vi "CPT Control 12.1.vi"() -> ()   [LabVIEW 2015]
uses:
  <vilib>/Analysis/baseanly.llb/Mean (DBL).vi
  <vilib>/Analysis/baseanly.llb/Normalize Vector.vi
  <vilib>/Utility/file.llb/Read From Spreadsheet File (string).vi
  <vilib>/Utility/file.llb/Write To Spreadsheet File (string).vi
  <vilib>/Utility/file.llb/Write To Spreadsheet File (DBL).vi
  <vilib>/Analysis/2dsp.llb/1D Cross Correlation (DBL).vi
  <vilib>/Utility/file.llb/Read Delimited Spreadsheet (DBL).vi
  <vilib>/Analysis/NI_AALBase.lvlib
  <vilib>/Analysis/NI_AALPro.lvlib
panel:
  out "Waveform Chart":dbl[](graph)
  in  "fre3":dbl
  out "Distance Difference Graph 2":dbl[](graph)
  out "Pore Offset:":dbl
  out "Side Offset:":dbl
  out "Axial Offset:":dbl
  in  "SET Pump Offsets":bool
  in  "Pore Offset SOLL":dbl
  in  "Side Offset Soll":dbl
  in  "Axial Offset Soll":dbl
  out "Stop Distance IS":dbl min=0.0 max=20.0 format="%#_f mm"
  in  "Stop Distance":dbl=20.0 min=0.0 max=20.0 format="%#_g mm"
  out "reset_flag":bool
  out "Time Loop":u32 format="%.0f ms"
  out "Pre-shearing output":dbl
  out "ms Offset":u32
  out "Test Flag":bool
  out "Date/Time:":string
  in  "Notaus":bool
  in  "Settings Tab":T1(tab)
  out "Axial Pressure":T2(graph)
  out "Side Pressure":T2(graph)
  out "Pore Pressure":T2(graph)
  in  "Visualize data":bool
  in  "Set":bool
  in  "maximum acceptable \nSide volume change (ml)":dbl
  in  "SET Pump Pressures":bool
  out "Porepressure":dbl format="%#_4f kPa"
  out "Axialpressure":dbl format="%#_4f kPa"
  out "Sidepressure":dbl format="%#_4f kPa"
  in  "Soll Pore Pressure":dbl min=-200.0 max=4900.0 format="%#_3f kPa"
  in  "Soll Axial Pressure":dbl min=-200.0 max=4000.0 format="%#_3f kPa"
  in  "Soll Side Pressure":dbl min=-200.0 max=4000.0 format="%#_3f kPa"
  in  "Activate Manuel Control":bool
  in  "Schieberegler":dbl(slide) min=-1.0 max=1.0 scale=1.0..-1.0
  out "Position Piston":dbl(slide)
  in  "Move":bool
  out "Contact?":bool
  out "Force Sensor":dbl format="%#_4g N"
  in  "Go - Seitendruck":bool
  in  "Go - Axialdruck":bool
  in  "Velocity Linear":dbl=200.0 format="%#_g kPa/Min"
  in  "Up_Lower":bool
  in  "Delta Pore":dbl format="%#_g kPa"
  in  "GO All Pressure":bool
  in  "Delta Seiten":dbl format="%#_g kPa"
  in  "Delta Axial":dbl format="%#_g kPa"
  in  "Go - Porendruck":bool
  out "Actual side volume change (ml)":sgl format="%.2f"
  out "Velocity deviation":T3(graph)
  out "Acceleration":T3(graph)
  in  "Finish test":bool
  in  "Set file":bool
  in  "Static peneration test":path
  in  "Vibro test 3":path
  in  "Vibro test 1":path
  in  "Static penetration Depth(mm) - 4":dbl
  in  "Time delay - 4":dbl
  in  "Enable Vibro Mode 2":bool
  in  "Enable Vibro Mode 3":bool
  in  "Depth(mm)3":dbl
  in  "Background velocity-3":dbl
  in  "Amplitdue-3":dbl
  in  "freq-3 ( Hz) 2":dbl
  in  "Time delay-3":dbl
  in  "Depth(mm)2":dbl
  in  "Background velocity-2":dbl
  in  "Amplitdue-2":dbl
  in  "freq-2 ( Hz)":dbl
  in  "Switch Vibro Mode":bool
  in  "Control start":bool
  in  "Control Stop":bool
  in  "Activate":bool
  out "Velocity vs Controller output":cluster{dbl[], dbl[]}[](graph)
  out "Correlation curve":dbl[](graph)
  out "time shift steps":sgl format="%.2f"
  in  "Visualize data":bool
  in  "Start Correlation":bool
  out "Intercept b":dbl
  out "Slope m":dbl
  in  "Time delay-2":dbl
  in  "Enable Vibro Mode 1":bool
  in  "Vibration frequency - 1  (Hz)":dbl
  in  "background velocity -1 (mm/s)":dbl
  in  "Amplitude - 1 (mm)":dbl
  in  "Vibro test 2":path
  in  "SET P/I Value":bool
  in  "Set auto file name":bool
  in  "SET Vibro Settings":bool
  out "Vibro Test IS":bool
  out "Frequency IS":dbl min=0.0 max=40.0 format="%#_g Hz"
  out "Amplitude IS":dbl=1.0 min=0.0 max=40.0 format="%#_g mm"
  out "Feeding IS":dbl min=0.0 max=20.0 format="%#_f mm/s"
  in  "New Path":string
  out "Path Logging":path
  in  "Set New Path":bool
  in  "VibroTest":bool=TRUE
  in  "Frequency SOLL":dbl=5.0 min=0.0 max=40.0 format="%#_g Hz"
  in  "Amplitude SOLL":dbl=3.0 min=0.0 max=40.0 format="%#_g mm"
  in  "Vorschub SOLL":dbl=20.0 min=0.0 max=20.0 format="%#_g mm/s"
  in  "Record Data":bool
  out "Record Flag":bool
  in  "start penetration":bool
  out "Boolean":bool
  in  "Soll I-Value":i32 min=-200 max=4000
  in  "Soll P-Value":i32 min=-200 max=4900
  out "IS I-Value":i32
  out "IS P-Value":i32
  out "Axial Pressure okay:":bool
  out "Side Pressure okay:":bool
  out "Pore Pressure okay:":bool
  in  "Circumference Control":bool
  in  "Turn off BC5":bool
  in  "SET Pre-Shearing":bool
  in  "Number of Cycles SOLL":dbl format="%#_f"
  in  "Duration of Cycle SOLL":i32
  in  "Amplitude Cycle SOLL":i32
  in  "Start Pre-Shearing":bool
  out "Pre-Shearing Ended Successful:":bool
  in  "Sollwert Porenwasser":dbl
  in  "Sollwert Seitendruck":dbl
  in  "Huang Su Calibration File":path
  out "IS Parameter 1":dbl=-163.9 format="%#_g x^6 +"
  out "IS Parameter 2":dbl=-163.9 format="%#_g x^5 +"
  out "IS Parameter 3":dbl=-163.9 format="%#_g x^4 +"
  out "IS Parameter 4":dbl=-163.9 format="%#_g x^3 +"
  out "IS Parameter 5":dbl=-163.9 format="%#_g x^2 +"
  out "IS Parameter 6":dbl=-163.9 format="%#_g x     +"
  out "IS Parameter 7":dbl=-163.9
  in  "SET Huang Su":bool
  in  "SOLL Parameter 1":dbl=-163.9 format="%#_g x^6 +"
  in  "SOLL Paramter 2":dbl=-163.9 format="%#_g x^5 +"
  in  "SOLL Parameter 3":dbl=-163.9 format="%#_g x^4 +"
  in  "SOLL Parameter 4":dbl=-163.9 format="%#_g x^3 +"
  in  "SOLL Parameter 5":dbl=-163.9 format="%#_g x^2 +"
  in  "SOLL Parameter 6":dbl=-163.9 format="%#_g x     +"
  in  "SOLL Parameter 7":dbl=-163.9
  out "Piston Position (mm)":dbl[](graph)
  out "Linear calibration":cluster{"array":dbl[], "array":dbl[]}(graph)
  in  "Calibration start":bool
  in  "Soll Slope-Strain":dbl
  in  "Soll Intercept-strain":dbl
  in  "Set button":bool
  out "IS-ADWIN":dbl
  out "IS- ADWIN":dbl
  in  "Initial cone position (mm)":dbl
  in  "Starting penetration depth (mm)  2":dbl
  in  "initial strain r0":dbl
  out "Timer Leackage":dbl format="%#_g s"
  out "Axial Leackage":dbl format="%.2f ml/m"
  out "Side Leackage":dbl format="%.2f ml/m"
  out "Pore Leackage":dbl format="%.2f ml/m"
  in  "Reset Leackage":bool
  out "Axial Kp:":dbl=40.0
  out "Axial Ki:":dbl format="%.2f"
  out "Side Kp:":dbl=40.0
  out "Side Ki:":dbl format="%.2f"
  out "Pore Kp:":dbl=40.0
  out "Pore Ki:":dbl format="%.2f"
  in  "SET Pump Controls":bool
  out "Modus":i32
  in  "Kpa":dbl=40.0
  in  "Kia":dbl=0.2 format="%.1f"
  in  "Kps":dbl=40.0
  in  "Kis":dbl=0.2 format="%.1f"
  in  "Kpp":dbl=40.0
  in  "Kip":dbl=0.2 format="%.1f"
  in  "Set":bool
  out "Side Offset: 2":dbl
  out "Axial Offset: 2":dbl
  out "Pore Offset: 2":dbl
  in  "Axial Offset Soll 2":dbl
  in  "Side Offset Soll 2":dbl
  in  "Pore Offset SOLL 2":dbl
  out "ms Offset Pre-Shearing":u32
  out "Seitendruck save":dbl format="%#.0f"
  out "Axialdruck save":dbl format="%#.0f"
  out "Porendruck save":dbl format="%#.0f"
  in  "View Tab":T4(tab)
  in  "Reset_left_graph":bool
  out "Recording":bool
  out "Cone Pressure":cluster{"mean":dbl, "mean":dbl}(graph)
  out "LVDT 3":dbl format="%0.3f mm"
  out "LVDT 2":dbl format="%0.3f mm"
  out "ml Pore Linear":dbl(slide) scale=0.0..1015.0
  out "ml Side Linear":dbl(slide) scale=0.0..1009.0
  out "ml Axial Linear":dbl(slide) scale=0.0..1014.5
  out "Pore":dbl format="%#_4g ml"
  out "Side":dbl format="%#_4g ml"
  out "Axial":dbl format="%#_4g ml"
  out "Addional Side Pressure":dbl format="%.2f kPa"
  out "Max Expansion":dbl format="%.2f mm"
  out "LVDT 1":dbl format="%0.3f mm"
  in  "Regelung Akiv Axial":bool
  in  "Regelung Akiv Sidepressure":bool
  in  "Regelung Akiv Porepress":bool
  out "Axial Pressure  [KPa]":dbl format="%#.2f kPa"
  out "Side Pressure  [KPa]":dbl format="%#.2f kPa"
  out "Pore Pressure [KPa]":dbl format="%#.2f kPa"
  out "ml Fontpanel":cluster{"mean":dbl, "mean":dbl, "mean":dbl}(graph)
  out "LVDT Frontpannel":cluster{"mean":dbl, "mean":dbl, "mean":dbl}(graph)
  out "Interner Kraftsensor [MPa]":cluster{"Y":dbl[], "Y":dbl[]}[](graph) caption="XY-Graph"
  out "Notaus Activ":bool
  out "Linear Control On":bool
  out "Test Started":bool
  out "Ready":bool
  out "Manuel Control":bool
  out "Pump Control On":bool
  out "Hold Position":bool
  out "Test ended":bool
  out "Penetration ongoing":bool
  out "Cone Tip Resistance":dbl format="%0.2f"
  out "Cone Side Resistance":dbl format="%0.2f"
  in  "Activate Pumps/Piston Controls":bool
  out "Distance Graph":T2(graph)
  out "Linear regression":cluster{dbl[], dbl[]}[](graph)
  out "Controller Output":T2(graph)
  out "Regelung Out":dbl(graph)
  out "Valve Is":dbl(graph)
  out "SOLL IS Distance":cluster{dbl, dbl}(graph)
  in  "Stop/Start":bool
  out "Axialdruck [Pa] 4":dbl(graph)
  out "Seitendruck [Pa] 3":dbl(graph)
  out "Porendruck [Pa] 2":dbl(graph)
  in  "Reset Alarm":bool
  out "Side Alarm":bool
  in  "Erlaubte Max Abweichung Side":dbl
  in  "Erlaubte  Max Abweichung Pore":dbl
  in  "Erlaubte Max Abweichung Axial":dbl
  out "Sollvorgabe":T5(graph)
  out "S":u32
  out "Total Elapsed Seconds":dbl
  out "Alarm Triggered":bool
  out "Abweichung Side":dbl format="%#_4g"
  out "Pore Alarm":bool
  out "Axial Alarm":bool
  out "Abweichung Pore":dbl format="%#_4g"
  out "Abweichung Axial":dbl format="%#_5g"
  # "Activate Manuel Piston Control"
  # "Velocity Piston"
  # "Up"
  # "Down"
  # "IS-ADwin:"
  # "Set Value:"
  # "Pore Pressure:"
  # "Side Pressure"
  # "Axial Pressure"
  # "Linear Pressure Control"
  # "Decreasing"
  # "Increasing"
  # "Delta Pore"
  # "Delta Side"
  # "Delta Axial"
  # "Vibro Settings"
  # "IS-ADwin:"
  # "Set Value:"
  # "Feeding:"
  # "Vibro Test ON:"
  # "Amplitude:"
  # "Frequency:"
  # "Controller Settings"
  # "IS-ADwin:"
  # "Set Value:"
  # "Kp:"
  # "Ki:"
  # "End of Test"
  # "IS-ADwin:"
  # "Set Value:"
  # "IS-ADwin:"
  # "Set Value:"
  # "Leackage Indicator"
  # "IS-ADwin:"
  # "Set Value:"
  # "Control"
  # "Pressure"
  # "reset"
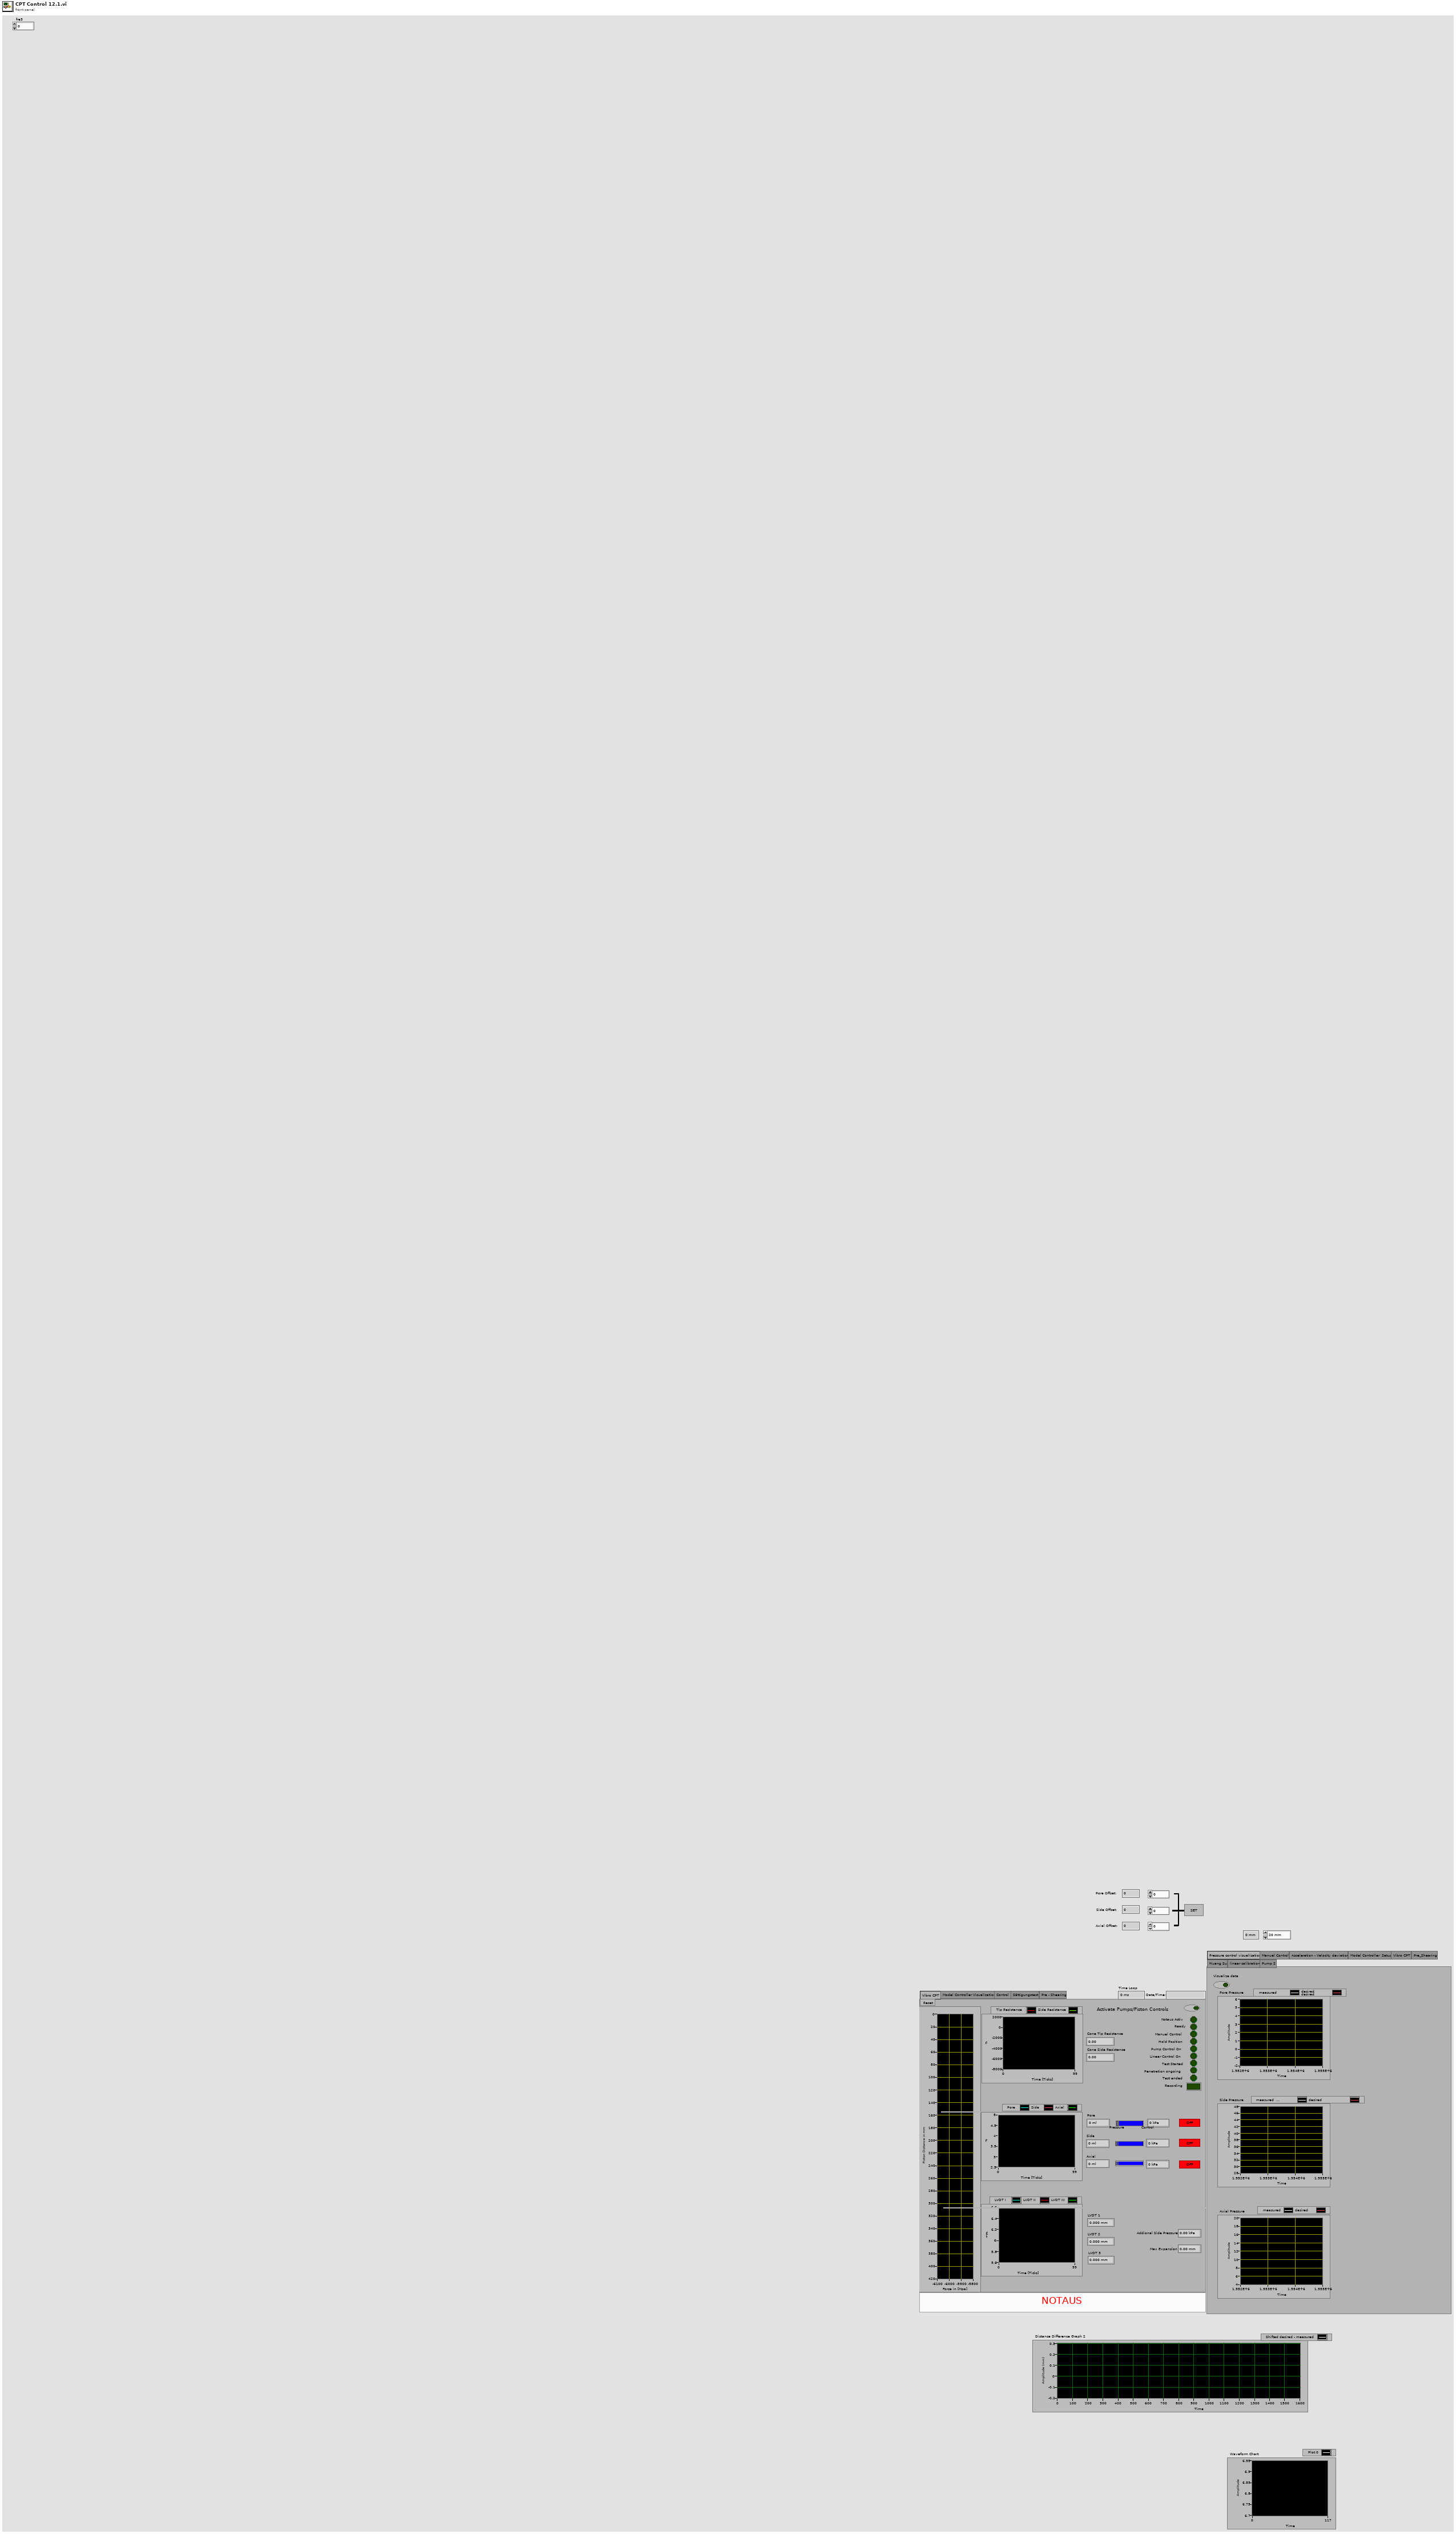
[diagram p1: front panel]
types:
  T1 = enum32{"Pressure control visualization", "Manuel Control", "Acceleration - Velocity deviation", "Model Controller  Setup", "Vibro CPT", "Pre_Shearing", "Huang Su", "linear calibration", "Pump S"}
  T2 = cluster{"Output Array":dbl[], "Output Array":dbl[]}[]
  T3 = cluster{"Output Array":dbl[], "Output Array 2":dbl[]}
  T4 = enum32{"Vibro CPT", "Model Controller Visualization", "Control", "Sättigungstest", "Pre - Shearing"}
  T5 = cluster{"Axial Pressure  [KPa]":dbl, "Pre-shearing output":dbl}
  T6 = enum8{"Enabled", "Disabled", "Disabled and Grayed Out"}
  T7 = enum16{"Program Counter", "Force ", "Position Induktiv", "Position Laser", "Laser 01", "Axial Stellwert", "LVDT 1", "LVDT 2", "LVDT 3", "Pore Pressure", "Side Pressure ", "Axial Pressure", "Pore Volumen", "Side Volumen ", "Axial Volumen ", "NaN", "LVDT Max", "Side Addtional Pressure", "Stellwert Regler", "Cone  Pore Pressure ", "Cone  Side Pressure ", "Valve Kolbenposition", "Regelanweichung", "Regelabweichung Summe ", ""}
  T8 = enum16{"Program Counter", "Force ", "Position Induktiv", "PorePress_regout", "SidePress_regout", "AxialPress_regout", "LVDT 1", "LVDT 2", "LVDT 3", "Pore Pressure", "Side Pressure ", "Axial Pressure", "Pore Volumen", "Side Volumen ", "Axial Volumen ", "Soll_Porepress", "Soll_Sidepress", "Soll_axialpress", "LVDT_max", "desired distance", "predict distance", "fitted velocity", "Valve IST", "Tip resistance", "Pore pressure", "Distance_Regout", "velocity data", "estimated_Distance_Regout", "normalize vel", "normalize Distance_regout", "strain", "additional side pressure", "initial_depth", "Distance_digital", "initial volume", "actual volume", "actual side volume"}
  T9 = enum16{"NaN", "WegInd_Digits", "Valve_IST", "KraftHTM_Digits", "WegInd_Delta", "WegLaser_Digits", "Laser_O1", "Laser_M3", "LVDT_2", "LVDT_3", "LVDT_1", "PorePress_Digits", "AxialPress_Digits", "SidePress_Digits", "SpindelA_Digits", "SpindelB_Digits", "SpindelC_Digits", "FPAR_17", "Slope_calibration", "Intercept_calibration", "PorePressOffset", "AxialPressOffset", "SidePressOffset", "FPAR_23", "FPAR_24", "Vorschub", "Sinusfrequenz_Vibro", "Amplitude_Vibro", "PreShearingOutput", "FPAR_29", "FPAR_30", "FPAR_31", "FPAR_32", "FPAR_33", "FPAR_34", "FPAR_35", "FPAR_36", "FPAR_37", "FPAR_38", "FPAR_39", "Kp_Porepress", "Ki_Porepress", "Kp_Sidepress", "Ki_Sidepress", "Kp_Axialpress", "Ki_Axialpress", "FPAR_46", "FPAR_47", "FPAR_48", "FPAR_49", "FPAR_50", "PaProMin", "FPAR_52", "FPAR_53", "FPAR_54", "Huang_Su_par_1", "Huang_Su_par_2", "Huang_Su_par_3", "Huang_Su_par_4", "Huang_Su_par_5", "FPAR_60", "FPAR_61", "Huang_Su_par_6", "Huang_Su_par_7", "FPAR_64", "FPAR_65", "FPAR_66", "Model_PreShearing", "Model_Vibro", "FPAR_69", "FPAR_70", "FPAR_71", "Set_Soll_PorePressure", "Set_Soll_AxialPressure", "Set_Soll_SidePressure", "Soll_PorePressure", "Soll_AxialPressure", "Soll_SidePressure", "Taktzeit", "Abtastfrequenz", "Clock"}
  T10 = enum16{"NaN", "WegInd_Digits", "Valve_IST", "KraftHTM_Digits", "WegInd_Delta", "WegLaser_Digits", "Laser_O1", "Laser_M3", "LVDT_2", "LVDT_3", "LVDT_1", "PorePress_Digits", "AxialPress_Digits", "SidePress_Digits", "SpindelA_Digits", "SpindelB_Digits", "SpindelC_Digits", "FPAR_17", "FPAR_18", "FPAR_19", "PorePressOffset", "AxialPressOffset", "SidePressOffset", "FPAR_23", "FPAR_24", "Vorschub", "Sinusfrequenz_Vibro", "Amplitude_Vibro", "PreShearingOutput", "FPAR_29", "FPAR_30", "FPAR_31", "FPAR_32", "FPAR_33", "FPAR_34", "FPAR_35", "FPAR_36", "FPAR_37", "FPAR_38", "FPAR_39", "Kp_Porepress", "Ki_Porepress", "Kp_Sidepress", "Ki_Sidepress", "Kp_Axialpress", "Ki_Axialpress", "FPAR_46", "FPAR_47", "FPAR_48", "FPAR_49", "FPAR_50", "PaProMin", "FPAR_52", "FPAR_53", "FPAR_54", "Huang_Su_par_1", "Huang_Su_par_2", "Huang_Su_par_3", "Huang_Su_par_4", "Huang_Su_par_5", "FPAR_60", "FPAR_61", "Huang_Su_par_6", "Huang_Su_par_7", "FPAR_64", "FPAR_65", "FPAR_66", "Model_PreShearing", "Model_Vibro", "FPAR_69", "FPAR_70", "FPAR_71", "Set_Soll_PorePressure", "Set_Soll_AxialPressure", "Set_Soll_SidePressure", "Soll_PorePressure", "Soll_AxialPressure", "Soll_SidePressure", "Taktzeit", "Abtastfrequenz", "Clock"}
  T11 = cluster{"Output Array":dbl[], "Output Array":dbl[]}
  T12 = cluster{"Output Array":dbl[], "normalized waveform":waveform(dbl)}
  T13 = cluster{"Output Array":dbl[], "normalized waveform":waveform(dbl)}[]
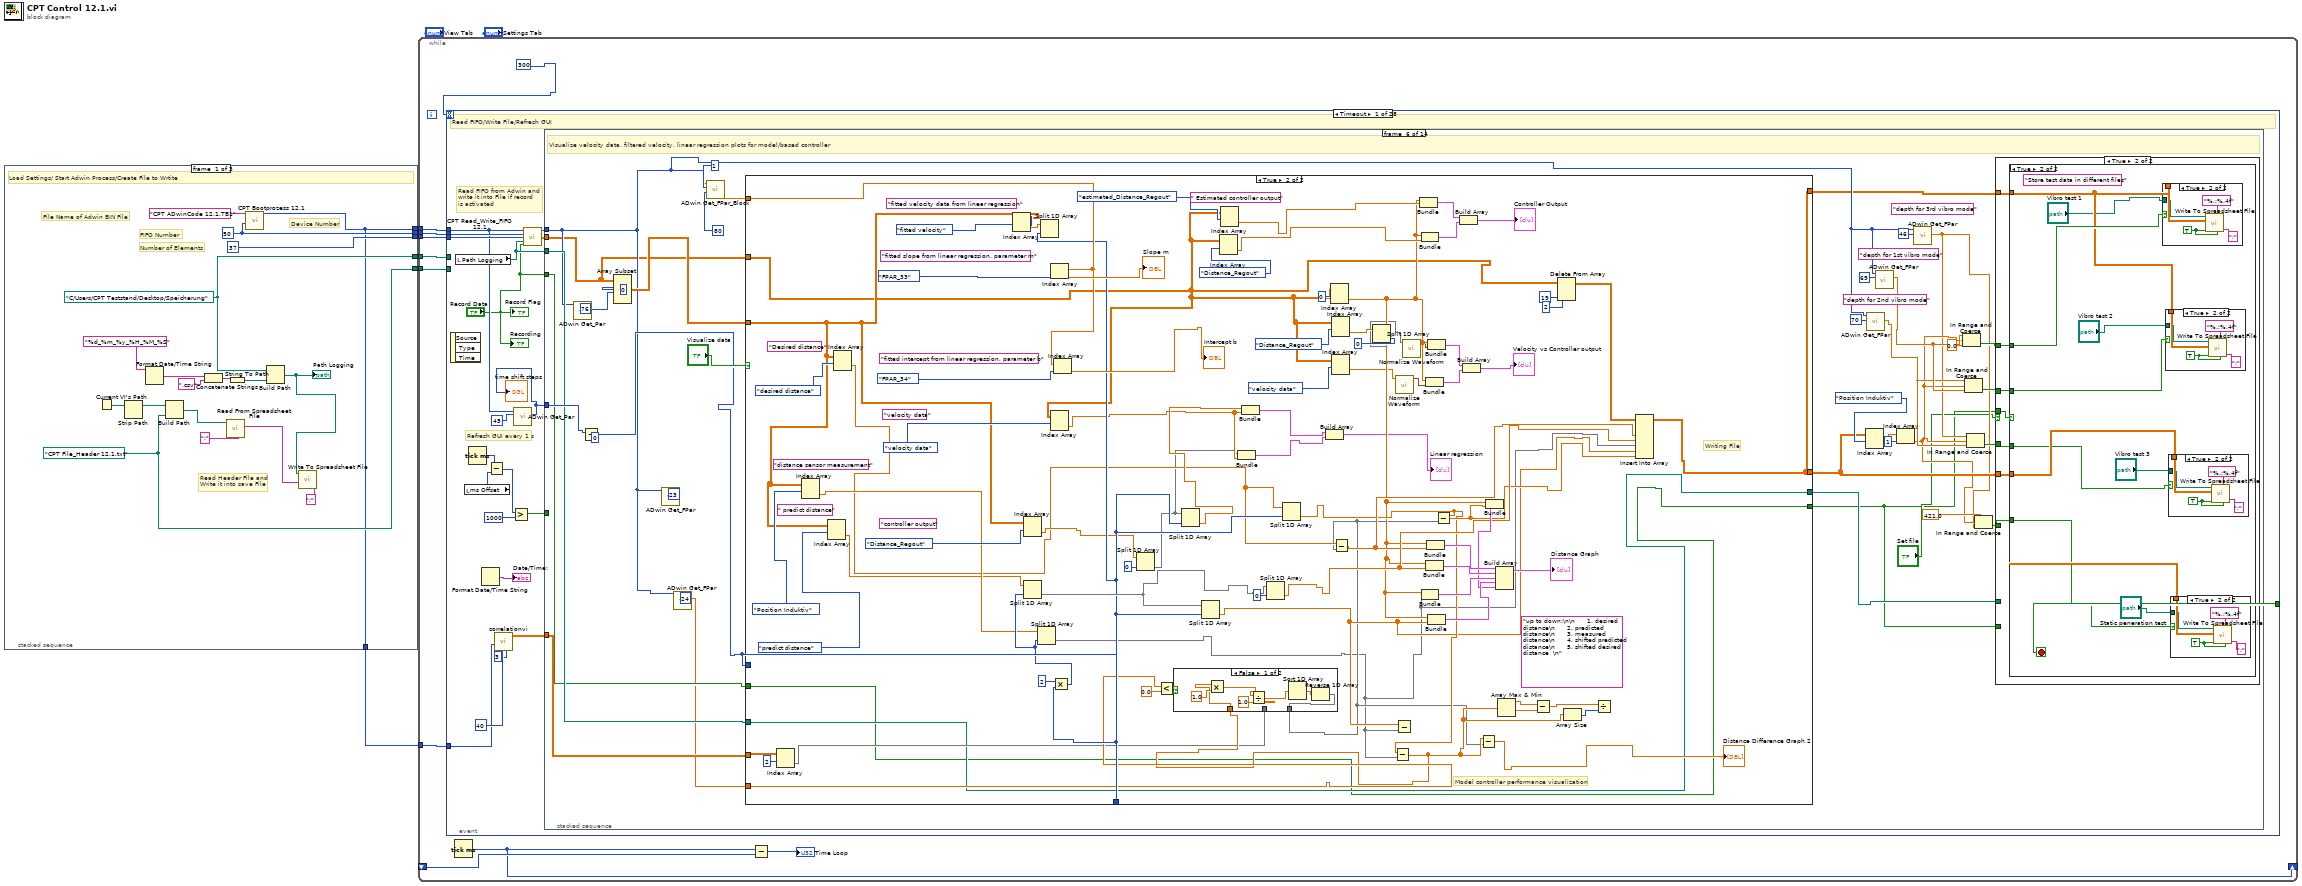
[diagram p0: block diagram]
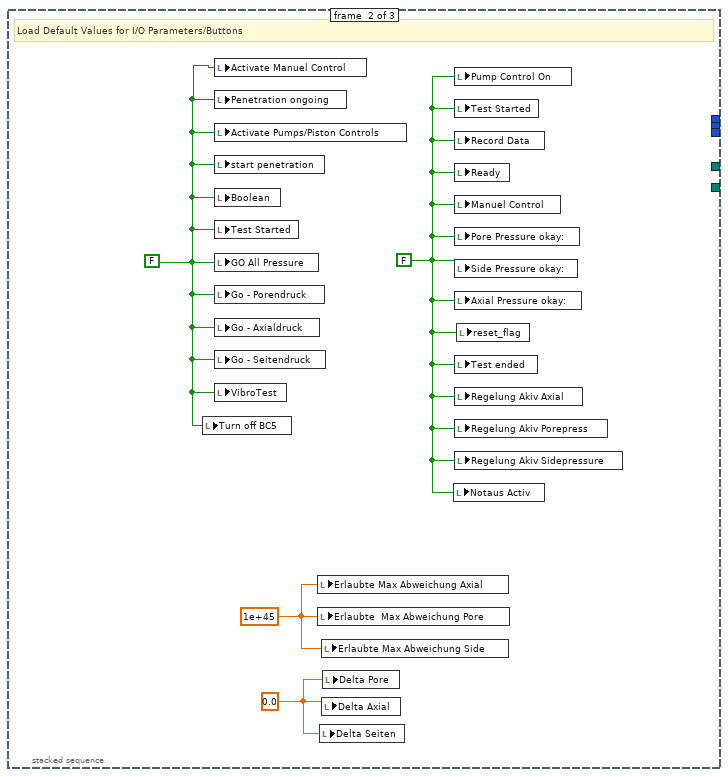
[diagram p2: hidden frame]
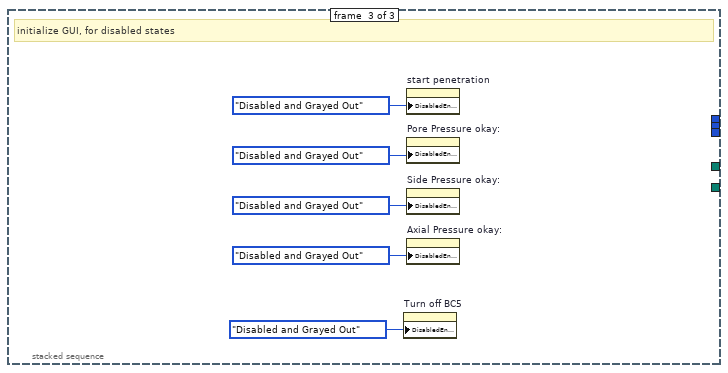
[diagram p3: hidden frame]
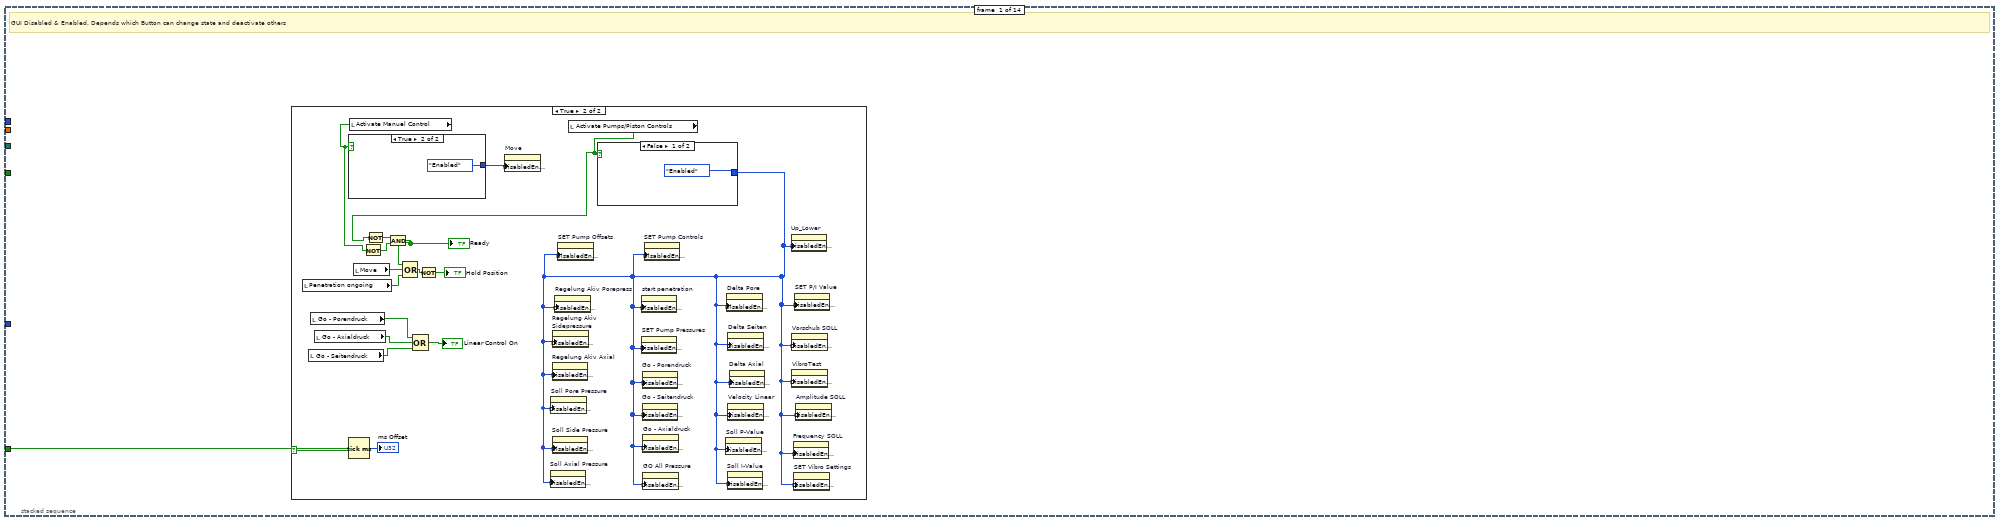
[diagram p4: hidden frame]
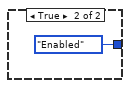
[diagram p6: hidden frame]
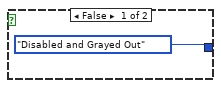
[diagram p7: hidden frame]
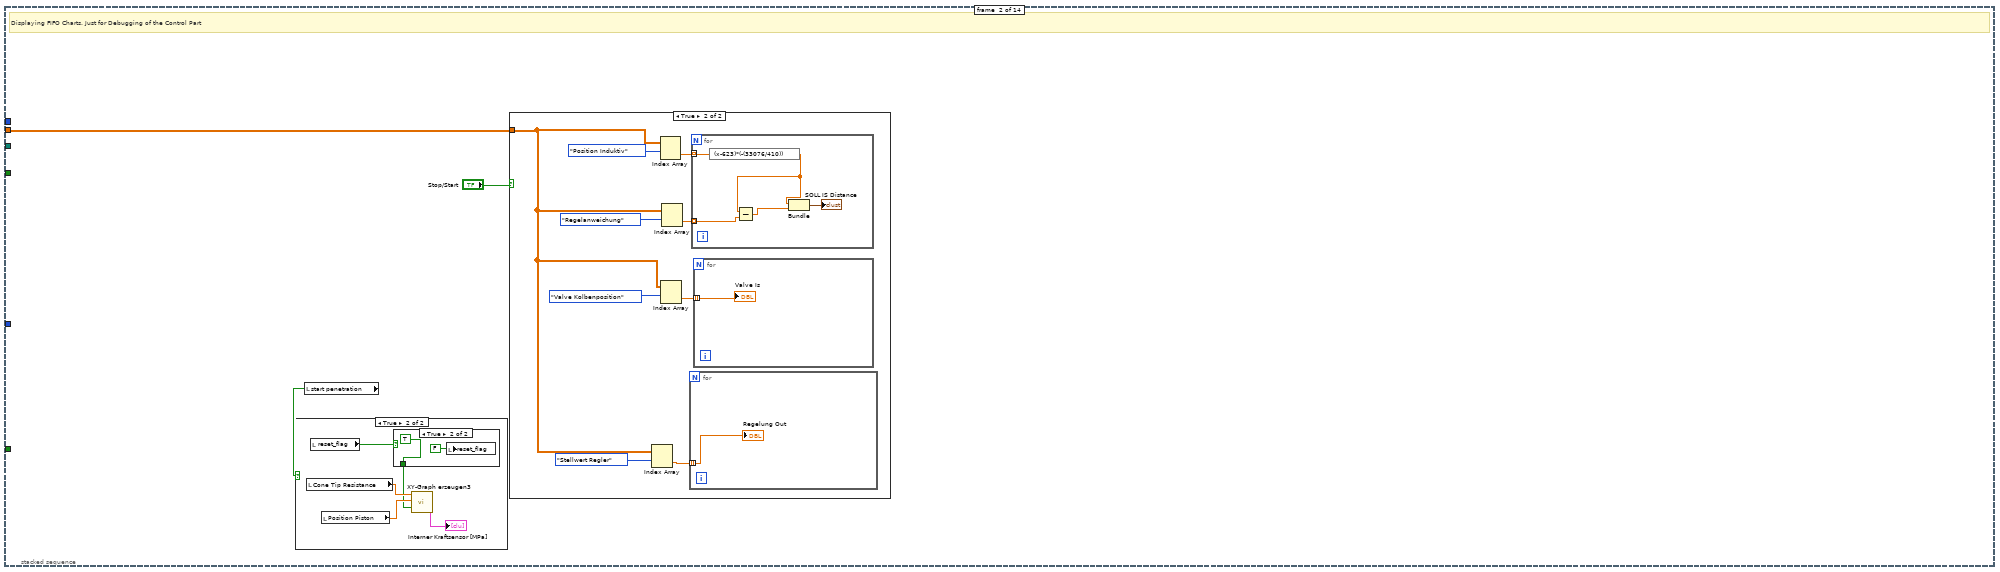
[diagram p8: hidden frame]
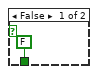
[diagram p10: hidden frame]
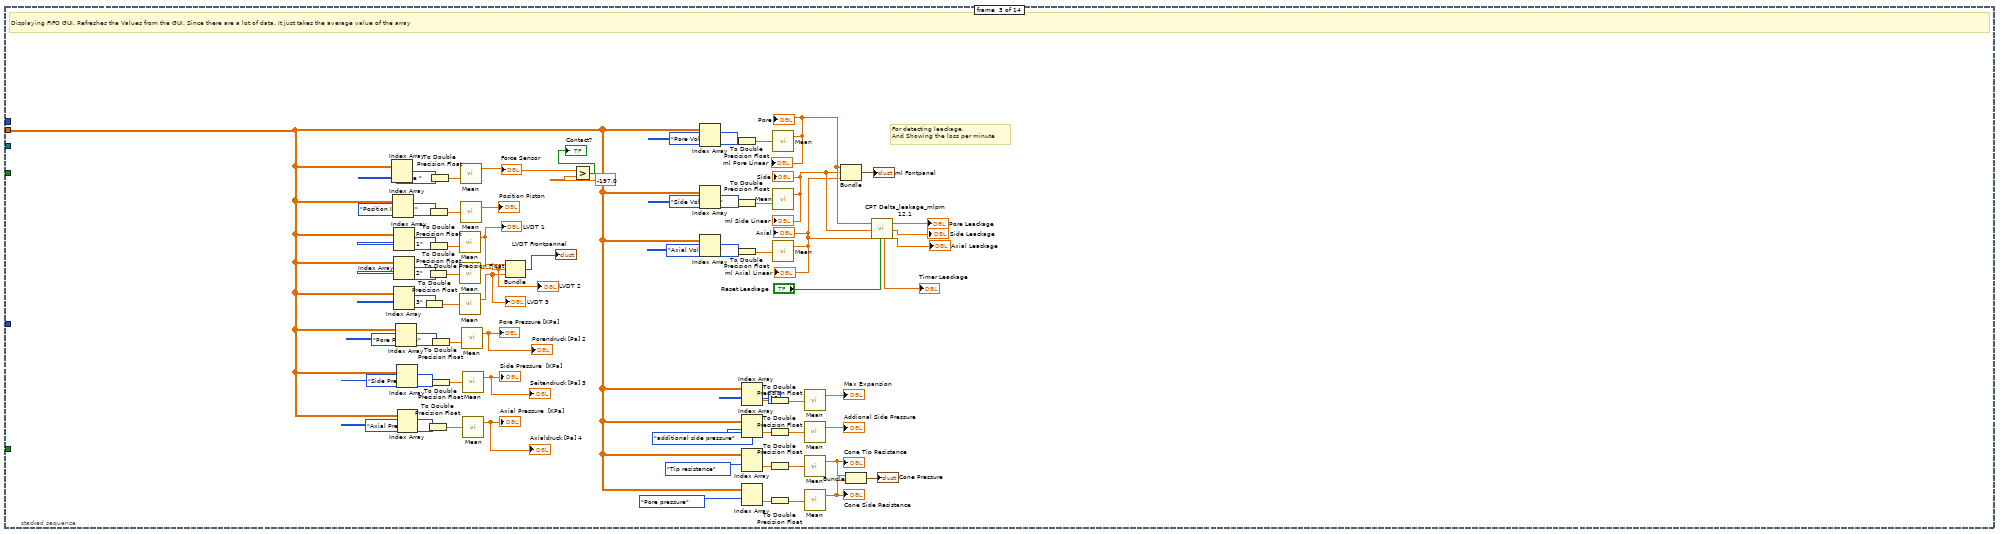
[diagram p12: hidden frame]
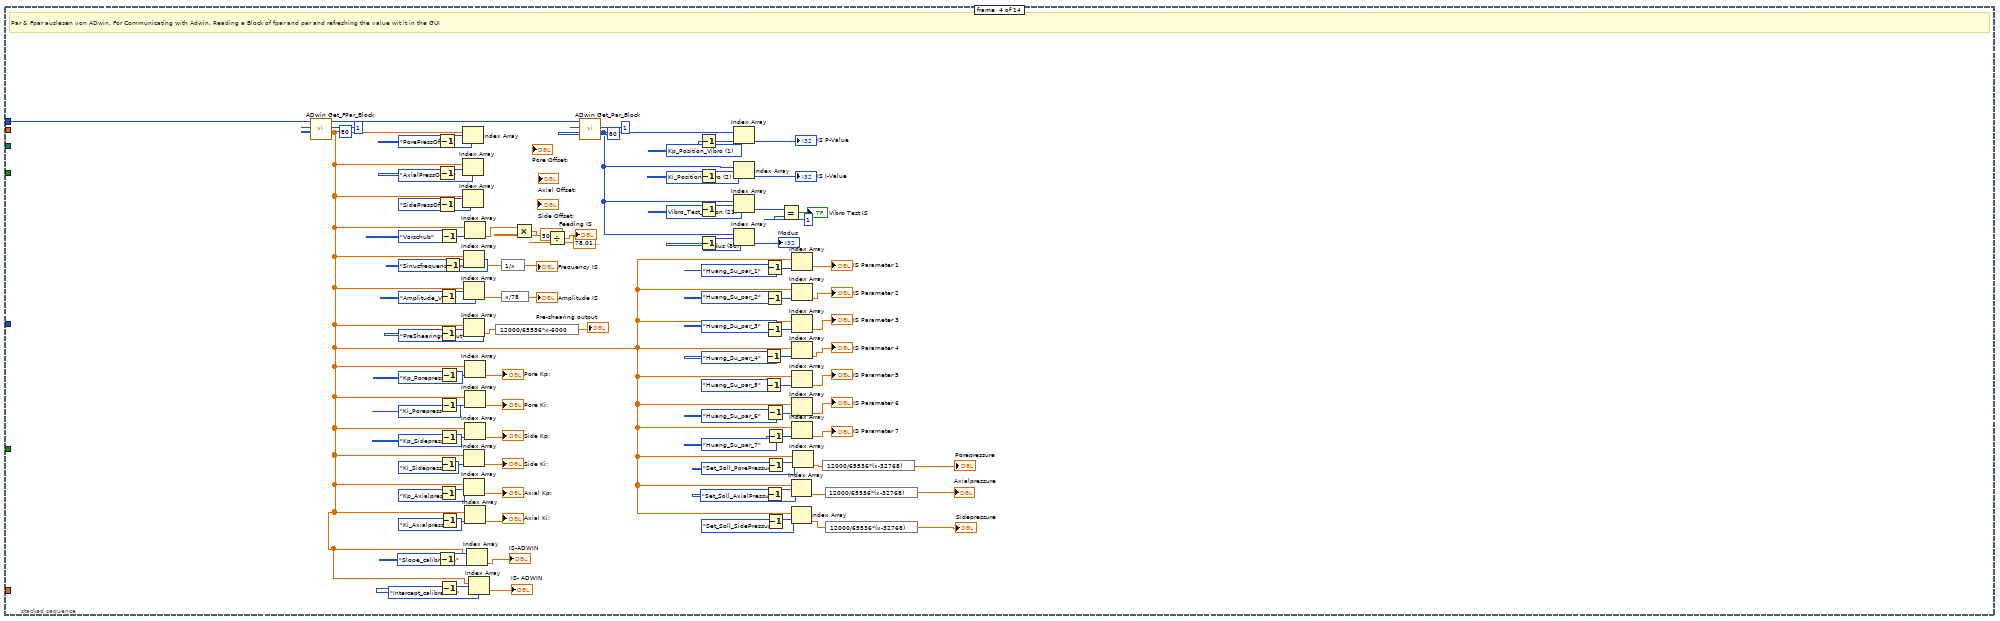
[diagram p13: hidden frame]
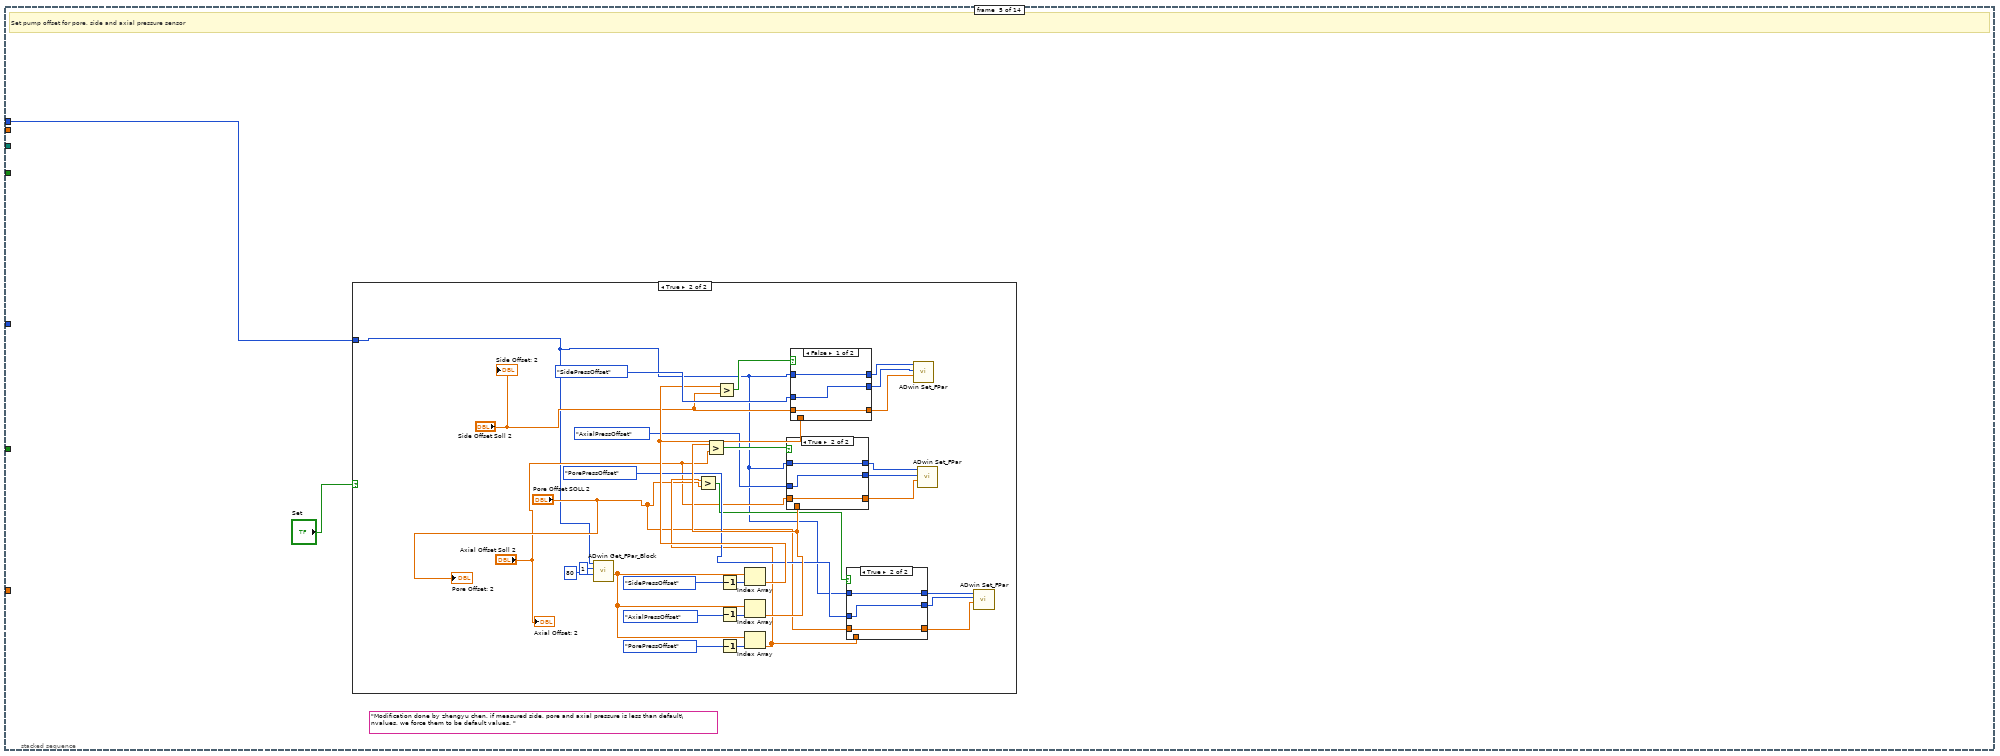
[diagram p14: hidden frame]
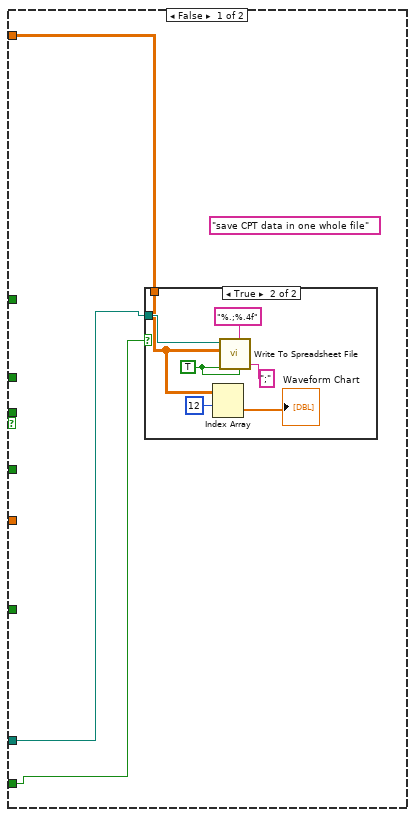
[diagram p19: hidden frame]
diagram:
  n1 = stacked-sequence {
    tunnel: [w7 _ _] -> w6
    tunnel: [w24 _ _] -> w5
    tunnel: [37 ("dimension size") _ _] -> w4
    tunnel: [w11 _ _] -> w3
    tunnel: [w9 _ _] -> w2
    tunnel: [w7 _ _] -> w1
    frame #0 {
      w9 = path "CPT File_Header 12.1.txt" ("Grundpfad")
      w24 = u16 50 ("FifoNo")
      w11 = path "C:/Users/CPT Teststand/Desktop/Speicherung" ("Grundpfad")
      # "Read Header File and \nWrite it into save File"
      # "File Name of Adwin BIN File"
      # "Device Number"
      # "Number of Elements"
      # "FIFO Number"
      # "Load Settings/ Start Adwin Process/Create File to Wrtite"
      n2 = Current VI's Path() -> (path=w14:path)
      n3 = Strip Path(path=w14) -> (stripped path=w13:path)  [unwired: 1 out]
      n4 = Format Date/Time String(time format string (%c)="%d_%m_%y_%H_%M_%S") -> (date/time string=w18:string)  [unwired: 2 in]
      n5 = Build Path(base path=w13, name or relative path=w9) -> (appended path=w15:path)
      n6 = Concatenate Strings(w18, ".csv" ("String")) -> (w21:string)
      n7 = call-poly <vilib>:"Read From Spreadsheet File.vi"("delimiter (\\t)"=";" ("delimiter (\\t)"), "file path (dialog if empty)"=w15) -> ("first row"=w16:string[])  [unwired: 5 in, 4 out]
      n8 = String To Path(string=w21) -> (path=w20:path)
      n9 = call "CPT Bootprozess 12.1.vi"("FifoNo"=w24, "Boot File Relative Referenz"="CPT ADwinCode 12.1.TB1" ("Filename")) -> ("Device No. out"=w7:u16)  [unwired: 8 in, 1 out]
      n10 = Build Path(base path=w11, name or relative path=w20) -> (appended path=w8:path)
      "Path Logging" <- w8
      n11 = call-poly <vilib>:"Write To Spreadsheet File.vi"("delimiter (\\t)"=";" ("delimiter (\\t)"), "1D data"=w16, "file path (dialog if empty)"=w8) -> ()  [unwired: 5 in, 1 out]
    }
    frame #1 {
      w26 = 1e+45 ("Abweichung Solll  - Ist")
      w27 = 0.0 ("Delta Pore")
      w28 = FALSE ("Boolean")
      w25 = FALSE ("Freeze")
      # "Load Default Values for I/O Parameters/Buttons"
      n12 = local write "Turn off BC5"(w28) -> ()
      n13 = local write "Activate Manuel Control"(w28) -> ()
      n14 = local write "Penetration ongoing"(w28) -> ()
      n15 = local write "Activate Pumps/Piston Controls"(w28) -> ()
      n16 = local write "start penetration"(w28) -> ()
      n17 = local write "Boolean"(w28) -> ()
      n18 = local write "Test Started"(w28) -> ()
      n19 = local write "GO All Pressure"(w28) -> ()
      n20 = local write "Go - Porendruck"(w28) -> ()
      n21 = local write "Go - Axialdruck"(w28) -> ()
      n22 = local write "Go - Seitendruck"(w28) -> ()
      n23 = local write "VibroTest"(w28) -> ()
      n24 = local write "Erlaubte Max Abweichung Axial"(w26) -> ()
      n25 = local write "Erlaubte  Max Abweichung Pore"(w26) -> ()
      n26 = local write "Delta Seiten"(w27) -> ()
      n27 = local write "Erlaubte Max Abweichung Side"(w26) -> ()
      n28 = local write "Delta Axial"(w27) -> ()
      n29 = local write "Delta Pore"(w27) -> ()
      n30 = local write "Notaus Activ"(w25) -> ()
      n31 = local write "Pump Control On"(w25) -> ()
      n32 = local write "Test Started"(w25) -> ()
      n33 = local write "Record Data"(w25) -> ()
      n34 = local write "Ready"(w25) -> ()
      n35 = local write "Manuel Control"(w25) -> ()
      n36 = local write "Pore Pressure okay:"(w25) -> ()
      n37 = local write "Side Pressure okay:"(w25) -> ()
      n38 = local write "Axial Pressure okay:"(w25) -> ()
      n39 = local write "Test ended"(w25) -> ()
      n40 = local write "Regelung Akiv Axial"(w25) -> ()
      n41 = local write "Regelung Akiv Porepress"(w25) -> ()
      n42 = local write "Regelung Akiv Sidepressure"(w25) -> ()
      n43 = local write "reset_flag"(w25) -> ()
    }
    frame #2 {
      # "initialize GUI, for disabled states"
      n44 = property on="Turn off BC5" class="Bool (strict)"("DisabledEnum"=T6."Disabled and Grayed Out" ("Disabled")) -> ()  [unwired: 2 in, 2 out]
      n45 = property on="start penetration" class="Bool (strict)"("DisabledEnum"=T6."Disabled and Grayed Out" ("Disabled")) -> ()  [unwired: 2 in, 2 out]
      n46 = property on="Pore Pressure okay:" class="Bool (strict)"("DisabledEnum"=T6."Disabled and Grayed Out" ("Disabled")) -> ()  [unwired: 2 in, 2 out]
      n47 = property on="Side Pressure okay:" class="Bool (strict)"("DisabledEnum"=T6."Disabled and Grayed Out" ("Disabled")) -> ()  [unwired: 2 in, 2 out]
      n48 = property on="Axial Pressure okay:" class="Bool (strict)"("DisabledEnum"=T6."Disabled and Grayed Out" ("Disabled")) -> ()  [unwired: 2 in, 2 out]
    }
  }
  n49 = while {
    tunnel: w6 -> [w35]
    shift-right: [w42] -> _
    shift-left: _ -> [w44]
    tunnel: w5 -> [w41]
    tunnel: w4 -> [w40]
    tunnel: w3 -> [w39]
    tunnel: w2 -> [w37]
    tunnel: w1 -> [w36]
    stop <- w38 stop-if-true
    n50 = event shown="[0] Timeout" {
      selector: _ -> [_ _ _ _ _ _ _ _ _ _ _ _ _ _ _ _ _ _ _ _ _ _ _ _ _ _ _ _]
      dyn-events: _ -> [_ _ _ _ _ _ _ _ _ _ _ _ _ _ _ _ _ _ _ _ _ _ _ _ _ _ _ _]
      timeout: 300 -> [_ _ _ _ _ _ _ _ _ _ _ _ _ _ _ _ _ _ _ _ _ _ _ _ _ _ _ _]
      tunnel: w35 -> [w52 _ w928 w934 w986 w999 w1004 w1013 w1020 _ w1073 w1109 w1120 _ w1194 _ w1221 w1229 w1243 w1247 w1257 w1267 w1275 w1292 w1332 w1355 w1365 w1410]
      tunnel: w41 -> [w63 _ _ _ _ _ _ _ _ _ _ _ _ _ _ _ _ _ _ _ _ _ _ _ _ _ _ _]
      tunnel: w40 -> [w62 _ _ _ _ _ _ _ _ _ _ _ _ _ _ _ _ _ _ _ _ _ _ _ _ _ _ _]
      tunnel: w39 -> [_ _ _ _ _ _ _ _ _ _ _ _ _ w1164 _ w1203 _ _ _ _ _ _ _ _ _ _ _ _]
      tunnel: [_ _ w930 _ _ _ _ _ _ _ _ _ _ _ _ _ _ _ _ _ _ _ _ _ _ _ _ _] -> w38
      tunnel: w37 -> [_ _ _ _ _ _ _ _ _ _ _ _ _ w1156 _ w1196 _ _ _ _ _ _ _ _ _ _ _ _]
      tunnel: w36 -> [w47 _ _ _ _ _ _ _ _ _ _ _ _ _ _ _ _ _ _ _ _ _ _ _ _ _ _ _]
      event Timeout {
        # "Read FIFO from Adwin and \nwrite it into File if record \nis activated"
        # "Refresh GUI every 1 s"
        # "Read FIFO/Write File/Refresh GUI"
        n51 = event-data() -> ()  [unwired: 1 in, 3 out]
        n52 = local read "Path Logging"() -> (w46:path)
        n53 = local read "ms Offset"() -> (w59:u32)
        n54 = Tick Count (ms)() -> (millisecond timer value=w58:u32)
        n55 = Format Date/Time String() -> (date/time string=→"Date/Time:":string)  [unwired: 3 in]
        n56 = Subtract(x=w58, y=w59) -> (x-y=w56:u32)
        n57 = call "correlationvi.vi"("Number of Elements"=3, "FifoNo"=i16 40, "Device No."=w47) -> ("Output Array 2"=w48:dbl[][])  [unwired: 6 in, 2 out]
        n58 = Greater?(x=w56, y=u32 1000) -> (0:w57:bool)
        n59 = call "ADwin Get_Par.vi"("index"=u16 45 ("Device No. out"), "Device No. (1)"=w52) -> ("ParameterValue"=w51:i32)  [unwired: 7 in, 2 out]
        "time shift steps" <- w51
        n60 = call "CPT Read_Write_FIFO 12.1.vi"("Device No."=w52, "FifoNo"=w63, "Number of Elements"=w62, "Path Logging"=w46, "Record"="Record Data") -> ("Device No. out"=w60:u16, "Output Array"=w61:dbl[][])  [unwired: 9 in]
        n61 = stacked-sequence {
          tunnel: w61 -> [_ w87 w127 _ _ w338 w524 w577 w617 _ w739 _ _ _]
          tunnel: w60 -> [_ _ _ w273 w287 w353 w522 _ w610 w734 w742 w766 _ w900]
          tunnel: w57 -> [w64 _ _ _ _ _ _ _ _ _ _ _ _ _]
          tunnel: w51 -> [_ _ _ _ _ w368 _ _ w616 _ _ _ _ _]
          tunnel: w48 -> [_ _ _ _ _ w363 w528 _ _ _ _ _ _ _]
          tunnel: w46 -> [_ _ _ _ _ w366 _ _ _ _ _ _ _ _]
          tunnel: "Record Data" -> [_ _ _ _ _ w365 _ _ _ _ _ _ _ _]
          frame #0 {
            # "GUI Disabled & Enabled. Depends which Button can change state and deactivate others"
            n62 = case shown="True" w64 {
              frame False {
              }
              frame True {
                n63 = local read "Penetration ongoing"() -> (w77:bool)
                n64 = local read "Go - Seitendruck"() -> (w73:bool)
                n65 = local read "Go - Porendruck"() -> (w71:bool)
                n66 = local read "Go - Axialdruck"() -> (w72:bool)
                n67 = Tick Count (ms)() -> (millisecond timer value=→"ms Offset":u32)
                n68 = local read "Activate Manuel Control"() -> (w69:bool)
                n69 = case shown="True" w69 {
                  tunnel: [T6."Disabled and Grayed Out" ("Disabled") T6."Enabled" ("Disabled")] -> w80
                  frame False {
                  }
                  frame True {
                  }
                }
                n70 = local read "Move"() -> (w78:bool)
                n71 = Not(x=w69) -> (.not. x?=w67:bool)
                n72 = Compound Arithmetic op=OR(w71, w72, w73) -> (→"Linear Control On":bool)
                n73 = property on="Move" class="Bool (strict)"("DisabledEnum"=w80) -> ()  [unwired: 2 in, 2 out]
                n74 = local read "Activate Pumps/Piston Controls"() -> (w70:bool)
                n75 = Not(x=w70) -> (.not. x?=w68:bool)
                n76 = And(x=w68, y=w67) -> (x .and. y?=w66:bool)
                "Ready" <- w66
                n77 = Compound Arithmetic op=OR(w66, w78, w77) -> (w76:bool)
                n78 = Not(x=w76) -> (.not. x?=→"Hold Position":bool)
                n79 = case shown="False" w70 {
                  tunnel: [T6."Enabled" ("Disabled") T6."Enabled" ("Disabled")] -> w65
                  frame False {
                  }
                  frame True {
                  }
                }
                n80 = property on="Soll Axial Pressure" class="DigNum (strict)"("DisabledEnum"=w65) -> ()  [unwired: 2 in, 2 out]
                n81 = property on="Soll Pore Pressure" class="DigNum (strict)"("DisabledEnum"=w65) -> ()  [unwired: 2 in, 2 out]
                n82 = property on="Regelung Akiv Axial" class="Bool (strict)"("DisabledEnum"=w65) -> ()  [unwired: 2 in, 2 out]
                n83 = property on="Soll Side Pressure" class="DigNum (strict)"("DisabledEnum"=w65) -> ()  [unwired: 2 in, 2 out]
                n84 = property on="Regelung Akiv Sidepressure" class="Bool (strict)"("DisabledEnum"=w65) -> ()  [unwired: 2 in, 2 out]
                n85 = property on="Regelung Akiv Porepress" class="Bool (strict)"("DisabledEnum"=w65) -> ()  [unwired: 2 in, 2 out]
                n86 = property on="SET Pump Offsets" class="Bool"("DisabledEnum"=w65) -> ()  [unwired: 2 in, 2 out]
                n87 = property on="start penetration" class="Bool (strict)"("DisabledEnum"=w65) -> ()  [unwired: 2 in, 2 out]
                n88 = property on="SET Pump Pressures" class="Bool"("DisabledEnum"=w65) -> ()  [unwired: 2 in, 2 out]
                n89 = property on="Go - Porendruck" class="Bool (strict)"("DisabledEnum"=w65) -> ()  [unwired: 2 in, 2 out]
                n90 = property on="Go - Seitendruck" class="Bool (strict)"("DisabledEnum"=w65) -> ()  [unwired: 2 in, 2 out]
                n91 = property on="Go - Axialdruck" class="Bool (strict)"("DisabledEnum"=w65) -> ()  [unwired: 2 in, 2 out]
                n92 = property on="GO All Pressure" class="Bool (strict)"("DisabledEnum"=w65) -> ()  [unwired: 2 in, 2 out]
                n93 = property on="SET Pump Controls" class="Bool"("DisabledEnum"=w65) -> ()  [unwired: 2 in, 2 out]
                n94 = property on="Soll P-Value" class="DigNum (strict)"("DisabledEnum"=w65) -> ()  [unwired: 2 in, 2 out]
                n95 = property on="Delta Pore" class="DigNum (strict)"("DisabledEnum"=w65) -> ()  [unwired: 2 in, 2 out]
                n96 = property on="Soll I-Value" class="DigNum (strict)"("DisabledEnum"=w65) -> ()  [unwired: 2 in, 2 out]
                n97 = property on="Delta Seiten" class="DigNum (strict)"("DisabledEnum"=w65) -> ()  [unwired: 2 in, 2 out]
                n98 = property on="Velocity Linear" class="DigNum (strict)"("DisabledEnum"=w65) -> ()  [unwired: 2 in, 2 out]
                n99 = property on="Delta Axial" class="DigNum (strict)"("DisabledEnum"=w65) -> ()  [unwired: 2 in, 2 out]
                n100 = property on="Up_Lower" class="Bool (strict)"("DisabledEnum"=w65) -> ()  [unwired: 2 in, 2 out]
                n101 = property on="Vorschub SOLL" class="DigNum (strict)"("DisabledEnum"=w65) -> ()  [unwired: 2 in, 2 out]
                n102 = property on="VibroTest" class="Bool (strict)"("DisabledEnum"=w65) -> ()  [unwired: 2 in, 2 out]
                n103 = property on="Frequency SOLL" class="DigNum (strict)"("DisabledEnum"=w65) -> ()  [unwired: 2 in, 2 out]
                n104 = property on="SET Vibro Settings" class="Bool"("DisabledEnum"=w65) -> ()  [unwired: 2 in, 2 out]
                n105 = property on="SET P/I Value" class="Bool"("DisabledEnum"=w65) -> ()  [unwired: 2 in, 2 out]
                n106 = property on="Amplitude SOLL" class="DigNum (strict)"("DisabledEnum"=w65) -> ()  [unwired: 2 in, 2 out]
              }
            }
          }
          frame #1 {
            # "Displaying FIFO Charts. Just for Debugging of the Control Part"
            n107 = local read "start penetration"() -> (w85:bool)
            n108 = case shown="True" w85 {
              frame False {
              }
              frame True {
                n109 = local read "Cone Tip Resistance"() -> (w90:dbl)
                n110 = local read "reset_flag"() -> (w89:bool)
                n111 = local read "Position Piston"() -> (w91:dbl)
                n112 = case shown="True" w89 {
                  tunnel: [FALSE ("Reset") TRUE ("Reset")] -> w88
                  frame False {
                  }
                  frame True {
                    n113 = local write "reset_flag"(FALSE ("reset_flag")) -> ()
                  }
                }
                n114 = call "XY-Graph erzeugen3"("Reset"=w88, "Y Input"=w91, "X Input"=w90) -> ("XY Graph"=→"Interner Kraftsensor [MPa]":cluster{"Y":dbl[], "Y":dbl[]}[])  [unwired: 7 in, 1 out]
              }
            }
            n115 = case shown="True" "Stop/Start" {
              tunnel: w87 -> [_ w101]
              frame False {
              }
              frame True {
                n116 = Index Array(array=w101, index (row)=T7."Stellwert Regler" ("Enum")) -> (element=w96:dbl[])  [unwired: 1 in]
                n117 = Index Array(array=w101, index (row)=T7."Position Induktiv" ("Enum")) -> (element=w104:dbl[])  [unwired: 1 in]
                n118 = Index Array(array=w101, index (row)=T7."Valve Kolbenposition" ("Enum")) -> (element=w102:dbl[])  [unwired: 1 in]
                n119 = Index Array(array=w101, index (row)=T7."Regelanweichung" ("Enum")) -> (element=w103:dbl[])  [unwired: 1 in]
                n120 = for {
                  tunnel: w96 -> [w105] mode=indexing
                  "Regelung Out" <- w105
                }
                n121 = for {
                  tunnel: w104 -> [w110] mode=indexing
                  tunnel: w103 -> [w107] mode=indexing
                  n122 = expression code="(x-623)*(-(33076/410))"(w110) -> (w109:dbl)
                  n123 = Subtract(x=w109, y=w107) -> (x-y=w108:dbl)
                  n124 = Bundle(w109, w108) -> (→"SOLL IS Distance":cluster{dbl, dbl})  [unwired: 1 in]
                }
                n125 = for {
                  tunnel: w102 -> [w106] mode=indexing
                  "Valve Is" <- w106
                }
              }
            }
          }
          frame #2 {
            # "For detecting leackage. \nAnd Showing the loss per minute"
            # "Displaying FIFO GUI. Refreshes the Values from the GUI. Since there are a lot of data. It just takes the average value of the array"
            n126 = Index Array(array=w127, index (row)=T7."Force " ("Enum")) -> (element=w173:dbl[])  [unwired: 1 in]
            n127 = Index Array(array=w127, index (row)=T7."Position Induktiv" ("Enum")) -> (element=w174:dbl[])  [unwired: 1 in]
            n128 = Index Array(array=w127, index (row)=T7."LVDT 1" ("Enum")) -> (element=w179:dbl[])  [unwired: 1 in]
            n129 = Index Array(array=w127, index (row)=T7."LVDT 2" ("Enum")) -> (element=w180:dbl[])  [unwired: 1 in]
            n130 = Index Array(array=w127, index (row)=T7."LVDT 3" ("Enum")) -> (element=w181:dbl[])  [unwired: 1 in]
            n131 = Index Array(array=w127, index (row)=T7."Pore Pressure" ("Enum")) -> (element=w164:dbl[])  [unwired: 1 in]
            n132 = Index Array(array=w127, index (row)=T7."Side Pressure " ("Enum")) -> (element=w165:dbl[])  [unwired: 1 in]
            n133 = Index Array(array=w127, index (row)=T7."Axial Pressure" ("Enum")) -> (element=w166:dbl[])  [unwired: 1 in]
            n134 = To Double Precision Float(number=w181) -> (double precision float=w178:dbl[])
            n135 = To Double Precision Float(number=w166) -> (double precision float=w163:dbl[])
            n136 = To Double Precision Float(number=w180) -> (double precision float=w176:dbl[])
            n137 = To Double Precision Float(number=w174) -> (double precision float=w169:dbl[])
            n138 = To Double Precision Float(number=w179) -> (double precision float=w177:dbl[])
            n139 = To Double Precision Float(number=w173) -> (double precision float=w170:dbl[])
            n140 = To Double Precision Float(number=w164) -> (double precision float=w162:dbl[])
            n141 = To Double Precision Float(number=w165) -> (double precision float=w161:dbl[])
            n142 = call-poly <vilib>:"Mean.vi"("X"=w177) -> ("mean"=w182:dbl)  [unwired: 1 out]
            "LVDT 1" <- w182
            n143 = call-poly <vilib>:"Mean.vi"("X"=w176) -> ("mean"=w143:dbl)  [unwired: 1 out]
            "LVDT 2" <- w143
            n144 = call-poly <vilib>:"Mean.vi"("X"=w178) -> ("mean"=w142:dbl)  [unwired: 1 out]
            "LVDT 3" <- w142
            n145 = call-poly <vilib>:"Mean.vi"("X"=w170) -> ("mean"=w171:dbl)  [unwired: 1 out]
            "Force Sensor" <- w171
            n146 = call-poly <vilib>:"Mean.vi"("X"=w169) -> ("mean"=→"Position Piston":dbl)  [unwired: 1 out]
            n147 = call-poly <vilib>:"Mean.vi"("X"=w162) -> ("mean"=→"Pore Pressure [KPa]" →"Porendruck [Pa] 2":dbl)  [unwired: 1 out]
            n148 = call-poly <vilib>:"Mean.vi"("X"=w161) -> ("mean"=→"Side Pressure  [KPa]" →"Seitendruck [Pa] 3":dbl)  [unwired: 1 out]
            n149 = call-poly <vilib>:"Mean.vi"("X"=w163) -> ("mean"=→"Axial Pressure  [KPa]" →"Axialdruck [Pa] 4":dbl)  [unwired: 1 out]
            n150 = Bundle("mean"=w182, "mean"=w143, "mean"=w142) -> (→"LVDT Frontpannel":cluster{"mean":dbl, "mean":dbl, "mean":dbl})  [unwired: 1 in]
            n151 = Greater?(x=w171, y=-197.0) -> (0:→"Contact?":bool)
            n152 = Index Array(array=w127, index (row)=T7."Pore Volumen" ("Enum")) -> (element=w148:dbl[])  [unwired: 1 in]
            n153 = Index Array(array=w127, index (row)=T7."Side Volumen " ("Enum")) -> (element=w149:dbl[])  [unwired: 1 in]
            n154 = Index Array(array=w127, index (row)=T7."Axial Volumen " ("Enum")) -> (element=w150:dbl[])  [unwired: 1 in]
            n155 = To Double Precision Float(number=w148) -> (double precision float=w145:dbl[])
            n156 = To Double Precision Float(number=w149) -> (double precision float=w146:dbl[])
            n157 = To Double Precision Float(number=w150) -> (double precision float=w147:dbl[])
            n158 = Index Array(array=w127, index (row)=18) -> (element=w153:dbl[])  [unwired: 1 in]
            n159 = Index Array(array=w127, index (row)=T8."additional side pressure" ("Enum")) -> (element=w154:dbl[])  [unwired: 1 in]
            n160 = Index Array(array=w127, index (row)=T8."Tip resistance" ("Enum")) -> (element=w158:dbl[])  [unwired: 1 in]
            n161 = Index Array(array=w127, index (row)=T8."Pore pressure" ("Enum")) -> (element=w160:dbl[])  [unwired: 1 in]
            n162 = To Double Precision Float(number=w153) -> (double precision float=w151:dbl[])
            n163 = To Double Precision Float(number=w154) -> (double precision float=w152:dbl[])
            n164 = To Double Precision Float(number=w158) -> (double precision float=w157:dbl[])
            n165 = To Double Precision Float(number=w160) -> (double precision float=w159:dbl[])
            n166 = call-poly <vilib>:"Mean.vi"("X"=w145) -> ("mean"=w123:dbl)  [unwired: 1 out]
            "ml Pore Linear" <- w123
            "Pore" <- w123
            n167 = call-poly <vilib>:"Mean.vi"("X"=w146) -> ("mean"=w122:dbl)  [unwired: 1 out]
            "ml Side Linear" <- w122
            "Side" <- w122
            n168 = call-poly <vilib>:"Mean.vi"("X"=w147) -> ("mean"=w121:dbl)  [unwired: 1 out]
            "ml Axial Linear" <- w121
            "Axial" <- w121
            n169 = call-poly <vilib>:"Mean.vi"("X"=w151) -> ("mean"=→"Max Expansion":dbl)  [unwired: 1 out]
            n170 = call-poly <vilib>:"Mean.vi"("X"=w152) -> ("mean"=→"Addional Side Pressure":dbl)  [unwired: 1 out]
            n171 = call-poly <vilib>:"Mean.vi"("X"=w157) -> ("mean"=w141:dbl)  [unwired: 1 out]
            "Cone Tip Resistance" <- w141
            n172 = call-poly <vilib>:"Mean.vi"("X"=w159) -> ("mean"=w140:dbl)  [unwired: 1 out]
            "Cone Side Resistance" <- w140
            n173 = Bundle("mean"=w123, "mean"=w122, "mean"=w121) -> (→"ml Fontpanel":cluster{"mean":dbl, "mean":dbl, "mean":dbl})  [unwired: 1 in]
            n174 = Bundle("mean"=w141, "mean"=w140) -> (→"Cone Pressure":cluster{"mean":dbl, "mean":dbl})  [unwired: 1 in]
            n175 = call "CPT Delta_leakage_mlpm 12.1.vi"("IN Pore"=w123, "IN Side"=w122, "IN Axial"=w121, "Reset"="Reset Leackage") -> ("Time Out"=→"Timer Leackage":dbl, "OUT Pore Leakage"=→"Pore Leackage":dbl, "OUT Side Leakage"=→"Side Leackage":dbl, "OUT Axial Leakage"=→"Axial Leackage":dbl)  [unwired: 12 in]
          }
          frame #3 {
            w197 = u16 80 items=["NaN", "Kp_Position_Vibro", "Ki_Position_Vibro", "PAR_3", "Sinusfrequenz_preSh", "Zylinder_Move_Button", "PAR_6", "PAR_7", "PAR_8", "PAR_9", "PAR_10", "PAR_11", "PAR_12", "Amplitude_PreSh", "Compass_OFF", "PAR_15", "PAR_16", "SollMoog", "PAR_18", "PAR_19", "PAR_20", "Vibro_Test_Button", "PAR_22", "PAR_23", "PAR_24", "PAR_25", "PAR_26", "PAR_27", "PAR_28", "PAR_29", "PAR_30", "PAR_31", "PAR_32", "Start_Test_Button", "PAR_34", "Programm_counter", "PAR_36", "Circumference_ON_Flag", "PAR_38", "PAR_39", "Pore_Control_Button", "Side_Control_Button", "Axial_Control_Button", "PAR_43", "PAR_44", "PAR_45", "Einfahren_Piston", "PAR_47", "PAR_48", "PAR_49", "PAR_50", "PAR_51", "PAR_52", "PAR_53", "PAR_54", "PAR_55", "PAR_56", "PAR_57", "LinearUpDown_Button", "Linear_Pore_GO", "Linear_Axial_GO", "Linear_Side_GO", "PAR_62", "PAR_63", "PAR_64", "PAR_65", "PAR_66", "PAR_67", "PAR_68", "PAR_69", "Pre_Shearing_Button", "PAR_71", "PAR_72", "PAR_73", "PAR_74", "Circumf_Control_On", "PAR_76", "PAR_77", "PAR_78", "PAR_79", "Modus", "", "", "", "", "", "", "", "", "", "", "", "", "", "", "", "", "", "", "", "", "", "", "", "", "", ""] ("par_enum")
            w198 = u16 21 items=["NaN", "Kp_Position_Vibro", "Ki_Position_Vibro", "PAR_3", "Sinusfrequenz_preSh", "Zylinder_Move_Button", "PAR_6", "PAR_7", "PAR_8", "PAR_9", "PAR_10", "PAR_11", "PAR_12", "Amplitude_PreSh", "Compass_OFF", "PAR_15", "PAR_16", "SollMoog", "PAR_18", "PAR_19", "PAR_20", "Vibro_Test_Button", "PAR_22", "PAR_23", "PAR_24", "PAR_25", "PAR_26", "PAR_27", "PAR_28", "PAR_29", "PAR_30", "PAR_31", "PAR_32", "Start_Test_Button", "PAR_34", "Programm_counter", "PAR_36", "Circumference_ON_Flag", "PAR_38", "PAR_39", "Pore_Control_Button", "Side_Control_Button", "Axial_Control_Button", "PAR_43", "PAR_44", "PAR_45", "Einfahren_Piston", "PAR_47", "PAR_48", "PAR_49", "PAR_50", "PAR_51", "PAR_52", "PAR_53", "PAR_54", "PAR_55", "PAR_56", "PAR_57", "LinearUpDown_Button", "Linear_Pore_GO", "Linear_Axial_GO", "Linear_Side_GO", "PAR_62", "PAR_63", "PAR_64", "PAR_65", "PAR_66", "PAR_67", "PAR_68", "PAR_69", "Pre_Shearing_Button", "PAR_71", "PAR_72", "PAR_73", "PAR_74", "Circumf_Control_On", "PAR_76", "PAR_77", "PAR_78", "PAR_79", "Modus", "", "", "", "", "", "", "", "", "", "", "", "", "", "", "", "", "", "", "", "", "", "", "", "", "", ""] ("par_enum")
            w196 = u16 2 items=["NaN", "Kp_Position_Vibro", "Ki_Position_Vibro", "PAR_3", "Sinusfrequenz_preSh", "Zylinder_Move_Button", "PAR_6", "PAR_7", "PAR_8", "PAR_9", "PAR_10", "PAR_11", "PAR_12", "Amplitude_PreSh", "Compass_OFF", "PAR_15", "PAR_16", "SollMoog", "PAR_18", "PAR_19", "PAR_20", "Vibro_Test_Button", "PAR_22", "PAR_23", "PAR_24", "PAR_25", "PAR_26", "PAR_27", "PAR_28", "PAR_29", "PAR_30", "PAR_31", "PAR_32", "Start_Test_Button", "PAR_34", "Programm_counter", "PAR_36", "Circumference_ON_Flag", "PAR_38", "PAR_39", "Pore_Control_Button", "Side_Control_Button", "Axial_Control_Button", "PAR_43", "PAR_44", "PAR_45", "Einfahren_Piston", "PAR_47", "PAR_48", "PAR_49", "PAR_50", "PAR_51", "PAR_52", "PAR_53", "PAR_54", "PAR_55", "PAR_56", "PAR_57", "LinearUpDown_Button", "Linear_Pore_GO", "Linear_Axial_GO", "Linear_Side_GO", "PAR_62", "PAR_63", "PAR_64", "PAR_65", "PAR_66", "PAR_67", "PAR_68", "PAR_69", "Pre_Shearing_Button", "PAR_71", "PAR_72", "PAR_73", "PAR_74", "Circumf_Control_On", "PAR_76", "PAR_77", "PAR_78", "PAR_79", "Modus", "", "", "", "", "", "", "", "", "", "", "", "", "", "", "", "", "", "", "", "", "", "", "", "", "", ""] ("par_enum")
            w195 = u16 1 items=["NaN", "Kp_Position_Vibro", "Ki_Position_Vibro", "PAR_3", "Sinusfrequenz_preSh", "Zylinder_Move_Button", "PAR_6", "PAR_7", "PAR_8", "PAR_9", "PAR_10", "PAR_11", "PAR_12", "Amplitude_PreSh", "Compass_OFF", "PAR_15", "PAR_16", "SollMoog", "PAR_18", "PAR_19", "PAR_20", "Vibro_Test_Button", "PAR_22", "PAR_23", "PAR_24", "PAR_25", "PAR_26", "PAR_27", "PAR_28", "PAR_29", "PAR_30", "PAR_31", "PAR_32", "Start_Test_Button", "PAR_34", "Programm_counter", "PAR_36", "Circumference_ON_Flag", "PAR_38", "PAR_39", "Pore_Control_Button", "Side_Control_Button", "Axial_Control_Button", "PAR_43", "PAR_44", "PAR_45", "Einfahren_Piston", "PAR_47", "PAR_48", "PAR_49", "PAR_50", "PAR_51", "PAR_52", "PAR_53", "PAR_54", "PAR_55", "PAR_56", "PAR_57", "LinearUpDown_Button", "Linear_Pore_GO", "Linear_Axial_GO", "Linear_Side_GO", "PAR_62", "PAR_63", "PAR_64", "PAR_65", "PAR_66", "PAR_67", "PAR_68", "PAR_69", "Pre_Shearing_Button", "PAR_71", "PAR_72", "PAR_73", "PAR_74", "Circumf_Control_On", "PAR_76", "PAR_77", "PAR_78", "PAR_79", "Modus", "", "", "", "", "", "", "", "", "", "", "", "", "", "", "", "", "", "", "", "", "", "", "", "", "", ""] ("par_enum")
            # "Par & Fpar auslesen von ADwin. For Communicating with Adwin. Reading a Block of fpar and par and refreshing the value wit it in the GUI"
            n176 = call "ADwin Get_FPar_Block.vi"("count"=i16 80, "startindex"=i16 1, "Device No."=w273) -> ("Data"=w183:sgl[], "Device No. out"=w264:u16)  [unwired: 2 in, 2 out]
            n177 = Decrement(x=T10."PorePressOffset" ("Enum")) -> (x-1=w270:T10)
            n178 = Decrement(x=T10."AxialPressOffset" ("Enum")) -> (x-1=w269:T10)
            n179 = Decrement(x=T10."SidePressOffset" ("Enum")) -> (x-1=w268:T10)
            n180 = Decrement(x=T9."Slope_calibration" ("Enum")) -> (x-1=w188:T9)
            n181 = Decrement(x=T10."Amplitude_Vibro" ("Enum")) -> (x-1=w265:T10)
            n182 = Decrement(x=T10."PreShearingOutput" ("Enum")) -> (x-1=w226:T10)
            n183 = Decrement(x=T10."Ki_Sidepress" ("Enum")) -> (x-1=w258:T10)
            n184 = Decrement(x=T10."Kp_Axialpress" ("Enum")) -> (x-1=w257:T10)
            n185 = Decrement(x=T10."Vorschub" ("Enum")) -> (x-1=w267:T10)
            n186 = Decrement(x=T10."Kp_Porepress" ("Enum")) -> (x-1=w261:T10)
            n187 = Decrement(x=T10."Ki_Porepress" ("Enum")) -> (x-1=w260:T10)
            n188 = Decrement(x=T10."Kp_Sidepress" ("Enum")) -> (x-1=w259:T10)
            n189 = Decrement(x=T9."Intercept_calibration" ("Enum")) -> (x-1=w185:T9)
            n190 = Decrement(x=T10."Ki_Axialpress" ("Enum")) -> (x-1=w256:T10)
            n191 = Decrement(x=T10."Sinusfrequenz_Vibro" ("Enum")) -> (x-1=w266:T10)
            n192 = Index Array(array=w183, index=w270) -> ()  [unwired: 1 out]
            n193 = Index Array(array=w183, index=w269) -> ()  [unwired: 1 out]
            n194 = Index Array(array=w183, index=w268) -> ()  [unwired: 1 out]
            n195 = Index Array(array=w183, index=w266) -> (element=w263:sgl)
            n196 = Index Array(array=w183, index=w265) -> (element=w262:sgl)
            n197 = Index Array(array=w183, index=w226) -> (element=w225:sgl)
            n198 = Index Array(array=w183, index=w258) -> (element=→"Side Ki:":sgl)
            n199 = Index Array(array=w183, index=w257) -> (element=→"Axial Kp:":sgl)
            n200 = Index Array(array=w183, index=w267) -> (element=w194:sgl)
            n201 = Index Array(array=w183, index=w261) -> (element=→"Pore Kp:":sgl)
            n202 = Index Array(array=w183, index=w260) -> (element=→"Pore Ki:":sgl)
            n203 = Index Array(array=w183, index=w259) -> (element=→"Side Kp:":sgl)
            n204 = Index Array(array=w183, index=w256) -> (element=→"Axial Ki:":sgl)
            n205 = Index Array(array=w183, index=w188) -> (element=→"IS-ADWIN":sgl)
            n206 = Index Array(array=w183, index=w185) -> (element=→"IS- ADWIN":sgl)
            n207 = expression code="12000/65536*x-6000"(w225) -> (→"Pre-shearing output":sgl)
            n208 = expression code="1/x"(w263) -> (→"Frequency IS":sgl)
            n209 = expression code="x/78"(w262) -> (→"Amplitude IS":sgl)
            n210 = Multiply(x=w194, y=sgl 5000.0) -> (x*y=w191:sgl)
            n211 = Divide(x=w191, y=sgl 78.01) -> (x/y=→"Feeding IS":sgl)
            n212 = call "ADwin Get_Par_Block.vi"("count"=i16 80, "startindex"=i16 1, "Device No."=w264) -> ("Data"=w276:i32[])  [unwired: 1 in, 3 out]
            n213 = Decrement(x=w195) -> (x-1=w280:u16)
            n214 = Decrement(x=w196) -> (x-1=w279:u16)
            n215 = Decrement(x=w198) -> (x-1=w278:u16)
            n216 = Decrement(x=w197) -> (x-1=w277:u16)
            n217 = Index Array(array=w276, index=w280) -> (element=→"IS P-Value":i32)
            n218 = Index Array(array=w276, index=w279) -> (element=→"IS I-Value":i32)
            n219 = Index Array(array=w276, index=w278) -> (element=w275:i32)
            n220 = Index Array(array=w276, index=w277) -> (element=→"Modus":i32)
            n221 = Decrement(x=T10."Huang_Su_par_4" ("Enum")) -> (x-1=w246:T10)
            n222 = Decrement(x=T10."Huang_Su_par_5" ("Enum")) -> (x-1=w245:T10)
            n223 = Decrement(x=T10."Huang_Su_par_1" ("Enum")) -> (x-1=w249:T10)
            n224 = Decrement(x=T10."Huang_Su_par_2" ("Enum")) -> (x-1=w248:T10)
            n225 = Decrement(x=T10."Huang_Su_par_3" ("Enum")) -> (x-1=w247:T10)
            n226 = Decrement(x=T10."Set_Soll_AxialPressure" ("Enum")) -> (x-1=w241:T10)
            n227 = Decrement(x=T10."Huang_Su_par_6" ("Enum")) -> (x-1=w244:T10)
            n228 = Decrement(x=T10."Huang_Su_par_7" ("Enum")) -> (x-1=w243:T10)
            n229 = Decrement(x=T10."Set_Soll_PorePressure" ("Enum")) -> (x-1=w242:T10)
            n230 = Decrement(x=T10."Set_Soll_SidePressure" ("Enum")) -> (x-1=w240:T10)
            n231 = Equal?(x=w275, y=1) -> (x = y?=→"Vibro Test IS":bool)
            n232 = Index Array(array=w183, index=w241) -> (element=w235:sgl)
            n233 = Index Array(array=w183, index=w240) -> (element=w234:sgl)
            n234 = Index Array(array=w183, index=w249) -> (element=→"IS Parameter 1":sgl)
            n235 = Index Array(array=w183, index=w248) -> (element=→"IS Parameter 2":sgl)
            n236 = Index Array(array=w183, index=w247) -> (element=→"IS Parameter 3":sgl)
            n237 = Index Array(array=w183, index=w246) -> (element=→"IS Parameter 4":sgl)
            n238 = Index Array(array=w183, index=w245) -> (element=→"IS Parameter 5":sgl)
            n239 = Index Array(array=w183, index=w244) -> (element=→"IS Parameter 6":sgl)
            n240 = Index Array(array=w183, index=w243) -> (element=→"IS Parameter 7":sgl)
            n241 = Index Array(array=w183, index=w242) -> (element=w236:sgl)
            n242 = expression code="12000/65536*(x-32768)"(w236) -> (→"Porepressure":sgl)
            n243 = expression code="12000/65536*(x-32768)"(w235) -> (→"Axialpressure":sgl)
            n244 = expression code="12000/65536*(x-32768)"(w234) -> (→"Sidepressure":sgl)
          }
          frame #4 {
            (unwired) "Modification done by zhengyu chen, if measured side, pore and axial pressure is less than default\nvalues, we force them to be default values. "
            # "Set pump offset for pore, side and axial pressure sensor"
            n245 = case shown="True" "Set" {
              tunnel: w287 -> [_ w289]
              frame False {
              }
              frame True {
                n246 = call "ADwin Get_FPar_Block.vi"("count"=i16 80, "startindex"=i16 1, "Device No."=w289) -> ("Data"=w311:sgl[])  [unwired: 2 in, 3 out]
                n247 = Decrement(x=T10."SidePressOffset" ("Enum")) -> (x-1=w314:T10)
                n248 = Decrement(x=T10."AxialPressOffset" ("Enum")) -> (x-1=w313:T10)
                n249 = Decrement(x=T10."PorePressOffset" ("Enum")) -> (x-1=w312:T10)
                n250 = Index Array(array=w311, index=w314) -> (element=w307:sgl)
                n251 = Greater?(x=w307, y="Side Offset Soll 2") -> (0:w318:bool)
                n252 = Index Array(array=w311, index=w313) -> (element=w299:sgl)
                n253 = Greater?(x=w299, y="Axial Offset Soll 2") -> (0:w304:bool)
                n254 = Index Array(array=w311, index=w312) -> (element=w296:sgl)
                n255 = Greater?(x=w296, y="Pore Offset SOLL 2") -> (0:w297:bool)
                n256 = case shown="True" w304 {
                  tunnel: w289 -> [w327 w331]
                  tunnel: [w327 w331] -> w302
                  tunnel: "Axial Offset Soll 2" -> [w328 w329]
                  tunnel: [w328 w329] -> w300
                  tunnel: T10."AxialPressOffset" ("Enum") -> [w326 w330]
                  tunnel: [w326 w330] -> w301
                  tunnel: w299 -> [_ _]
                  frame False {
                  }
                  frame True {
                  }
                }
                n257 = case shown="False" w318 {
                  tunnel: w289 -> [w333 w337]
                  tunnel: [w333 w337] -> w319
                  tunnel: "Side Offset Soll 2" -> [w334 w335]
                  tunnel: [w334 w335] -> w305
                  tunnel: T10."SidePressOffset" ("Enum") -> [w332 w336]
                  tunnel: [w332 w336] -> w306
                  tunnel: w307 -> [_ _]
                  frame False {
                  }
                  frame True {
                  }
                }
                n258 = case shown="True" w297 {
                  tunnel: w289 -> [w321 w325]
                  tunnel: [w321 w325] -> w295
                  tunnel: "Pore Offset SOLL 2" -> [w322 w323]
                  tunnel: [w322 w323] -> w293
                  tunnel: T10."PorePressOffset" ("Enum") -> [w320 w324]
                  tunnel: [w320 w324] -> w294
                  tunnel: w296 -> [_ _]
                  frame False {
                  }
                  frame True {
                  }
                }
                n259 = call "ADwin Set_FPar.vi"("Value"=w305, "Index"=w306, "Device No."=w319) -> ()  [unwired: 6 in, 3 out]
                n260 = call "ADwin Set_FPar.vi"("Value"=w300, "Index"=w301, "Device No."=w302) -> ()  [unwired: 6 in, 3 out]
                n261 = call "ADwin Set_FPar.vi"("Value"=w293, "Index"=w294, "Device No."=w295) -> ()  [unwired: 6 in, 3 out]
                "Pore Offset: 2" <- "Pore Offset SOLL 2"
                "Axial Offset: 2" <- "Axial Offset Soll 2"
                "Side Offset: 2" <- "Side Offset Soll 2"
              }
            }
          }
          frame #5 {
            (unwired) "depth for 3rd vibro mode"
            (unwired) "depth for 2nd vibro mode"
            (unwired) "depth for 1st vibro mode"
            # "Visualize velocity data, filtered velocity, linear regression plots for model/based controller"
            n262 = call "ADwin Get_Par.vi"("index"=i16 76, "Device No. (1)"=w353) -> ("ParameterValue"=w371:i32)  [unwired: 7 in, 2 out]
            n263 = Subtract(x=w368, y=0) -> (x-y=w369:i32)
            n264 = Array Subset(array=w338, index (row)=0 ("index"), length (row)=w371) -> (w370:dbl[][])  [unwired: 2 in]
            n265 = call "ADwin Get_FPar.vi"("Index"=u16 23, "Device No. (1)"=w353) -> ()  [unwired: 7 in, 3 out]
            n266 = call "ADwin Get_FPar.vi"("Index"=u16 24, "Device No. (1)"=w353) -> ("ParameterValue"=w361:sgl)  [unwired: 7 in, 2 out]
            n267 = call "ADwin Get_FPar_Block.vi"("count"=i16 80, "startindex"=i16 1, "Device No."=w353) -> ("Data"=w377:sgl[])  [unwired: 2 in, 3 out]
            n268 = case shown="True" "Visualize data" {
              tunnel: w377 -> [_ w505]
              tunnel: w370 -> [_ w466]
              tunnel: w369 -> [_ w470]
              tunnel: w369 -> [_ _]
              tunnel: w366 -> [w427 w443]
              tunnel: w365 -> [w426 w442]
              tunnel: w363 -> [_ w464]
              tunnel: w361 -> [_ w449]
              tunnel: [w425 w437] -> w348
              tunnel: [w427 w443] -> w340
              tunnel: [w426 w442] -> w339
              tunnel: [w425 w437] -> w350
              tunnel: w338 -> [w425 w430]
              frame False {
                n269 = Delete From Array(array=w425, length=2, index (row)=19) -> ()  [unwired: 1 in, 2 out]
              }
              frame True {
                (unwired) "up to down:\n\n      1. desired  distance\n      2. predicted distance\n      3. measured distance\n      4. shifted predicted distance\n      5. shifted desired distance  \n"
                (unwired) " Estimated controller output"
                (unwired) " predict distance"
                (unwired) "Desired distance"
                (unwired) "fitted velocity data from linear regression"
                (unwired) "controller output"
                (unwired) "distance sensor measurement"
                (unwired) "velocity data"
                (unwired) "fitted intercept from linear regression, parameter b"
                (unwired) "fitted slope from linear regression, parameter m"
                # "Writing File"
                # "Model controller performance visualization"
                n270 = Index Array(array=w464, index (row)=2) -> (element=w445:dbl[])  [unwired: 1 in]
                n271 = Index Array(array=w466, index (row)=T8."Position Induktiv" ("Enum")) -> (element=w471:dbl[])  [unwired: 1 in]
                n272 = Index Array(array=w466, index (row)=T8."predict distance" ("Enum")) -> (element=w462:dbl[])  [unwired: 1 in]
                n273 = Index Array(array=w466, index (row)=T8."desired distance" ("Enum")) -> (element=w458:dbl[])  [unwired: 1 in]
                n274 = Index Array(array=w466, index (row)=T8."fitted velocity" ("Enum")) -> (element=w473:dbl[])  [unwired: 1 in]
                n275 = Index Array(array=w466, index (row)=T8."Distance_Regout" ("Enum")) -> (element=w461:dbl[])  [unwired: 1 in]
                n276 = Split 1D Array(array=w473, index=w470) -> ()  [unwired: 2 out]
                n277 = Index Array(array=w430, index (row)=T8."velocity data" ("Enum")) -> (element=w435:dbl[])  [unwired: 1 in]
                n278 = Index Array(array=w505, index=T10."FPAR_33" ("Enum")) -> (element=→"Slope m":sgl)
                n279 = Multiply(x=2, y=w470) -> (x*y=w475:i32)
                n280 = Split 1D Array(array=w462, index=w475) -> (second subarray=w477:dbl[])  [unwired: 1 out]
                n281 = Split 1D Array(array=w471, index=w475) -> (second subarray=w436:dbl[])  [unwired: 1 out]
                n282 = Index Array(array=w505, index=T10."FPAR_34" ("Enum")) -> (element=→"Intercept b":sgl)
                n283 = Split 1D Array(array=w461, index=0) -> (second subarray=w434:dbl[])  [unwired: 1 out]
                n284 = Less?(x=w449, y=sgl 0.0) -> (x < y?=w448:bool)
                n285 = Split 1D Array(array=w434, index=w470) -> (second subarray=w472:dbl[])  [unwired: 1 out]
                n286 = Split 1D Array(array=w477, index=w470) -> (second subarray=w451:dbl[])  [unwired: 1 out]
                n287 = Index Array(array=w430, index (row)=T8."Distance_Regout" ("Enum")) -> (element=w500:dbl[])  [unwired: 1 in]
                n288 = Index Array(array=w430, index (row)=T8."estimated_Distance_Regout" ("Enum")) -> (element=w501:dbl[])  [unwired: 1 in]
                n289 = Bundle(w434, "Output Array"=w435) -> (w432:cluster{dbl[], "Output Array":dbl[]})  [unwired: 1 in]
                n290 = Bundle(w472, "Output Array"=w435) -> (w433:cluster{dbl[], "Output Array":dbl[]})  [unwired: 1 in]
                n291 = Split 1D Array(array=w477, index=0) -> (second subarray=w469:dbl[])  [unwired: 1 out]
                n292 = Split 1D Array(array=w458, index=w470) -> (second subarray=w457:dbl[])  [unwired: 1 out]
                n293 = Build Array(w433, w432) -> (→"Linear regression":cluster{dbl[], "Output Array":dbl[]}[])
                n294 = Index Array(array=w430, index (row)=0) -> (element=w456:dbl[])  [unwired: 1 in]
                n295 = Index Array(array=w430, index (row)=T8."Distance_Regout" ("Enum")) -> (element=w479:dbl[])  [unwired: 1 in]
                n296 = Index Array(array=w430, index (row)=T8."velocity data" ("Enum")) -> (element=w439:dbl[])  [unwired: 1 in]
                n297 = Split 1D Array(array=w479, index=0) -> (second subarray=w441:dbl[])  [unwired: 1 out]
                n298 = Subtract(x=w457, y=w436) -> (x-y=w447:dbl[])
                n299 = case shown="False" w448 {
                  tunnel: w447 -> [w515 w521]
                  tunnel: [w511 w518] -> w446
                  tunnel: w445 -> [_ w519]
                  frame False {
                    n300 = Multiply(x=w515, y=1.0) -> (x*y=w513:dbl[])
                    n301 = Divide(x=w513, y=1.0) -> (x/y=w514:dbl[])
                    n302 = Sort 1D Array(array=w514) -> (sorted array=w512:dbl[])
                    n303 = Reverse 1D Array(array=w512) -> (reversed array=w511:dbl[])
                  }
                  frame True {
                    n304 = call-poly <vilib>:"Mean.vi"("X"=w521) -> ("mean"=w520:dbl)  [unwired: 1 out]
                    n305 = Multiply(x=w520, y=w519) -> (x*y=w518:dbl[])
                  }
                }
                n306 = Subtract(x=w458, y=w446) -> (x-y=w460:dbl[])
                n307 = call <vilib>:"Normalize Waveform.vi"("waveform in"=w439) -> ("normalized waveform"=w438:waveform(dbl))  [unwired: 7 in, 3 out]
                n308 = Subtract(x=w451, y=w436) -> ()  [unwired: 1 out]
                n309 = call <vilib>:"Normalize Waveform.vi"("waveform in"=w441) -> ("normalized waveform"=w440:waveform(dbl))  [unwired: 7 in, 3 out]
                n310 = Bundle("Output Array"=w456, "Output Array"=w501) -> (w499:T11)  [unwired: 1 in]
                n311 = Bundle("Output Array"=w456, "Output Array"=w500) -> (w498:T11)  [unwired: 1 in]
                n312 = Bundle("Output Array"=w456, w436) -> (w494:cluster{"Output Array":dbl[], dbl[]})  [unwired: 1 in]
                n313 = Bundle("Output Array"=w456, w469) -> (w495:cluster{"Output Array":dbl[], dbl[]})  [unwired: 1 in]
                n314 = Bundle("Output Array"=w456, "normalized waveform"=w438) -> (w503:T12)  [unwired: 1 in]
                n315 = Bundle("Output Array"=w456, w460) -> (w496:cluster{"Output Array":dbl[], dbl[]})  [unwired: 1 in]
                n316 = Bundle("Output Array"=w456, "normalized waveform"=w440) -> (w492:T12)  [unwired: 1 in]
                n317 = Bundle("Output Array"=w456, w451) -> (w491:cluster{"Output Array":dbl[], dbl[]})  [unwired: 1 in]
                n318 = Subtract(x=w457, y=w446) -> (x-y=w459:dbl[])
                n319 = Build Array(w499, w498) -> (→"Controller Output":T2)
                n320 = Build Array(w492, w503) -> (→"Velocity vs Controller output":T13)
                n321 = Subtract(x=w447, y=w446) -> (x-y=→"Distance Difference Graph 2":dbl[])
                n322 = Bundle("Output Array"=w456, w459) -> (w474:cluster{"Output Array":dbl[], dbl[]})  [unwired: 1 in]
                n323 = Build Array(w496, w495, w494, w491, w474) -> (→"Distance Graph":cluster{"Output Array":dbl[], dbl[]}[])
                n324 = Array Max & Min(array=w447) -> (max value=w455:dbl, min value=w454:dbl)  [unwired: 2 out]
                n325 = Subtract(x=w455, y=w454) -> (x-y=w453:dbl)
                n326 = Delete From Array(array=w430, length=2, index (row)=19) -> (array with subset deleted=w465:dbl[][])  [unwired: 1 in, 1 out]
                n327 = Array Size(array=w447) -> (size(s)=w452:i32)
                n328 = Divide(x=w453, y=w452) -> ()  [unwired: 1 out]
                n329 = Insert Into Array(array=w465, new element #1=w460, new element #2=w469, new element #3=w436, new element #4=w451, new element #5=w459) -> (w437:dbl[][])  [unwired: 2 in]
              }
            }
            n330 = Index Array(array=w348, index (row)=T8."Position Induktiv" ("Enum")) -> (element=w359:dbl[])  [unwired: 1 in]
            n331 = call "ADwin Get_FPar.vi"("Index"=u16 70, "Device No. (1)"=w353) -> ("ParameterValue"=w347:sgl)  [unwired: 7 in, 2 out]
            n332 = call "ADwin Get_FPar.vi"("Index"=u16 69, "Device No. (1)"=w353) -> ("ParameterValue"=w351:sgl)  [unwired: 7 in, 2 out]
            n333 = Index Array(array=w359, index=1) -> (element=w344:dbl)
            n334 = call "ADwin Get_FPar.vi"("Index"=u16 46, "Device No. (1)"=w353) -> ("ParameterValue"=w343:sgl)  [unwired: 7 in, 2 out]
            n335 = In Range and Coerce(upper limit=w351, x=w344, lower limit=0.0) -> (In Range?=w355:bool)  [unwired: 1 out]
            n336 = In Range and Coerce(upper limit=w347, x=w344, lower limit=w351) -> (In Range?=w349:bool)  [unwired: 1 out]
            n337 = In Range and Coerce(upper limit=w343, x=w344, lower limit=w347) -> (In Range?=w346:bool)  [unwired: 1 out]
            n338 = In Range and Coerce(upper limit=421.0, x=w344, lower limit=w343) -> (In Range?=w342:bool)  [unwired: 1 out]
            n339 = case shown="True" "Set file" {
              tunnel: w355 -> [_ w394]
              tunnel: w350 -> [w380 w393]
              tunnel: w349 -> [_ w392]
              tunnel: w348 -> [_ w391]
              tunnel: w346 -> [_ w390]
              tunnel: w339 -> [_ w389]
              tunnel: w342 -> [_ w388]
              tunnel: w340 -> [w379 _]
              tunnel: w339 -> [w378 _]
              frame False {
                (unwired) "save CPT data in one whole file"
                n340 = case shown="True" w378 {
                  tunnel: w380 -> [_ w383]
                  tunnel: w379 -> [_ w385]
                  frame False {
                  }
                  frame True {
                    w387 = TRUE ("append to file? (new file:F)")
                    n341 = Index Array(array=w383, index (row)=12) -> (element=→"Waveform Chart":dbl[])  [unwired: 1 in]
                    n342 = call-poly <vilib>:"Write To Spreadsheet File.vi"("delimiter (\\t)"=";" ("delimiter (\\t)"), "transpose? (no:F)"=w387, "format (%.3f)"="%.;%.4f", "append to file? (new file:F)"=w387, "2D data"=w383, "file path (dialog if empty)"=w385) -> ()  [unwired: 2 in, 1 out]
                  }
                }
              }
              frame True {
                n343 = case shown="True" w389 {
                  tunnel: w394 -> [_ w404]
                  tunnel: w393 -> [_ w403]
                  tunnel: w392 -> [_ w402]
                  tunnel: w391 -> [_ w401]
                  tunnel: w390 -> [_ w400]
                  tunnel: w388 -> [_ w399]
                  frame False {
                  }
                  frame True {
                    (unwired) "Store test data in different files"
                    n344 = case shown="True" w404 {
                      tunnel: w403 -> [_ w417]
                      tunnel: "Vibro test 1" -> [_ w416]
                      frame False {
                      }
                      frame True {
                        w419 = TRUE ("append to file? (new file:F)")
                        n345 = call-poly <vilib>:"Write To Spreadsheet File.vi"("delimiter (\\t)"=";" ("delimiter (\\t)"), "transpose? (no:F)"=w419, "format (%.3f)"="%.;%.4f", "append to file? (new file:F)"=w419, "2D data"=w417, "file path (dialog if empty)"=w416) -> ()  [unwired: 2 in, 1 out]
                      }
                    }
                    n346 = case shown="True" w402 {
                      tunnel: w403 -> [_ w412]
                      tunnel: "Vibro test 2" -> [_ w411]
                      frame False {
                      }
                      frame True {
                        w414 = TRUE ("append to file? (new file:F)")
                        n347 = call-poly <vilib>:"Write To Spreadsheet File.vi"("delimiter (\\t)"=";" ("delimiter (\\t)"), "transpose? (no:F)"=w414, "format (%.3f)"="%.;%.4f", "append to file? (new file:F)"=w414, "2D data"=w412, "file path (dialog if empty)"=w411) -> ()  [unwired: 2 in, 1 out]
                      }
                    }
                    n348 = case shown="True" w400 {
                      tunnel: w401 -> [_ w407]
                      tunnel: "Vibro test 3" -> [_ w406]
                      frame False {
                      }
                      frame True {
                        w409 = TRUE ("append to file? (new file:F)")
                        n349 = call-poly <vilib>:"Write To Spreadsheet File.vi"("delimiter (\\t)"=";" ("delimiter (\\t)"), "transpose? (no:F)"=w409, "format (%.3f)"="%.;%.4f", "append to file? (new file:F)"=w409, "2D data"=w407, "file path (dialog if empty)"=w406) -> ()  [unwired: 2 in, 1 out]
                      }
                    }
                    n350 = case shown="True" w399 {
                      tunnel: w401 -> [_ w422]
                      tunnel: "Static peneration test" -> [_ w421]
                      frame False {
                      }
                      frame True {
                        w424 = TRUE ("append to file? (new file:F)")
                        n351 = call-poly <vilib>:"Write To Spreadsheet File.vi"("delimiter (\\t)"=";" ("delimiter (\\t)"), "transpose? (no:F)"=w424, "format (%.3f)"="%.;%.4f", "append to file? (new file:F)"=w424, "2D data"=w422, "file path (dialog if empty)"=w421) -> ()  [unwired: 2 in, 1 out]
                      }
                    }
                  }
                }
              }
            }
          }
          frame #6 {
            (unwired) "Only use one period of data"
            (unwired) "Velocity deviation"
            (unwired) "acceleration"
            # "Perform correlation to get time delay"
            n352 = call "ADwin Get_Par.vi"("index"=i16 76, "Device No. (1)"=w522) -> ("ParameterValue"=w525:i32)  [unwired: 7 in, 2 out]
            n353 = Array Subset(array=w524, index (row)=0 ("index"), length (row)=w525) -> (w523:dbl[][])  [unwired: 2 in]
            n354 = Index Array(array=w528, index (row)=0) -> (element=w534:dbl[])  [unwired: 1 in]
            n355 = Index Array(array=w528, index (row)=1) -> (element=w531:dbl[])  [unwired: 1 in]
            n356 = Index Array(array=w523, index (row)=0) -> (element=w529:dbl[])  [unwired: 1 in]
            n357 = Bundle(w529, "Output Array 2"=w534) -> (→"Acceleration":cluster{dbl[], "Output Array 2":dbl[]})  [unwired: 1 in]
            n358 = Bundle(w529, "Output Array 2"=w531) -> (→"Velocity deviation":cluster{dbl[], "Output Array 2":dbl[]})  [unwired: 1 in]
            n359 = case shown="True" "Start Correlation" {
              tunnel: w523 -> [w538 w564]
              tunnel: w522 -> [_ w541]
              frame False {
                (unwired) "normalized velocity"
                n360 = Index Array(array=w538, index (row)=25) -> ()  [unwired: 1 in, 1 out]
                n361 = Index Array(array=w538, index (row)=26) -> ()  [unwired: 1 in, 1 out]
              }
              frame True {
                (unwired) "correlation between distance measurement and controller output"
                (unwired) 1 ("index (row)")
                (unwired) "normalized controller output"
                (unwired) "normalized velocity"
                n362 = call "ADwin Set_Par.vi"("Value"=0, "Index"=i16 9, "Device No."=w541) -> ()  [unwired: 6 in, 3 out]
                n363 = Index Array(array=w564, index (row)=T8."velocity data" ("Enum")) -> (element=w547:dbl[])  [unwired: 1 in]
                n364 = Index Array(array=w564, index (row)=T8."Distance_Regout" ("Enum")) -> (element=w546:dbl[])  [unwired: 1 in]
                n365 = Index Array(array=w564, index (row)=T8."Position Induktiv" ("Enum")) -> (element=w559:dbl[])  [unwired: 1 in]
                n366 = call-poly <vilib>:"Normalize.vi"("Vector"=w546) -> ("Normalized Vector"=w545:dbl[])  [unwired: 1 in, 3 out]
                n367 = Index Array(array=w564, index (row)=T8."Distance_Regout" ("Enum")) -> (element=w561:dbl[])  [unwired: 1 in]
                n368 = call-poly <vilib>:"Normalize.vi"("Vector"=w547) -> ("Normalized Vector"=w544:dbl[])  [unwired: 1 in, 3 out]
                n369 = Array Size(array=w544) -> (size(s)=w565:i32)
                n370 = call <vilib>:"Normalize Waveform.vi"("waveform in"=w559) -> ("normalized waveform"=w562:waveform(dbl))  [unwired: 7 in, 3 out]
                n371 = call <vilib>:"Normalize Waveform.vi"("waveform in"=w561) -> ("normalized waveform"=w560:waveform(dbl))  [unwired: 7 in, 3 out]
                n372 = Split 1D Array(array=w545, index=0) -> (second subarray=w543:dbl[])  [unwired: 1 out]
                n373 = Array Size(array=w559) -> (size(s)=w558:i32)
                n374 = call-poly <vilib>:"CrossCorrelation.vi"("Y"=w560, "X"=w562) -> ("Rxy"=w563:dbl[])  [unwired: 8 in, 1 out]
                n375 = Array Max & Min(array=w563) -> (max index (indices)=w566:i32)  [unwired: 3 out]
                n376 = call-poly <vilib>:"CrossCorrelation.vi"("normalization"=enum32{"none", "unbiased", "biased"}."none", "algorithm"=enum32{"direct", "frequency domain"}."direct", "Y"=w544, "X"=w543) -> ("Rxy"=w542:dbl[])  [unwired: 6 in, 1 out]
                "Correlation curve" <- w542
                n377 = Array Max & Min(array=w542) -> (max index (indices)=w574:i32)  [unwired: 3 out]
                n378 = Subtract(x=w574, y=w565) -> (x-y=w573:i32)
                n379 = Absolute Value(x=w573) -> (abs(x)=w550:i32)
                n380 = Subtract(x=w566, y=w558) -> (x-y=w567:i32)
                n381 = Absolute Value(x=w567) -> (abs(x)=w570:i32)
                n382 = Round To Nearest(number=w550) -> (nearest integer value=w552:i32)
                n383 = Divide(x=w570, y=1) -> (x/y=w568:dbl)
                n384 = Round To Nearest(number=w568) -> ()  [unwired: 1 out]
                n385 = Subtract(x=w552, y=0 ("index")) -> (x-y=w548:i32)
                n386 = Divide(x=w548, y=1) -> ()  [unwired: 1 out]
              }
            }
          }
          frame #7 {
            # "Visualize pressure control data"
            n387 = case shown="False" "Visualize data" {
              tunnel: w577 -> [_ w581]
              frame False {
              }
              frame True {
                n388 = Index Array(array=w581, index (row)=T8."Soll_Porepress" ("Enum")) -> (element=w605:dbl[])  [unwired: 1 in]
                n389 = expression code="12000/65536*x-6000"(w605) -> (w603:dbl[])
                n390 = Index Array(array=w581, index (row)=T8."Soll_Sidepress" ("Enum")) -> (element=w595:dbl[])  [unwired: 1 in]
                n391 = Index Array(array=w581, index (row)=T8."Program Counter" ("Enum")) -> (element=w604:dbl[])  [unwired: 1 in]
                n392 = Index Array(array=w581, index (row)=T8."Pore Pressure" ("Enum")) -> (element=w607:dbl[])  [unwired: 1 in]
                n393 = Index Array(array=w581, index (row)=T8."Soll_axialpress" ("Enum")) -> (element=w586:dbl[])  [unwired: 1 in]
                n394 = expression code="12000/65536*x-6000"(w595) -> (w593:dbl[])
                n395 = expression code="12000/65536*x -6000"(w586) -> (w584:dbl[])
                n396 = Index Array(array=w581, index (row)=T8."Program Counter" ("Enum")) -> (element=w594:dbl[])  [unwired: 1 in]
                n397 = Index Array(array=w581, index (row)=T8."Side Pressure " ("Enum")) -> (element=w597:dbl[])  [unwired: 1 in]
                n398 = Index Array(array=w581, index (row)=T8."Program Counter" ("Enum")) -> (element=w585:dbl[])  [unwired: 1 in]
                n399 = Index Array(array=w581, index (row)=T8."Axial Pressure" ("Enum")) -> (element=w588:dbl[])  [unwired: 1 in]
                n400 = Bundle("Output Array"=w604, "Output Array"=w607) -> (w602:T11)  [unwired: 1 in]
                n401 = Bundle("Output Array"=w604, "Output Array"=w603) -> (w601:T11)  [unwired: 1 in]
                n402 = Bundle("Output Array"=w594, "Output Array"=w597) -> (w592:T11)  [unwired: 1 in]
                n403 = Bundle("Output Array"=w585, "Output Array"=w588) -> (w583:T11)  [unwired: 1 in]
                n404 = Bundle("Output Array"=w594, "Output Array"=w593) -> (w591:T11)  [unwired: 1 in]
                n405 = Build Array(w602, w601) -> (→"Pore Pressure":T2)
                n406 = Bundle("Output Array"=w585, "Output Array"=w584) -> (w582:T11)  [unwired: 1 in]
                n407 = Build Array(w592, w591) -> (→"Side Pressure":T2)
                n408 = Build Array(w583, w582) -> (→"Axial Pressure":T2)
              }
            }
          }
          frame #8 {
            # "Control parameters setup and activation, Switch frequency mode Setup"
            n409 = case shown="True" "Control start" {
              tunnel: w610 -> [_ w627]
              frame False {
              }
              frame True {
                n410 = call "ADwin Set_Par.vi"("Value"=sgl 1.0, "Index"=i16 39, "Device No."=w627) -> ()  [unwired: 6 in, 3 out]
              }
            }
            n411 = case shown="True" TRUE {
              tunnel: w617 -> [_ _]
              tunnel: w610 -> [_ _]
              tunnel: w610 -> [_ w660]
              tunnel: w616 -> [_ _]
              tunnel: w610 -> [_ w668]
              tunnel: [w657 w666] -> w615
              tunnel: "Switch Vibro Mode" -> [w657 w666]
              frame False {
              }
              frame True {
                n412 = case shown="True" w666 {
                  tunnel: w668 -> [_ w721]
                  frame False {
                  }
                  frame True {
                    n413 = call "ADwin Set_FPar.vi"("Value"="Time delay-3", "Index"=i16 66, "Device No."=w721) -> ()  [unwired: 6 in, 3 out]
                  }
                }
                n414 = case shown="True" w666 {
                  tunnel: w668 -> [_ w718]
                  frame False {
                  }
                  frame True {
                    n415 = call "ADwin Set_FPar.vi"("Value"="Depth(mm)3", "Index"=i16 70, "Device No."=w718) -> ()  [unwired: 6 in, 3 out]
                  }
                }
                n416 = case shown="True" w666 {
                  tunnel: w660 -> [_ w723]
                  frame False {
                  }
                  frame True {
                    n417 = call "ADwin Set_Par.vi"("Value"=sgl 1.0, "Index"=i16 6, "Device No."=w723) -> ()  [unwired: 6 in, 3 out]
                  }
                }
                n418 = call "ADwin Get_Par.vi"("index"=i16 10, "Device No. (1)"=w660) -> ("ParameterValue"=w663:i32)  [unwired: 7 in, 2 out]
                n419 = call "ADwin Get_Par.vi"("index"=i16 11, "Device No. (1)"=w660) -> ("ParameterValue"=w667:i32)  [unwired: 7 in, 2 out]
                n420 = case shown="True" "Enable Vibro Mode 3" {
                  tunnel: w668 -> [_ w698]
                  tunnel: w667 -> [_ w697]
                  tunnel: w666 -> [_ w696]
                  tunnel: w660 -> [_ w695]
                  frame False {
                  }
                  frame True {
                    n421 = call "ADwin Set_Par.vi"("Value"=1, "Index"=i16 35, "Device No."=w695) -> ()  [unwired: 6 in, 3 out]
                    n422 = case shown="1" w697 {
                      tunnel: w698 -> [_ w699]
                      tunnel: w696 -> [_ w705]
                      tunnel: w698 -> [_ w704]
                      tunnel: w698 -> [_ w703]
                      frame 0, Default {
                      }
                      frame 1 {
                        n423 = case shown="True" w705 {
                          tunnel: w699 -> [_ w715]
                          tunnel: "freq-3 ( Hz) 2" -> [_ w714]
                          frame False {
                          }
                          frame True {
                            n424 = call "ADwin Set_FPar.vi"("Value"=w714, "Index"=i16 26, "Device No."=w715) -> ()  [unwired: 6 in, 3 out]
                          }
                        }
                        n425 = case shown="True" w705 {
                          tunnel: w704 -> [_ w706]
                          tunnel: "Background velocity-3" -> [_ w707]
                          frame False {
                          }
                          frame True {
                            n426 = call "ADwin Set_FPar.vi"("Value"=w707, "Index"=i16 24, "Device No."=w706) -> ()  [unwired: 6 in, 3 out]
                          }
                        }
                        n427 = case shown="True" w705 {
                          tunnel: w703 -> [_ w712]
                          tunnel: "Amplitdue-3" -> [_ w711]
                          frame False {
                          }
                          frame True {
                            n428 = Multiply(x=w711, y=2.0) -> (x*y=w709:dbl)
                            n429 = call "ADwin Set_FPar.vi"("Value"=w709, "Index"=i16 23, "Device No."=w712) -> ()  [unwired: 6 in, 3 out]
                          }
                        }
                      }
                    }
                  }
                }
                n430 = case shown="True" w666 {
                  tunnel: w668 -> [_ w729]
                  frame False {
                  }
                  frame True {
                    n431 = call "ADwin Set_FPar.vi"("Value"="Time delay-2", "Index"=i16 65, "Device No."=w729) -> ()  [unwired: 6 in, 3 out]
                  }
                }
                n432 = case shown="True" w666 {
                  tunnel: w668 -> [_ w727]
                  frame False {
                  }
                  frame True {
                    n433 = call "ADwin Set_FPar.vi"("Value"="Depth(mm)2", "Index"=i16 69, "Device No."=w727) -> ()  [unwired: 6 in, 3 out]
                  }
                }
                n434 = call "ADwin Set_FPar.vi"("Value"="Time delay - 4", "Index"=i16 47, "Device No."=w660) -> ()  [unwired: 6 in, 3 out]
                n435 = call "ADwin Set_FPar.vi"("Value"="Static penetration Depth(mm) - 4", "Index"=i16 46, "Device No."=w660) -> ()  [unwired: 6 in, 3 out]
                n436 = case shown="True" "Enable Vibro Mode 2" {
                  tunnel: w663 -> [_ w676]
                  tunnel: w668 -> [_ w675]
                  tunnel: w666 -> [_ w674]
                  tunnel: w660 -> [_ w671]
                  frame False {
                  }
                  frame True {
                    n437 = call "ADwin Set_Par.vi"("Value"=1, "Index"=i16 34, "Device No."=w671) -> ()  [unwired: 6 in, 3 out]
                    n438 = case shown="1" w676 {
                      tunnel: w675 -> [_ w678]
                      tunnel: w674 -> [_ w677]
                      frame 0, Default {
                      }
                      frame 1 {
                        n439 = case shown="True" w677 {
                          tunnel: w678 -> [_ w691]
                          tunnel: "freq-2 ( Hz)" -> [_ w690]
                          frame False {
                          }
                          frame True {
                            n440 = call "ADwin Set_FPar.vi"("Value"=w690, "Index"=i16 26, "Device No."=w691) -> ()  [unwired: 6 in, 3 out]
                          }
                        }
                        n441 = case shown="True" w677 {
                          tunnel: w678 -> [_ w688]
                          tunnel: "Amplitdue-2" -> [_ w687]
                          frame False {
                          }
                          frame True {
                            n442 = Multiply(x=w687, y=2.0) -> (x*y=w685:dbl)
                            n443 = call "ADwin Set_FPar.vi"("Value"=w685, "Index"=i16 23, "Device No."=w688) -> ()  [unwired: 6 in, 3 out]
                          }
                        }
                        n444 = case shown="True" w677 {
                          tunnel: w678 -> [_ w683]
                          tunnel: "Background velocity-2" -> [_ w682]
                          frame False {
                          }
                          frame True {
                            n445 = call "ADwin Set_FPar.vi"("Value"=w682, "Index"=i16 24, "Device No."=w683) -> ()  [unwired: 6 in, 3 out]
                          }
                        }
                      }
                    }
                  }
                }
              }
            }
            n446 = case shown="True" "Control Stop" {
              tunnel: w610 -> [w651 w654]
              frame False {
                n447 = call "ADwin Set_FPar.vi"("Value"=sgl 0.0, "Index"=i16 71, "Device No."=w651) -> ()  [unwired: 6 in, 3 out]
              }
              frame True {
                n448 = call "ADwin Set_FPar.vi"("Value"=sgl 1.0, "Index"=i16 71, "Device No."=w654) -> ()  [unwired: 6 in, 3 out]
              }
            }
            n449 = case shown="False" "Finish test" {
              tunnel: w610 -> [_ w624]
              tunnel: w610 -> [w619 _]
              frame False {
                n450 = case shown="True" "Activate" {
                  tunnel: w619 -> [_ w621]
                  frame False {
                  }
                  frame True {
                    n451 = call "ADwin Set_Par.vi"("Value"=sgl 12.0, "Index"=i16 80, "Device No."=w621) -> ()  [unwired: 6 in, 3 out]
                  }
                }
              }
              frame True {
                n452 = call "ADwin Set_Par.vi"("Value"=sgl 1.0, "Index"=i16 15, "Device No."=w624) -> ()  [unwired: 6 in, 3 out]
              }
            }
            n453 = case shown="False" w615 {
              tunnel: w610 -> [w630 _]
              frame False {
                n454 = case shown="True" "Enable Vibro Mode 1" {
                  tunnel: w630 -> [_ w638]
                  frame False {
                  }
                  frame True {
                    w632 = 0.5 ("y")
                    n455 = Multiply(x="Amplitude - 1 (mm)", y=2.0) -> (x*y=w635:dbl)
                    n456 = case shown="True" TRUE {
                      tunnel: w638 -> [_ _]
                      tunnel: "Vibration frequency - 1  (Hz)" -> [_ w649]
                      tunnel: w638 -> [_ w648]
                      frame False {
                      }
                      frame True {
                        n457 = call "ADwin Set_FPar.vi"("Value"=w649, "Index"=i16 26, "Device No."=w648) -> ()  [unwired: 6 in, 3 out]
                      }
                    }
                    n458 = Less?(x="background velocity -1 (mm/s)", y=w632) -> (x < y?=w634:bool)
                    n459 = call "ADwin Set_FPar.vi"("Value"=w635, "Index"=i16 23, "Device No."=w638) -> ()  [unwired: 6 in, 3 out]
                    n460 = case shown="True" w634 {
                      tunnel: w638 -> [w643 w646]
                      tunnel: "background velocity -1 (mm/s)" -> [w642 w645]
                      tunnel: w632 -> [_ _]
                      frame False {
                        n461 = call "ADwin Set_FPar.vi"("Value"=w642, "Index"=i16 24, "Device No."=w643) -> ()  [unwired: 6 in, 3 out]
                      }
                      frame True {
                        n462 = call "ADwin Set_FPar.vi"("Value"=w645, "Index"=i16 24, "Device No."=w646) -> ()  [unwired: 6 in, 3 out]
                      }
                    }
                  }
                }
              }
              frame True {
              }
            }
          }
          frame #9 {
            n463 = case shown="True" "Set" {
              tunnel: w734 -> [_ w738]
              frame False {
              }
              frame True {
                n464 = call "ADwin Set_FPar.vi"("Value"="maximum acceptable \nSide volume change (ml)", "Index"=i16 32, "Device No."=w738) -> ()  [unwired: 6 in, 3 out]
              }
            }
            n465 = call "ADwin Get_FPar.vi"("Index"=u16 33, "Device No. (1)"=w734) -> ("ParameterValue"=→"Actual side volume change (ml)":sgl)  [unwired: 7 in, 2 out]
          }
          frame #10 {
            # "Linear calibration with BC5"
            n466 = call "ADwin Get_FPar_Block.vi"("count"=i16 80, "startindex"=i16 1, "Device No."=w742) -> ("Data"=w741:sgl[], "Device No. out"=w740:u16)  [unwired: 2 in, 2 out]
            n467 = case shown="True" "Calibration start" {
              tunnel: w741 -> [_ _]
              tunnel: w740 -> [w746 w754]
              tunnel: w739 -> [_ w751]
              frame False {
                n468 = call "ADwin Set_Par.vi"("Value"=sgl 0.0, "Index"=i16 72, "Device No."=w746) -> ()  [unwired: 6 in, 3 out]
              }
              frame True {
                (unwired) " Position of Piston"
                (unwired) "Strain"
                (unwired) "Additional Side Pressure"
                n469 = call "ADwin Set_Par.vi"("Value"=sgl 1.0, "Index"=i16 72, "Device No."=w754) -> ()  [unwired: 6 in, 3 out]
                n470 = Index Array(array=w751, index (row)=2) -> (element=→"Piston Position (mm)":dbl[])  [unwired: 1 in]
                n471 = Index Array(array=w751, index (row)=30) -> (element=w765:dbl[])  [unwired: 1 in]
                n472 = Index Array(array=w751, index (row)=31) -> (element=w764:dbl[])  [unwired: 1 in]
                n473 = Bundle("Output Array"=w765, "Output Array"=w764) -> (→"Linear calibration":T11)  [unwired: 1 in]
                n474 = call "ADwin Set_FPar.vi"("Value"="Starting penetration depth (mm)  2", "Index"=i16 29, "Device No."=w754) -> ()  [unwired: 6 in, 3 out]
                n475 = call "ADwin Set_FPar.vi"("Value"="initial strain r0", "Index"=i16 30) -> ()  [unwired: 7 in, 3 out]
                n476 = call "ADwin Set_FPar.vi"("Value"="Initial cone position (mm)", "Index"=i16 31, "Device No."=w754) -> ()  [unwired: 6 in, 3 out]
              }
            }
          }
          frame #11 {
            # "Linear Pressure Control"
            n477 = local read "Delta Seiten"() -> (w773:dbl)
            n478 = local read "Delta Axial"() -> (w768:dbl)
            n479 = local read "Go - Porendruck"() -> (w780:bool)
            n480 = local read "Go - Seitendruck"() -> (w775:bool)
            n481 = local read "Go - Axialdruck"() -> (w770:bool)
            n482 = local read "Delta Pore"() -> (w778:dbl)
            n483 = Greater?(x=w768, y=0.0) -> (0:w771:bool)
            n484 = Greater?(x=w773, y=0.0) -> (0:w776:bool)
            n485 = Greater?(x=w778, y=0.0) -> (0:w781:bool)
            n486 = And(x=w770, y=w771) -> (x .and. y?=w769:bool)
            n487 = And(x=w775, y=w776) -> (x .and. y?=w774:bool)
            n488 = And(x=w780, y=w781) -> (x .and. y?=w779:bool)
            n489 = local read "Up_Lower"() -> (w784:bool)
            n490 = case shown="True" w779 {
              tunnel: w784 -> [w832 w840]
              tunnel: [w832 w840] -> w783
              tunnel: w766 -> [_ w835]
              frame False {
                n491 = local read "Pore Pressure [KPa]"() -> (→"Porendruck save":dbl)
              }
              frame True {
                n492 = local read "Porendruck save"() -> (w838:dbl)
                n493 = local read "Porepressure"() -> (w834:dbl)
                n494 = case shown="True" w840 {
                  tunnel: "Delta Pore" -> [w850 w854]
                  tunnel: w838 -> [w849 w855]
                  tunnel: [w848 w853] -> w837
                  tunnel: w834 -> [w847 w852]
                  tunnel: [w846 w851] -> w836
                  frame False {
                    n495 = Subtract(x=w849, y=w850) -> (x-y=w848:dbl)
                    n496 = Greater?(x=w848, y=w847) -> (0:w846:bool)
                  }
                  frame True {
                    n497 = Add(x=w855, y=w854) -> (x+y=w853:dbl)
                    n498 = Greater?(x=w852, y=w853) -> (0:w851:bool)
                  }
                }
                n499 = case shown="True" w836 {
                  tunnel: w835 -> [_ w842]
                  frame False {
                  }
                  frame True {
                    w843 = u16 59 items=["NaN", "Kp_Position_Vibro", "Ki_Position_Vibro", "PAR_3", "Sinusfrequenz_preSh", "Zylinder_Move_Button", "PAR_6", "PAR_7", "PAR_8", "PAR_9", "PAR_10", "PAR_11", "PAR_12", "Amplitude_PreSh", "Compass_OFF", "PAR_15", "PAR_16", "SollMoog", "PAR_18", "PAR_19", "PAR_20", "Vibro_Test_Button", "PAR_22", "PAR_23", "PAR_24", "PAR_25", "PAR_26", "PAR_27", "PAR_28", "PAR_29", "PAR_30", "PAR_31", "PAR_32", "Start_Test_Button", "PAR_34", "Programm_counter", "PAR_36", "Circumference_ON_Flag", "PAR_38", "PAR_39", "Pore_Control_Button", "Side_Control_Button", "Axial_Control_Button", "PAR_43", "PAR_44", "PAR_45", "Einfahren_Piston", "PAR_47", "PAR_48", "PAR_49", "PAR_50", "PAR_51", "PAR_52", "PAR_53", "PAR_54", "PAR_55", "PAR_56", "PAR_57", "LinearUpDown_Button", "Linear_Pore_GO", "Linear_Axial_GO", "Linear_Side_GO", "PAR_62", "PAR_63", "PAR_64", "PAR_65", "PAR_66", "PAR_67", "PAR_68", "PAR_69", "Pre_Shearing_Button", "PAR_71", "PAR_72", "PAR_73", "PAR_74", "Circumf_Control_On", "PAR_76", "PAR_77", "PAR_78", "PAR_79", "Modus", "", "", "", "", "", "", "", "", "", "", "", "", "", "", "", "", "", "", "", "", "", "", "", "", "", ""] ("par_enum")
                    n500 = local write "Go - Porendruck"(FALSE ("Go - Porendruck")) -> ()
                    n501 = local write "Delta Pore"(0.0 ("Delta Pore")) -> ()
                    n502 = call "ADwin Set_Par.vi"("Value"=0, "Index"=w843, "Device No."=w842) -> ()  [unwired: 6 in, 3 out]
                  }
                }
                n503 = local write "Soll Pore Pressure"(w837) -> ()
              }
            }
            n504 = case shown="True" w774 {
              tunnel: w783 -> [w809 w816]
              tunnel: [w809 w816] -> w782
              tunnel: w766 -> [_ w811]
              frame False {
                n505 = local read "Side Pressure  [KPa]"() -> (→"Seitendruck save":dbl)
              }
              frame True {
                n506 = local read "Seitendruck save"() -> (w814:dbl)
                n507 = local read "Sidepressure"() -> (w810:dbl)
                n508 = case shown="True" w816 {
                  tunnel: "Delta Seiten" -> [w826 w830]
                  tunnel: w814 -> [w825 w831]
                  tunnel: [w824 w829] -> w812
                  tunnel: w810 -> [w823 w828]
                  tunnel: [w822 w827] -> w813
                  frame False {
                    n509 = Subtract(x=w825, y=w826) -> (x-y=w824:dbl)
                    n510 = Greater?(x=w824, y=w823) -> (0:w822:bool)
                  }
                  frame True {
                    n511 = Add(x=w831, y=w830) -> (x+y=w829:dbl)
                    n512 = Greater?(x=w828, y=w829) -> (0:w827:bool)
                  }
                }
                n513 = local write "Soll Side Pressure"(w812) -> ()
                n514 = case shown="True" w813 {
                  tunnel: w811 -> [_ w818]
                  frame False {
                  }
                  frame True {
                    w819 = u16 61 items=["NaN", "Kp_Position_Vibro", "Ki_Position_Vibro", "PAR_3", "Sinusfrequenz_preSh", "Zylinder_Move_Button", "PAR_6", "PAR_7", "PAR_8", "PAR_9", "PAR_10", "PAR_11", "PAR_12", "Amplitude_PreSh", "Compass_OFF", "PAR_15", "PAR_16", "SollMoog", "PAR_18", "PAR_19", "PAR_20", "Vibro_Test_Button", "PAR_22", "PAR_23", "PAR_24", "PAR_25", "PAR_26", "PAR_27", "PAR_28", "PAR_29", "PAR_30", "PAR_31", "PAR_32", "Start_Test_Button", "PAR_34", "Programm_counter", "PAR_36", "Circumference_ON_Flag", "PAR_38", "PAR_39", "Pore_Control_Button", "Side_Control_Button", "Axial_Control_Button", "PAR_43", "PAR_44", "PAR_45", "Einfahren_Piston", "PAR_47", "PAR_48", "PAR_49", "PAR_50", "PAR_51", "PAR_52", "PAR_53", "PAR_54", "PAR_55", "PAR_56", "PAR_57", "LinearUpDown_Button", "Linear_Pore_GO", "Linear_Axial_GO", "Linear_Side_GO", "PAR_62", "PAR_63", "PAR_64", "PAR_65", "PAR_66", "PAR_67", "PAR_68", "PAR_69", "Pre_Shearing_Button", "PAR_71", "PAR_72", "PAR_73", "PAR_74", "Circumf_Control_On", "PAR_76", "PAR_77", "PAR_78", "PAR_79", "Modus", "", "", "", "", "", "", "", "", "", "", "", "", "", "", "", "", "", "", "", "", "", "", "", "", "", ""] ("par_enum")
                    n515 = local write "Go - Seitendruck"(FALSE ("Go - Seitendruck")) -> ()
                    n516 = local write "Delta Seiten"(0.0 ("Delta Seiten")) -> ()
                    n517 = call "ADwin Set_Par.vi"("Value"=0, "Index"=w819, "Device No."=w818) -> ()  [unwired: 6 in, 3 out]
                  }
                }
              }
            }
            n518 = case shown="True" w769 {
              tunnel: w782 -> [_ w792]
              tunnel: w766 -> [_ w787]
              frame False {
                n519 = local read "Axial Pressure  [KPa]"() -> (→"Axialdruck save":dbl)
              }
              frame True {
                n520 = local read "Axialdruck save"() -> (w790:dbl)
                n521 = local read "Axialpressure"() -> (w786:dbl)
                n522 = case shown="True" w792 {
                  tunnel: "Delta Axial" -> [w802 w806]
                  tunnel: w790 -> [w801 w807]
                  tunnel: [w800 w805] -> w788
                  tunnel: w786 -> [w799 w804]
                  tunnel: [w798 w803] -> w789
                  frame False {
                    n523 = Subtract(x=w801, y=w802) -> (x-y=w800:dbl)
                    n524 = Greater?(x=w800, y=w799) -> (0:w798:bool)
                  }
                  frame True {
                    n525 = Add(x=w807, y=w806) -> (x+y=w805:dbl)
                    n526 = Greater?(x=w804, y=w805) -> (0:w803:bool)
                  }
                }
                n527 = case shown="True" w789 {
                  tunnel: w787 -> [_ w794]
                  frame False {
                  }
                  frame True {
                    w795 = u16 60 items=["NaN", "Kp_Position_Vibro", "Ki_Position_Vibro", "PAR_3", "Sinusfrequenz_preSh", "Zylinder_Move_Button", "PAR_6", "PAR_7", "PAR_8", "PAR_9", "PAR_10", "PAR_11", "PAR_12", "Amplitude_PreSh", "Compass_OFF", "PAR_15", "PAR_16", "SollMoog", "PAR_18", "PAR_19", "PAR_20", "Vibro_Test_Button", "PAR_22", "PAR_23", "PAR_24", "PAR_25", "PAR_26", "PAR_27", "PAR_28", "PAR_29", "PAR_30", "PAR_31", "PAR_32", "Start_Test_Button", "PAR_34", "Programm_counter", "PAR_36", "Circumference_ON_Flag", "PAR_38", "PAR_39", "Pore_Control_Button", "Side_Control_Button", "Axial_Control_Button", "PAR_43", "PAR_44", "PAR_45", "Einfahren_Piston", "PAR_47", "PAR_48", "PAR_49", "PAR_50", "PAR_51", "PAR_52", "PAR_53", "PAR_54", "PAR_55", "PAR_56", "PAR_57", "LinearUpDown_Button", "Linear_Pore_GO", "Linear_Axial_GO", "Linear_Side_GO", "PAR_62", "PAR_63", "PAR_64", "PAR_65", "PAR_66", "PAR_67", "PAR_68", "PAR_69", "Pre_Shearing_Button", "PAR_71", "PAR_72", "PAR_73", "PAR_74", "Circumf_Control_On", "PAR_76", "PAR_77", "PAR_78", "PAR_79", "Modus", "", "", "", "", "", "", "", "", "", "", "", "", "", "", "", "", "", "", "", "", "", "", "", "", "", ""] ("par_enum")
                    n528 = local write "Go - Axialdruck"(FALSE ("Go - Axialdruck")) -> ()
                    n529 = local write "Delta Axial"(0.0 ("Delta Axial")) -> ()
                    n530 = call "ADwin Set_Par.vi"("Value"=0, "Index"=w795, "Device No."=w794) -> ()  [unwired: 6 in, 3 out]
                  }
                }
                n531 = local write "Soll Axial Pressure"(w788) -> ()
              }
            }
          }
          frame #12 {
            # "Pre-Shearing"
            n532 = local read "Duration of Cycle SOLL"() -> (w858:i32)
            n533 = local read "Pre-shearing output"() -> (w860:dbl)
            n534 = local read "Start Pre-Shearing"() -> (w859:bool)
            n535 = local read "Axial Pressure  [KPa]"() -> (w882:dbl)
            n536 = Multiply(x=w858, y="Number of Cycles SOLL") -> (x*y=w857:dbl)
            n537 = local read "Pore Pressure [KPa]"() -> (w878:dbl)
            "Abweichung Pore" <- w878
            n538 = local read "Side Pressure  [KPa]"() -> (w865:dbl)
            "Abweichung Side" <- w865
            n539 = case shown="False" w859 {
              tunnel: w857 -> [_ w893]
              frame False {
                n540 = Tick Count (ms)() -> (millisecond timer value=w886:u32)
                n541 = Divide(x=w886, y=u32 1000) -> (x/y=→"ms Offset Pre-Shearing":dbl)
              }
              frame True {
                n542 = Tick Count (ms)() -> (millisecond timer value=w892:u32)
                n543 = local read "ms Offset Pre-Shearing"() -> (w894:u32)
                n544 = Divide(x=w892, y=u32 1000) -> (x/y=w890:dbl)
                n545 = Subtract(x=w890, y=w894) -> (x-y=w889:dbl)
                "S" <- w889
                n546 = Greater?(x=w889, y=w893) -> (0:w888:bool)
                "Pre-Shearing Ended Successful:" <- w888
                n547 = case shown="True" w888 {
                  frame False {
                  }
                  frame True {
                    n548 = local write "Start Pre-Shearing"(FALSE ("Par_70")) -> ()
                  }
                }
                "Total Elapsed Seconds" <- w893
              }
            }
            n549 = Bundle("Axial Pressure  [KPa]"=w882, "Pre-shearing output"=w860) -> (→"Sollvorgabe":T5)  [unwired: 1 in]
            n550 = Subtract(x="Sollwert Porenwasser", y="Erlaubte  Max Abweichung Pore") -> (x-y=w875:dbl)
            n551 = Add(x="Sollwert Seitendruck", y="Erlaubte Max Abweichung Side") -> (x+y=w868:dbl)
            n552 = Subtract(x="Sollwert Seitendruck", y="Erlaubte Max Abweichung Side") -> (x-y=w869:dbl)
            n553 = Add(x="Sollwert Porenwasser", y="Erlaubte  Max Abweichung Pore") -> (x+y=w874:dbl)
            n554 = Greater?(x=w865, y=w868) -> (0:w870:bool)
            n555 = Less?(x=w865, y=w869) -> (x < y?=w871:bool)
            n556 = Greater?(x=w878, y=w874) -> (0:w876:bool)
            n557 = Less?(x=w878, y=w875) -> (x < y?=w877:bool)
            n558 = Subtract(x=w860, y=w882) -> (x-y=w884:dbl)
            "Abweichung Axial" <- w884
            n559 = Absolute Value(x=w884) -> (abs(x)=w883:dbl)
            n560 = Or(x=w870, y=w871) -> (x .or. y?=w861:bool)
            "Side Alarm" <- w861
            n561 = Greater?(x=w883, y="Erlaubte Max Abweichung Axial") -> (0:w863:bool)
            "Axial Alarm" <- w863
            n562 = Or(x=w876, y=w877) -> (x .or. y?=w862:bool)
            "Pore Alarm" <- w862
            n563 = Compound Arithmetic op=OR(w863, w862, w861) -> (w864:bool)
            n564 = case shown="True" "Reset Alarm" {
              frame False {
              }
              frame True {
                n565 = local write "Alarm Triggered"(FALSE ("result")) -> ()
              }
            }
            n566 = case shown="True" w864 {
              frame False {
              }
              frame True {
                "Alarm Triggered" <- FALSE ("result")
              }
            }
          }
          frame #13 {
            # "End of Test Check"
            n567 = local read "Axial Pressure  [KPa]"() -> (w913:dbl)
            n568 = local read "Side Pressure  [KPa]"() -> (w914:dbl)
            n569 = local read "Pore Pressure [KPa]"() -> (w916:dbl)
            n570 = local read "start penetration"() -> (w899:bool)
            n571 = local read "Position Piston"() -> (w906:dbl)
            n572 = local read "Test Flag"() -> (w907:bool)
            n573 = local read "Turn off BC5"() -> (w904:bool)
            n574 = Less?(x=w913, y=70.0) -> (x < y?=w910:bool)
            "Axial Pressure okay:" <- w910
            n575 = Less?(x=w914, y=70.0) -> (x < y?=w911:bool)
            "Side Pressure okay:" <- w911
            n576 = Less?(x=w916, y=70.0) -> (x < y?=w912:bool)
            "Pore Pressure okay:" <- w912
            n577 = Greater?(x=w906, y=419.0) -> (0:w901:bool)
            n578 = Not(x=w899) -> (.not. x?=w898:bool)
            n579 = Not(x=w904) -> (.not. x?=w902:bool)
            n580 = And(x=w902, y=w901) -> (x .and. y?=w903:bool)
            n581 = Compound Arithmetic op=AND(w898, w907, w912, w911, w910) -> (w908:bool)
            n582 = case shown="False" w903 {
              tunnel: w900 -> [_ w922]
              frame False {
                n583 = property on="Turn off BC5" class="Bool (strict)"("DisabledEnum"=T6."Disabled and Grayed Out" ("Disabled")) -> ()  [unwired: 2 in, 2 out]
              }
              frame True {
                w919 = u16 14 items=["NaN", "Kp_Position_Vibro", "Ki_Position_Vibro", "PAR_3", "Sinusfrequenz_preSh", "Zylinder_Move_Button", "PAR_6", "PAR_7", "PAR_8", "PAR_9", "PAR_10", "PAR_11", "PAR_12", "Amplitude_PreSh", "Compass_OFF", "PAR_15", "PAR_16", "SollMoog", "PAR_18", "PAR_19", "PAR_20", "Vibro_Test_Button", "PAR_22", "PAR_23", "PAR_24", "PAR_25", "PAR_26", "PAR_27", "PAR_28", "PAR_29", "PAR_30", "PAR_31", "PAR_32", "Start_Test_Button", "PAR_34", "Programm_counter", "PAR_36", "Circumference_ON_Flag", "PAR_38", "PAR_39", "Pore_Control_Button", "Side_Control_Button", "Axial_Control_Button", "PAR_43", "PAR_44", "PAR_45", "Einfahren_Piston", "PAR_47", "PAR_48", "PAR_49", "PAR_50", "PAR_51", "PAR_52", "PAR_53", "PAR_54", "PAR_55", "PAR_56", "PAR_57", "LinearUpDown_Button", "Linear_Pore_GO", "Linear_Axial_GO", "Linear_Side_GO", "PAR_62", "PAR_63", "PAR_64", "PAR_65", "PAR_66", "PAR_67", "PAR_68", "PAR_69", "Pre_Shearing_Button", "PAR_71", "PAR_72", "PAR_73", "PAR_74", "Circumf_Control_On", "PAR_76", "PAR_77", "PAR_78", "PAR_79", "Modus", "", "", "", "", "", "", "", "", "", "", "", "", "", "", "", "", "", "", "", "", "", "", "", "", "", ""] ("par_enum")
                n584 = local write "Circumference Control"(FALSE ("Umfangsregelung")) -> ()
                n585 = property on="Turn off BC5" class="Bool (strict)"("DisabledEnum"=T6."Enabled" ("Disabled")) -> ()  [unwired: 2 in, 2 out]
                n586 = call "ADwin Set_Par.vi"("Value"=1, "Index"=w919, "Device No."=w922) -> ()  [unwired: 6 in, 3 out]
              }
            }
            n587 = case shown="True" w908 {
              frame False {
              }
              frame True {
                # "not used at the moment"
              }
            }
          }
        }
        "Record Flag" <- "Record Data"
        "Recording" <- "Record Data"
      }
      event "Reset_left_graph": Value Change {
        n588 = event-data() -> ("NewVal"=w925:bool)  [unwired: 1 in, 5 out]
        n589 = case shown="True" w925 {
          selector: w925 -> [_ w926]
          frame False {
          }
          frame True {
            "reset_flag" <- w926
          }
        }
        n590 = property on="Interner Kraftsensor [MPa]" class="XYGraph (strict)"("Value"=cluster{"Y":dbl[], "Y":dbl[]}[] [{"Y"=[0.0], "Y"=[0.0]}] ("Interner Kraftsensor [MPa]")) -> ()  [unwired: 2 in, 2 out]
      }
      event "Notaus": Value Change {
        w927 = u16 80 items=["NaN", "Kp_Position_Vibro", "Ki_Position_Vibro", "PAR_3", "Sinusfrequenz_preSh", "Zylinder_Move_Button", "PAR_6", "PAR_7", "PAR_8", "PAR_9", "PAR_10", "PAR_11", "PAR_12", "Amplitude_PreSh", "Compass_OFF", "PAR_15", "PAR_16", "SollMoog", "PAR_18", "PAR_19", "PAR_20", "Vibro_Test_Button", "PAR_22", "PAR_23", "PAR_24", "PAR_25", "PAR_26", "PAR_27", "PAR_28", "PAR_29", "PAR_30", "PAR_31", "PAR_32", "Start_Test_Button", "PAR_34", "Programm_counter", "PAR_36", "Circumference_ON_Flag", "PAR_38", "PAR_39", "Pore_Control_Button", "Side_Control_Button", "Axial_Control_Button", "PAR_43", "PAR_44", "PAR_45", "Einfahren_Piston", "PAR_47", "PAR_48", "PAR_49", "PAR_50", "PAR_51", "PAR_52", "PAR_53", "PAR_54", "PAR_55", "PAR_56", "PAR_57", "LinearUpDown_Button", "Linear_Pore_GO", "Linear_Axial_GO", "Linear_Side_GO", "PAR_62", "PAR_63", "PAR_64", "PAR_65", "PAR_66", "PAR_67", "PAR_68", "PAR_69", "Pre_Shearing_Button", "PAR_71", "PAR_72", "PAR_73", "PAR_74", "Circumf_Control_On", "PAR_76", "PAR_77", "PAR_78", "PAR_79", "Modus", "", "", "", "", "", "", "", "", "", "", "", "", "", "", "", "", "", "", "", "", "", "", "", "", "", ""] ("par_enum")
        # "Sets Adiwn State to Cancel all ongoing tasks and quit program"
        n591 = event-data() -> ("NewVal"=w930:bool)  [unwired: 1 in, 5 out]
        "Notaus Activ" <- w930
        n592 = call "ADwin Set_Par.vi"("Value"=10, "Index"=w927, "Device No."=w928) -> ()  [unwired: 6 in, 3 out]
      }
      event "SET Pump Offsets": Value Change {
        (unwired) "Modification done by zhengyu chen, if measured side, pore and axial pressure is less than default\nvalues, we force them to be default values. "
        n593 = event-data() -> ()  [unwired: 1 in, 6 out]
        n594 = call "ADwin Get_FPar_Block.vi"("count"=i16 80, "startindex"=i16 1, "Device No."=w934) -> ("Data"=w953:sgl[])  [unwired: 2 in, 3 out]
        n595 = Decrement(x=T10."SidePressOffset" ("Enum")) -> (x-1=w956:T10)
        n596 = Decrement(x=T10."AxialPressOffset" ("Enum")) -> (x-1=w955:T10)
        n597 = Decrement(x=T10."PorePressOffset" ("Enum")) -> (x-1=w954:T10)
        n598 = Index Array(array=w953, index=w956) -> (element=w949:sgl)
        n599 = Greater?(x=w949, y="Side Offset Soll") -> (0:w960:bool)
        n600 = Index Array(array=w953, index=w955) -> (element=w941:sgl)
        n601 = Greater?(x=w941, y="Axial Offset Soll") -> (0:w946:bool)
        n602 = Index Array(array=w953, index=w954) -> (element=w938:sgl)
        n603 = Greater?(x=w938, y="Pore Offset SOLL") -> (0:w939:bool)
        n604 = case shown="False" w946 {
          tunnel: w934 -> [w969 w973]
          tunnel: [w969 w973] -> w944
          tunnel: "Axial Offset Soll" -> [w970 _]
          tunnel: [w970 w971] -> w942
          tunnel: T10."AxialPressOffset" ("Enum") -> [w968 w972]
          tunnel: [w968 w972] -> w943
          tunnel: w941 -> [_ w971]
          frame False {
          }
          frame True {
          }
        }
        n605 = case shown="False" w960 {
          tunnel: w934 -> [w975 w979]
          tunnel: [w975 w979] -> w961
          tunnel: "Side Offset Soll" -> [w976 _]
          tunnel: [w976 w977] -> w947
          tunnel: T10."SidePressOffset" ("Enum") -> [w974 w978]
          tunnel: [w974 w978] -> w948
          tunnel: w949 -> [_ w977]
          frame False {
          }
          frame True {
          }
        }
        n606 = case shown="False" w939 {
          tunnel: w934 -> [w963 w967]
          tunnel: [w963 w967] -> w937
          tunnel: "Pore Offset SOLL" -> [w964 _]
          tunnel: [w964 w965] -> w935
          tunnel: T10."PorePressOffset" ("Enum") -> [w962 w966]
          tunnel: [w962 w966] -> w936
          tunnel: w938 -> [_ w965]
          frame False {
          }
          frame True {
          }
        }
        n607 = call "ADwin Set_FPar.vi"("Value"=w947, "Index"=w948, "Device No."=w961) -> ()  [unwired: 6 in, 3 out]
        n608 = call "ADwin Set_FPar.vi"("Value"=w942, "Index"=w943, "Device No."=w944) -> ()  [unwired: 6 in, 3 out]
        n609 = call "ADwin Set_FPar.vi"("Value"=w935, "Index"=w936, "Device No."=w937) -> ()  [unwired: 6 in, 3 out]
      }
      event "SET Pump Controls": Value Change {
        n610 = event-data() -> ()  [unwired: 1 in, 6 out]
        n611 = call "ADwin Set_FPar.vi"("Value"="Kpp", "Index"=T10."Kp_Porepress" ("Enum"), "Device No."=w986) -> ("Device No. out"=w997:u16)  [unwired: 6 in, 2 out]
        n612 = call "ADwin Set_FPar.vi"("Value"="Kip", "Index"=T10."Ki_Porepress" ("Enum"), "Device No."=w997) -> ("Device No. out"=w993:u16)  [unwired: 6 in, 2 out]
        n613 = call "ADwin Set_FPar.vi"("Value"="Kps", "Index"=T10."Kp_Sidepress" ("Enum"), "Device No."=w993) -> ("Device No. out"=w994:u16)  [unwired: 6 in, 2 out]
        n614 = call "ADwin Set_FPar.vi"("Value"="Kis", "Index"=T10."Ki_Sidepress" ("Enum"), "Device No."=w994) -> ("Device No. out"=w995:u16)  [unwired: 6 in, 2 out]
        n615 = call "ADwin Set_FPar.vi"("Value"="Kpa", "Index"=T10."Kp_Axialpress" ("Enum"), "Device No."=w995) -> ("Device No. out"=w996:u16)  [unwired: 6 in, 2 out]
        n616 = call "ADwin Set_FPar.vi"("Value"="Kia", "Index"=T10."Ki_Axialpress" ("Enum"), "Device No."=w996) -> ()  [unwired: 6 in, 3 out]
      }
      event "Turn off BC5": Value Change {
        n617 = event-data() -> ("NewVal"=w998:bool)  [unwired: 1 in, 5 out]
        n618 = case shown="True" w998 {
          tunnel: w999 -> [_ w1001]
          frame False {
          }
          frame True {
            w1000 = u16 14 items=["NaN", "Kp_Position_Vibro", "Ki_Position_Vibro", "PAR_3", "Sinusfrequenz_preSh", "Zylinder_Move_Button", "PAR_6", "PAR_7", "PAR_8", "PAR_9", "PAR_10", "PAR_11", "PAR_12", "Amplitude_PreSh", "Compass_OFF", "PAR_15", "PAR_16", "SollMoog", "PAR_18", "PAR_19", "PAR_20", "Vibro_Test_Button", "PAR_22", "PAR_23", "PAR_24", "PAR_25", "PAR_26", "PAR_27", "PAR_28", "PAR_29", "PAR_30", "PAR_31", "PAR_32", "Start_Test_Button", "PAR_34", "Programm_counter", "PAR_36", "Circumference_ON_Flag", "PAR_38", "PAR_39", "Pore_Control_Button", "Side_Control_Button", "Axial_Control_Button", "PAR_43", "PAR_44", "PAR_45", "Einfahren_Piston", "PAR_47", "PAR_48", "PAR_49", "PAR_50", "PAR_51", "PAR_52", "PAR_53", "PAR_54", "PAR_55", "PAR_56", "PAR_57", "LinearUpDown_Button", "Linear_Pore_GO", "Linear_Axial_GO", "Linear_Side_GO", "PAR_62", "PAR_63", "PAR_64", "PAR_65", "PAR_66", "PAR_67", "PAR_68", "PAR_69", "Pre_Shearing_Button", "PAR_71", "PAR_72", "PAR_73", "PAR_74", "Circumf_Control_On", "PAR_76", "PAR_77", "PAR_78", "PAR_79", "Modus", "", "", "", "", "", "", "", "", "", "", "", "", "", "", "", "", "", "", "", "", "", "", "", "", "", ""] ("par_enum")
            n619 = call "ADwin Set_Par.vi"("Value"=0, "Index"=w1000, "Device No."=w1001) -> ()  [unwired: 6 in, 3 out]
          }
        }
      }
      event "Circumference Control": Value Change {
        w1003 = u16 75 items=["NaN", "Kp_Position_Vibro", "Ki_Position_Vibro", "PAR_3", "Sinusfrequenz_preSh", "Zylinder_Move_Button", "PAR_6", "PAR_7", "PAR_8", "PAR_9", "PAR_10", "PAR_11", "PAR_12", "Amplitude_PreSh", "Compass_OFF", "PAR_15", "PAR_16", "SollMoog", "PAR_18", "PAR_19", "PAR_20", "Vibro_Test_Button", "PAR_22", "PAR_23", "PAR_24", "PAR_25", "PAR_26", "PAR_27", "PAR_28", "PAR_29", "PAR_30", "PAR_31", "PAR_32", "Start_Test_Button", "PAR_34", "Programm_counter", "PAR_36", "Circumference_ON_Flag", "PAR_38", "PAR_39", "Pore_Control_Button", "Side_Control_Button", "Axial_Control_Button", "PAR_43", "PAR_44", "PAR_45", "Einfahren_Piston", "PAR_47", "PAR_48", "PAR_49", "PAR_50", "PAR_51", "PAR_52", "PAR_53", "PAR_54", "PAR_55", "PAR_56", "PAR_57", "LinearUpDown_Button", "Linear_Pore_GO", "Linear_Axial_GO", "Linear_Side_GO", "PAR_62", "PAR_63", "PAR_64", "PAR_65", "PAR_66", "PAR_67", "PAR_68", "PAR_69", "Pre_Shearing_Button", "PAR_71", "PAR_72", "PAR_73", "PAR_74", "Circumf_Control_On", "PAR_76", "PAR_77", "PAR_78", "PAR_79", "Modus", "", "", "", "", "", "", "", "", "", "", "", "", "", "", "", "", "", "", "", "", "", "", "", "", "", ""] ("par_enum")
        n620 = event-data() -> ("NewVal"=w1005:bool)  [unwired: 1 in, 5 out]
        n621 = Select(t=1 ("Value"), s=w1005, f=0 ("Value")) -> (s? t:f=w1008:i32)
        n622 = case shown="True" w1005 {
          tunnel: w1004 -> [_ w1010]
          frame False {
          }
          frame True {
            w1009 = u16 37 items=["NaN", "Kp_Position_Vibro", "Ki_Position_Vibro", "PAR_3", "Sinusfrequenz_preSh", "Zylinder_Move_Button", "PAR_6", "PAR_7", "PAR_8", "PAR_9", "PAR_10", "PAR_11", "PAR_12", "Amplitude_PreSh", "Compass_OFF", "PAR_15", "PAR_16", "SollMoog", "PAR_18", "PAR_19", "PAR_20", "Vibro_Test_Button", "PAR_22", "PAR_23", "PAR_24", "PAR_25", "PAR_26", "PAR_27", "PAR_28", "PAR_29", "PAR_30", "PAR_31", "PAR_32", "Start_Test_Button", "PAR_34", "Programm_counter", "PAR_36", "Circumference_ON_Flag", "PAR_38", "PAR_39", "Pore_Control_Button", "Side_Control_Button", "Axial_Control_Button", "PAR_43", "PAR_44", "PAR_45", "Einfahren_Piston", "PAR_47", "PAR_48", "PAR_49", "PAR_50", "PAR_51", "PAR_52", "PAR_53", "PAR_54", "PAR_55", "PAR_56", "PAR_57", "LinearUpDown_Button", "Linear_Pore_GO", "Linear_Axial_GO", "Linear_Side_GO", "PAR_62", "PAR_63", "PAR_64", "PAR_65", "PAR_66", "PAR_67", "PAR_68", "PAR_69", "Pre_Shearing_Button", "PAR_71", "PAR_72", "PAR_73", "PAR_74", "Circumf_Control_On", "PAR_76", "PAR_77", "PAR_78", "PAR_79", "Modus", "", "", "", "", "", "", "", "", "", "", "", "", "", "", "", "", "", "", "", "", "", "", "", "", "", ""] ("par_enum")
            n623 = call "ADwin Set_Par.vi"("Value"=1, "Index"=w1009, "Device No."=w1010) -> ()  [unwired: 6 in, 3 out]
          }
        }
        n624 = call "ADwin Set_Par.vi"("Value"=w1008, "Index"=w1003, "Device No."=w1004) -> ()  [unwired: 6 in, 3 out]
      }
      event "Up_Lower": Value Change {
        w1012 = u16 58 items=["NaN", "Kp_Position_Vibro", "Ki_Position_Vibro", "PAR_3", "Sinusfrequenz_preSh", "Zylinder_Move_Button", "PAR_6", "PAR_7", "PAR_8", "PAR_9", "PAR_10", "PAR_11", "PAR_12", "Amplitude_PreSh", "Compass_OFF", "PAR_15", "PAR_16", "SollMoog", "PAR_18", "PAR_19", "PAR_20", "Vibro_Test_Button", "PAR_22", "PAR_23", "PAR_24", "PAR_25", "PAR_26", "PAR_27", "PAR_28", "PAR_29", "PAR_30", "PAR_31", "PAR_32", "Start_Test_Button", "PAR_34", "Programm_counter", "PAR_36", "Circumference_ON_Flag", "PAR_38", "PAR_39", "Pore_Control_Button", "Side_Control_Button", "Axial_Control_Button", "PAR_43", "PAR_44", "PAR_45", "Einfahren_Piston", "PAR_47", "PAR_48", "PAR_49", "PAR_50", "PAR_51", "PAR_52", "PAR_53", "PAR_54", "PAR_55", "PAR_56", "PAR_57", "LinearUpDown_Button", "Linear_Pore_GO", "Linear_Axial_GO", "Linear_Side_GO", "PAR_62", "PAR_63", "PAR_64", "PAR_65", "PAR_66", "PAR_67", "PAR_68", "PAR_69", "Pre_Shearing_Button", "PAR_71", "PAR_72", "PAR_73", "PAR_74", "Circumf_Control_On", "PAR_76", "PAR_77", "PAR_78", "PAR_79", "Modus", "", "", "", "", "", "", "", "", "", "", "", "", "", "", "", "", "", "", "", "", "", "", "", "", "", ""] ("par_enum")
        n625 = event-data() -> ()  [unwired: 1 in, 6 out]
        n626 = Select(t=1 ("Value"), s="Up_Lower", f=0 ("Value")) -> (s? t:f=w1014:i32)
        n627 = call "ADwin Set_Par.vi"("Value"=w1014, "Index"=w1012, "Device No."=w1013) -> ()  [unwired: 6 in, 3 out]
      }
      event "Go - Porendruck": Value Change {
        n628 = event-data() -> ()  [unwired: 1 in, 6 out]
        n629 = flat-sequence {
          tunnel: w1020 -> [w1021]
          tunnel: [w1029] -> w1019
          tunnel: [w1023] -> w1018
          tunnel: w1019 -> [w1046]
          tunnel: w1018 -> [w1051]
          frame #0 {
            w1025 = u16 58 items=["NaN", "Kp_Position_Vibro", "Ki_Position_Vibro", "PAR_3", "Sinusfrequenz_preSh", "Zylinder_Move_Button", "PAR_6", "PAR_7", "PAR_8", "PAR_9", "PAR_10", "PAR_11", "PAR_12", "Amplitude_PreSh", "Compass_OFF", "PAR_15", "PAR_16", "SollMoog", "PAR_18", "PAR_19", "PAR_20", "Vibro_Test_Button", "PAR_22", "PAR_23", "PAR_24", "PAR_25", "PAR_26", "PAR_27", "PAR_28", "PAR_29", "PAR_30", "PAR_31", "PAR_32", "Start_Test_Button", "PAR_34", "Programm_counter", "PAR_36", "Circumference_ON_Flag", "PAR_38", "PAR_39", "Pore_Control_Button", "Side_Control_Button", "Axial_Control_Button", "PAR_43", "PAR_44", "PAR_45", "Einfahren_Piston", "PAR_47", "PAR_48", "PAR_49", "PAR_50", "PAR_51", "PAR_52", "PAR_53", "PAR_54", "PAR_55", "PAR_56", "PAR_57", "LinearUpDown_Button", "Linear_Pore_GO", "Linear_Axial_GO", "Linear_Side_GO", "PAR_62", "PAR_63", "PAR_64", "PAR_65", "PAR_66", "PAR_67", "PAR_68", "PAR_69", "Pre_Shearing_Button", "PAR_71", "PAR_72", "PAR_73", "PAR_74", "Circumf_Control_On", "PAR_76", "PAR_77", "PAR_78", "PAR_79", "Modus", "", "", "", "", "", "", "", "", "", "", "", "", "", "", "", "", "", "", "", "", "", "", "", "", "", ""] ("par_enum")
            # "Pro Minute"
            n630 = local read "GO All Pressure"() -> (w1038:bool)
            n631 = local read "Velocity Linear"() -> (w1030:dbl)
            n632 = local read "Delta Pore"() -> (w1042:dbl)
            n633 = local read "Up_Lower"() -> (w1022:bool)
            n634 = Or(x="Go - Porendruck", y=w1038) -> (x .or. y?=w1039:bool)
            n635 = Multiply(x=5000.0 ("y"), y=60.0) -> (x*y=w1036:dbl)
            n636 = Greater?(x=w1042, y=0.0) -> (0:w1040:bool)
            n637 = Divide(x=5.4613, y=w1036) -> (x/y=w1037:dbl)
            n638 = And(x=w1039, y=w1040) -> (x .and. y?=w1029:bool)
            n639 = case shown="True" w1029 {
              selector: w1029 -> [_ w1044]
              frame False {
              }
              frame True {
                n640 = local write "Regelung Akiv Porepress"(w1044) -> ()
              }
            }
            n641 = Multiply(x=w1030, y=w1037) -> (x*y=w1033:dbl)
            n642 = local write "Go - Porendruck"(w1029) -> ()
            n643 = Select(t=1 ("Value"), s=w1022, f=0 ("Value")) -> (s? t:f=w1026:i32)
            n644 = call "ADwin Set_Par.vi"("Value"=w1026, "Index"=w1025, "Device No."=w1021) -> ("Device No. out"=w1024:u16)  [unwired: 6 in, 2 out]
            n645 = call "ADwin Set_FPar.vi"("Value"=w1033, "Index"=T10."PaProMin" ("Enum"), "Device No."=w1024) -> ("Device No. out"=w1023:u16)  [unwired: 6 in, 2 out]
          }
          frame #1 {
            w1050 = u16 40 items=["NaN", "Kp_Position_Vibro", "Ki_Position_Vibro", "PAR_3", "Sinusfrequenz_preSh", "Zylinder_Move_Button", "PAR_6", "PAR_7", "PAR_8", "PAR_9", "PAR_10", "PAR_11", "PAR_12", "Amplitude_PreSh", "Compass_OFF", "PAR_15", "PAR_16", "SollMoog", "PAR_18", "PAR_19", "PAR_20", "Vibro_Test_Button", "PAR_22", "PAR_23", "PAR_24", "PAR_25", "PAR_26", "PAR_27", "PAR_28", "PAR_29", "PAR_30", "PAR_31", "PAR_32", "Start_Test_Button", "PAR_34", "Programm_counter", "PAR_36", "Circumference_ON_Flag", "PAR_38", "PAR_39", "Pore_Control_Button", "Side_Control_Button", "Axial_Control_Button", "PAR_43", "PAR_44", "PAR_45", "Einfahren_Piston", "PAR_47", "PAR_48", "PAR_49", "PAR_50", "PAR_51", "PAR_52", "PAR_53", "PAR_54", "PAR_55", "PAR_56", "PAR_57", "LinearUpDown_Button", "Linear_Pore_GO", "Linear_Axial_GO", "Linear_Side_GO", "PAR_62", "PAR_63", "PAR_64", "PAR_65", "PAR_66", "PAR_67", "PAR_68", "PAR_69", "Pre_Shearing_Button", "PAR_71", "PAR_72", "PAR_73", "PAR_74", "Circumf_Control_On", "PAR_76", "PAR_77", "PAR_78", "PAR_79", "Modus", "", "", "", "", "", "", "", "", "", "", "", "", "", "", "", "", "", "", "", "", "", "", "", "", "", ""] ("par_enum")
            w1055 = u16 59 items=["NaN", "Kp_Position_Vibro", "Ki_Position_Vibro", "PAR_3", "Sinusfrequenz_preSh", "Zylinder_Move_Button", "PAR_6", "PAR_7", "PAR_8", "PAR_9", "PAR_10", "PAR_11", "PAR_12", "Amplitude_PreSh", "Compass_OFF", "PAR_15", "PAR_16", "SollMoog", "PAR_18", "PAR_19", "PAR_20", "Vibro_Test_Button", "PAR_22", "PAR_23", "PAR_24", "PAR_25", "PAR_26", "PAR_27", "PAR_28", "PAR_29", "PAR_30", "PAR_31", "PAR_32", "Start_Test_Button", "PAR_34", "Programm_counter", "PAR_36", "Circumference_ON_Flag", "PAR_38", "PAR_39", "Pore_Control_Button", "Side_Control_Button", "Axial_Control_Button", "PAR_43", "PAR_44", "PAR_45", "Einfahren_Piston", "PAR_47", "PAR_48", "PAR_49", "PAR_50", "PAR_51", "PAR_52", "PAR_53", "PAR_54", "PAR_55", "PAR_56", "PAR_57", "LinearUpDown_Button", "Linear_Pore_GO", "Linear_Axial_GO", "Linear_Side_GO", "PAR_62", "PAR_63", "PAR_64", "PAR_65", "PAR_66", "PAR_67", "PAR_68", "PAR_69", "Pre_Shearing_Button", "PAR_71", "PAR_72", "PAR_73", "PAR_74", "Circumf_Control_On", "PAR_76", "PAR_77", "PAR_78", "PAR_79", "Modus", "", "", "", "", "", "", "", "", "", "", "", "", "", "", "", "", "", "", "", "", "", "", "", "", "", ""] ("par_enum")
            n646 = Select(t=1 ("Value"), s=w1046, f=0 ("Value")) -> (s? t:f=w1054:i32)
            n647 = Select(t=1 ("Value"), s=w1046, f=0 ("Value")) -> (s? t:f=w1049:i32)
            n648 = call "ADwin Set_Par.vi"("Value"=w1054, "Index"=w1055, "Device No."=w1051) -> ("Device No. out"=w1045:u16)  [unwired: 6 in, 2 out]
            n649 = call "ADwin Set_Par.vi"("Value"=w1049, "Index"=w1050, "Device No."=w1045) -> ()  [unwired: 6 in, 3 out]
          }
        }
      }
      event "GO All Pressure": Value Change {
        n650 = event-data() -> ()  [unwired: 1 in, 6 out]
        n651 = case shown="True" "GO All Pressure" {
          selector: "GO All Pressure" -> [_ w1057]
          frame False {
          }
          frame True {
            n652 = flat-sequence {
              tunnel: w1057 -> [_]
              frame #0 {
                n653 = local read "Delta Seiten"() -> (w1063:dbl)
                n654 = local read "Delta Pore"() -> (w1066:dbl)
                n655 = local read "Delta Axial"() -> (w1060:dbl)
                n656 = Greater?(x=w1066, y=0.0) -> (0:w1065:bool)
                n657 = Greater?(x=w1063, y=0.0) -> (0:w1062:bool)
                n658 = Greater?(x=w1060, y=0.0) -> (0:w1059:bool)
                n659 = case shown="True" w1065 {
                  selector: w1065 -> [_ w1069]
                  frame False {
                  }
                  frame True {
                    n660 = property on="Go - Porendruck" class="Bool (strict)"("Val(Sgnl)"=w1069) -> ()  [unwired: 2 in, 2 out]
                  }
                }
                n661 = case shown="True" w1062 {
                  selector: w1062 -> [_ w1068]
                  frame False {
                  }
                  frame True {
                    n662 = property on="Go - Seitendruck" class="Bool (strict)"("Val(Sgnl)"=w1068) -> ()  [unwired: 2 in, 2 out]
                  }
                }
                n663 = case shown="True" w1059 {
                  selector: w1059 -> [_ w1067]
                  frame False {
                  }
                  frame True {
                    n664 = property on="Go - Axialdruck" class="Bool (strict)"("Val(Sgnl)"=w1067) -> ()  [unwired: 2 in, 2 out]
                  }
                }
              }
              frame #1 {
                n665 = local write "GO All Pressure"(FALSE ("GO All Pressure")) -> ()
              }
            }
          }
        }
      }
      event "Go - Axialdruck": Value Change {
        n666 = event-data() -> ()  [unwired: 1 in, 6 out]
        n667 = flat-sequence {
          tunnel: w1073 -> [w1074]
          tunnel: [w1082] -> w1072
          tunnel: [w1075] -> w1071
          tunnel: w1072 -> [w1099]
          tunnel: w1071 -> [w1104]
          frame #0 {
            w1078 = u16 58 items=["NaN", "Kp_Position_Vibro", "Ki_Position_Vibro", "PAR_3", "Sinusfrequenz_preSh", "Zylinder_Move_Button", "PAR_6", "PAR_7", "PAR_8", "PAR_9", "PAR_10", "PAR_11", "PAR_12", "Amplitude_PreSh", "Compass_OFF", "PAR_15", "PAR_16", "SollMoog", "PAR_18", "PAR_19", "PAR_20", "Vibro_Test_Button", "PAR_22", "PAR_23", "PAR_24", "PAR_25", "PAR_26", "PAR_27", "PAR_28", "PAR_29", "PAR_30", "PAR_31", "PAR_32", "Start_Test_Button", "PAR_34", "Programm_counter", "PAR_36", "Circumference_ON_Flag", "PAR_38", "PAR_39", "Pore_Control_Button", "Side_Control_Button", "Axial_Control_Button", "PAR_43", "PAR_44", "PAR_45", "Einfahren_Piston", "PAR_47", "PAR_48", "PAR_49", "PAR_50", "PAR_51", "PAR_52", "PAR_53", "PAR_54", "PAR_55", "PAR_56", "PAR_57", "LinearUpDown_Button", "Linear_Pore_GO", "Linear_Axial_GO", "Linear_Side_GO", "PAR_62", "PAR_63", "PAR_64", "PAR_65", "PAR_66", "PAR_67", "PAR_68", "PAR_69", "Pre_Shearing_Button", "PAR_71", "PAR_72", "PAR_73", "PAR_74", "Circumf_Control_On", "PAR_76", "PAR_77", "PAR_78", "PAR_79", "Modus", "", "", "", "", "", "", "", "", "", "", "", "", "", "", "", "", "", "", "", "", "", "", "", "", "", ""] ("par_enum")
            # "Entspricht 1 kPa"
            # "5000 Hz Programm"
            # "Pro Minute"
            n668 = local read "GO All Pressure"() -> (w1096:bool)
            n669 = local read "Delta Axial"() -> (w1093:dbl)
            n670 = Or(x="Go - Axialdruck", y=w1096) -> (x .or. y?=w1091:bool)
            n671 = Greater?(x=w1093, y=0.0) -> (0:w1092:bool)
            n672 = And(x=w1091, y=w1092) -> (x .and. y?=w1082:bool)
            n673 = local write "Go - Axialdruck"(w1082) -> ()
            n674 = Multiply(x=5000.0 ("y"), y=60.0) -> (x*y=w1089:dbl)
            n675 = case shown="True" w1082 {
              selector: w1082 -> [_ w1097]
              frame False {
              }
              frame True {
                n676 = local write "Regelung Akiv Axial"(w1097) -> ()
              }
            }
            n677 = Divide(x=5.4613, y=w1089) -> (x/y=w1090:dbl)
            n678 = local read "Up_Lower"() -> (w1076:bool)
            n679 = Multiply(x="Velocity Linear", y=w1090) -> (x*y=w1085:dbl)
            n680 = Select(t=1 ("Value"), s=w1076, f=0 ("Value")) -> (s? t:f=w1079:i32)
            n681 = call "ADwin Set_Par.vi"("Value"=w1079, "Index"=w1078, "Device No."=w1074) -> ("Device No. out"=w1077:u16)  [unwired: 6 in, 2 out]
            n682 = call "ADwin Set_FPar.vi"("Value"=w1085, "Index"=T10."PaProMin" ("Enum"), "Device No."=w1077) -> ("Device No. out"=w1075:u16)  [unwired: 6 in, 2 out]
          }
          frame #1 {
            w1103 = u16 42 items=["NaN", "Kp_Position_Vibro", "Ki_Position_Vibro", "PAR_3", "Sinusfrequenz_preSh", "Zylinder_Move_Button", "PAR_6", "PAR_7", "PAR_8", "PAR_9", "PAR_10", "PAR_11", "PAR_12", "Amplitude_PreSh", "Compass_OFF", "PAR_15", "PAR_16", "SollMoog", "PAR_18", "PAR_19", "PAR_20", "Vibro_Test_Button", "PAR_22", "PAR_23", "PAR_24", "PAR_25", "PAR_26", "PAR_27", "PAR_28", "PAR_29", "PAR_30", "PAR_31", "PAR_32", "Start_Test_Button", "PAR_34", "Programm_counter", "PAR_36", "Circumference_ON_Flag", "PAR_38", "PAR_39", "Pore_Control_Button", "Side_Control_Button", "Axial_Control_Button", "PAR_43", "PAR_44", "PAR_45", "Einfahren_Piston", "PAR_47", "PAR_48", "PAR_49", "PAR_50", "PAR_51", "PAR_52", "PAR_53", "PAR_54", "PAR_55", "PAR_56", "PAR_57", "LinearUpDown_Button", "Linear_Pore_GO", "Linear_Axial_GO", "Linear_Side_GO", "PAR_62", "PAR_63", "PAR_64", "PAR_65", "PAR_66", "PAR_67", "PAR_68", "PAR_69", "Pre_Shearing_Button", "PAR_71", "PAR_72", "PAR_73", "PAR_74", "Circumf_Control_On", "PAR_76", "PAR_77", "PAR_78", "PAR_79", "Modus", "", "", "", "", "", "", "", "", "", "", "", "", "", "", "", "", "", "", "", "", "", "", "", "", "", ""] ("par_enum")
            w1108 = u16 60 items=["NaN", "Kp_Position_Vibro", "Ki_Position_Vibro", "PAR_3", "Sinusfrequenz_preSh", "Zylinder_Move_Button", "PAR_6", "PAR_7", "PAR_8", "PAR_9", "PAR_10", "PAR_11", "PAR_12", "Amplitude_PreSh", "Compass_OFF", "PAR_15", "PAR_16", "SollMoog", "PAR_18", "PAR_19", "PAR_20", "Vibro_Test_Button", "PAR_22", "PAR_23", "PAR_24", "PAR_25", "PAR_26", "PAR_27", "PAR_28", "PAR_29", "PAR_30", "PAR_31", "PAR_32", "Start_Test_Button", "PAR_34", "Programm_counter", "PAR_36", "Circumference_ON_Flag", "PAR_38", "PAR_39", "Pore_Control_Button", "Side_Control_Button", "Axial_Control_Button", "PAR_43", "PAR_44", "PAR_45", "Einfahren_Piston", "PAR_47", "PAR_48", "PAR_49", "PAR_50", "PAR_51", "PAR_52", "PAR_53", "PAR_54", "PAR_55", "PAR_56", "PAR_57", "LinearUpDown_Button", "Linear_Pore_GO", "Linear_Axial_GO", "Linear_Side_GO", "PAR_62", "PAR_63", "PAR_64", "PAR_65", "PAR_66", "PAR_67", "PAR_68", "PAR_69", "Pre_Shearing_Button", "PAR_71", "PAR_72", "PAR_73", "PAR_74", "Circumf_Control_On", "PAR_76", "PAR_77", "PAR_78", "PAR_79", "Modus", "", "", "", "", "", "", "", "", "", "", "", "", "", "", "", "", "", "", "", "", "", "", "", "", "", ""] ("par_enum")
            n683 = Select(t=1 ("Value"), s=w1099, f=0 ("Value")) -> (s? t:f=w1107:i32)
            n684 = Select(t=1 ("Value"), s=w1099, f=0 ("Value")) -> (s? t:f=w1102:i32)
            n685 = call "ADwin Set_Par.vi"("Value"=w1107, "Index"=w1108, "Device No."=w1104) -> ("Device No. out"=w1100:u16)  [unwired: 6 in, 2 out]
            n686 = call "ADwin Set_Par.vi"("Value"=w1102, "Index"=w1103, "Device No."=w1100) -> ()  [unwired: 6 in, 3 out]
          }
        }
      }
      event "Velocity Linear": Value Change {
        # "5000 Hz Programm"
        # "Pro Minute"
        n687 = event-data() -> ("NewVal"=w1110:dbl)  [unwired: 1 in, 5 out]
        n688 = Multiply(x=5000.0 ("y"), y=60.0) -> (x*y=w1116:dbl)
        n689 = Divide(x=5.4613, y=w1116) -> (x/y=w1117:dbl)
        n690 = Multiply(x=w1110, y=w1117) -> (x*y=w1113:dbl)
        n691 = call "ADwin Set_FPar.vi"("Value"=w1113, "Index"=T10."PaProMin" ("Enum"), "Device No."=w1109) -> ()  [unwired: 6 in, 3 out]
      }
      event "Go - Seitendruck": Value Change {
        n692 = event-data() -> ()  [unwired: 1 in, 6 out]
        n693 = flat-sequence {
          tunnel: w1120 -> [w1122]
          tunnel: [w1124] -> w1119
          tunnel: [w1121] -> w1118
          tunnel: w1119 -> [w1151]
          tunnel: w1118 -> [w1146]
          frame #0 {
            w1126 = u16 58 items=["NaN", "Kp_Position_Vibro", "Ki_Position_Vibro", "PAR_3", "Sinusfrequenz_preSh", "Zylinder_Move_Button", "PAR_6", "PAR_7", "PAR_8", "PAR_9", "PAR_10", "PAR_11", "PAR_12", "Amplitude_PreSh", "Compass_OFF", "PAR_15", "PAR_16", "SollMoog", "PAR_18", "PAR_19", "PAR_20", "Vibro_Test_Button", "PAR_22", "PAR_23", "PAR_24", "PAR_25", "PAR_26", "PAR_27", "PAR_28", "PAR_29", "PAR_30", "PAR_31", "PAR_32", "Start_Test_Button", "PAR_34", "Programm_counter", "PAR_36", "Circumference_ON_Flag", "PAR_38", "PAR_39", "Pore_Control_Button", "Side_Control_Button", "Axial_Control_Button", "PAR_43", "PAR_44", "PAR_45", "Einfahren_Piston", "PAR_47", "PAR_48", "PAR_49", "PAR_50", "PAR_51", "PAR_52", "PAR_53", "PAR_54", "PAR_55", "PAR_56", "PAR_57", "LinearUpDown_Button", "Linear_Pore_GO", "Linear_Axial_GO", "Linear_Side_GO", "PAR_62", "PAR_63", "PAR_64", "PAR_65", "PAR_66", "PAR_67", "PAR_68", "PAR_69", "Pre_Shearing_Button", "PAR_71", "PAR_72", "PAR_73", "PAR_74", "Circumf_Control_On", "PAR_76", "PAR_77", "PAR_78", "PAR_79", "Modus", "", "", "", "", "", "", "", "", "", "", "", "", "", "", "", "", "", "", "", "", "", "", "", "", "", ""] ("par_enum")
            # "5000 Hz Programm"
            # "Pro Minute"
            n694 = local read "GO All Pressure"() -> (w1138:bool)
            n695 = local read "Delta Seiten"() -> (w1140:dbl)
            n696 = Or(x="Go - Seitendruck", y=w1138) -> (x .or. y?=w1142:bool)
            n697 = local read "Velocity Linear"() -> (w1130:dbl)
            n698 = Greater?(x=w1140, y=0.0) -> (0:w1139:bool)
            n699 = And(x=w1142, y=w1139) -> (x .and. y?=w1121:bool)
            n700 = local write "Go - Seitendruck"(w1121) -> ()
            n701 = case shown="True" w1121 {
              selector: w1121 -> [_ w1144]
              frame False {
              }
              frame True {
                n702 = local write "Regelung Akiv Sidepressure"(w1144) -> ()
              }
            }
            n703 = Multiply(x=5000.0 ("y"), y=60.0) -> (x*y=w1136:dbl)
            n704 = Divide(x=5.4613, y=w1136) -> (x/y=w1137:dbl)
            n705 = local read "Up_Lower"() -> (w1123:bool)
            n706 = Multiply(x=w1130, y=w1137) -> (x*y=w1133:dbl)
            n707 = Select(t=1 ("Value"), s=w1123, f=0 ("Value")) -> (s? t:f=w1127:i32)
            n708 = call "ADwin Set_Par.vi"("Value"=w1127, "Index"=w1126, "Device No."=w1122) -> ("Device No. out"=w1125:u16)  [unwired: 6 in, 2 out]
            n709 = call "ADwin Set_FPar.vi"("Value"=w1133, "Index"=T10."PaProMin" ("Enum"), "Device No."=w1125) -> ("Device No. out"=w1124:u16)  [unwired: 6 in, 2 out]
          }
          frame #1 {
            w1148 = u16 41 items=["NaN", "Kp_Position_Vibro", "Ki_Position_Vibro", "PAR_3", "Sinusfrequenz_preSh", "Zylinder_Move_Button", "PAR_6", "PAR_7", "PAR_8", "PAR_9", "PAR_10", "PAR_11", "PAR_12", "Amplitude_PreSh", "Compass_OFF", "PAR_15", "PAR_16", "SollMoog", "PAR_18", "PAR_19", "PAR_20", "Vibro_Test_Button", "PAR_22", "PAR_23", "PAR_24", "PAR_25", "PAR_26", "PAR_27", "PAR_28", "PAR_29", "PAR_30", "PAR_31", "PAR_32", "Start_Test_Button", "PAR_34", "Programm_counter", "PAR_36", "Circumference_ON_Flag", "PAR_38", "PAR_39", "Pore_Control_Button", "Side_Control_Button", "Axial_Control_Button", "PAR_43", "PAR_44", "PAR_45", "Einfahren_Piston", "PAR_47", "PAR_48", "PAR_49", "PAR_50", "PAR_51", "PAR_52", "PAR_53", "PAR_54", "PAR_55", "PAR_56", "PAR_57", "LinearUpDown_Button", "Linear_Pore_GO", "Linear_Axial_GO", "Linear_Side_GO", "PAR_62", "PAR_63", "PAR_64", "PAR_65", "PAR_66", "PAR_67", "PAR_68", "PAR_69", "Pre_Shearing_Button", "PAR_71", "PAR_72", "PAR_73", "PAR_74", "Circumf_Control_On", "PAR_76", "PAR_77", "PAR_78", "PAR_79", "Modus", "", "", "", "", "", "", "", "", "", "", "", "", "", "", "", "", "", "", "", "", "", "", "", "", "", ""] ("par_enum")
            w1155 = u16 61 items=["NaN", "Kp_Position_Vibro", "Ki_Position_Vibro", "PAR_3", "Sinusfrequenz_preSh", "Zylinder_Move_Button", "PAR_6", "PAR_7", "PAR_8", "PAR_9", "PAR_10", "PAR_11", "PAR_12", "Amplitude_PreSh", "Compass_OFF", "PAR_15", "PAR_16", "SollMoog", "PAR_18", "PAR_19", "PAR_20", "Vibro_Test_Button", "PAR_22", "PAR_23", "PAR_24", "PAR_25", "PAR_26", "PAR_27", "PAR_28", "PAR_29", "PAR_30", "PAR_31", "PAR_32", "Start_Test_Button", "PAR_34", "Programm_counter", "PAR_36", "Circumference_ON_Flag", "PAR_38", "PAR_39", "Pore_Control_Button", "Side_Control_Button", "Axial_Control_Button", "PAR_43", "PAR_44", "PAR_45", "Einfahren_Piston", "PAR_47", "PAR_48", "PAR_49", "PAR_50", "PAR_51", "PAR_52", "PAR_53", "PAR_54", "PAR_55", "PAR_56", "PAR_57", "LinearUpDown_Button", "Linear_Pore_GO", "Linear_Axial_GO", "Linear_Side_GO", "PAR_62", "PAR_63", "PAR_64", "PAR_65", "PAR_66", "PAR_67", "PAR_68", "PAR_69", "Pre_Shearing_Button", "PAR_71", "PAR_72", "PAR_73", "PAR_74", "Circumf_Control_On", "PAR_76", "PAR_77", "PAR_78", "PAR_79", "Modus", "", "", "", "", "", "", "", "", "", "", "", "", "", "", "", "", "", "", "", "", "", "", "", "", "", ""] ("par_enum")
            n710 = Select(t=1 ("Value"), s=w1146, f=0 ("Value")) -> (s? t:f=w1153:i32)
            n711 = Select(t=1 ("Value"), s=w1146, f=0 ("Value")) -> (s? t:f=w1150:i32)
            n712 = call "ADwin Set_Par.vi"("Value"=w1153, "Index"=w1155, "Device No."=w1151) -> ("Device No. out"=w1147:u16)  [unwired: 6 in, 2 out]
            n713 = call "ADwin Set_Par.vi"("Value"=w1150, "Index"=w1148, "Device No."=w1147) -> ()  [unwired: 6 in, 3 out]
          }
        }
      }
      event "Set auto file name": Value Change {
        n714 = event-data() -> ()  [unwired: 1 in, 6 out]
        n715 = local read "IS P-Value"() -> (w1188:i32)
        n716 = local read "IS I-Value"() -> (w1182:i32)
        n717 = local read "Feeding IS"() -> (w1179:dbl)
        n718 = local read "Amplitude IS"() -> (w1174:dbl)
        n719 = local read "Frequency IS"() -> (w1170:dbl)
        n720 = Number To Decimal String(number=w1174) -> (decimal integer string=w1176:string)  [unwired: 1 in]
        n721 = Number To Decimal String(number=w1170) -> (decimal integer string=w1172:string)  [unwired: 1 in]
        n722 = Number To Decimal String(number=w1179) -> (decimal integer string=w1180:string)  [unwired: 1 in]
        n723 = Number To Decimal String(number=w1182) -> (decimal integer string=w1184:string)  [unwired: 1 in]
        n724 = Number To Decimal String(number=w1188) -> (decimal integer string=w1187:string)  [unwired: 1 in]
        n725 = Concatenate Strings("_A" ("string"), w1176) -> (w1173:string)
        n726 = Concatenate Strings("_F" ("string"), w1172) -> (w1169:string)
        n727 = Concatenate Strings("_V" ("string"), w1180) -> (w1177:string)
        n728 = Concatenate Strings("_I" ("string"), w1184) -> (w1181:string)
        n729 = Concatenate Strings("P" ("string"), w1187) -> (w1185:string)
        n730 = Format Date/Time String(time format string (%c)="%d_%m_%y_%H_%M_") -> (date/time string=w1189:string)  [unwired: 2 in]
        n731 = Current VI's Path() -> (path=w1159:path)
        n732 = Strip Path(path=w1159) -> (stripped path=w1158:path)  [unwired: 1 out]
        n733 = Concatenate Strings(w1189, w1185, w1181, w1177, w1173, w1169, ".csv" ("String")) -> (w1165:string)
        n734 = Build Path(base path=w1158, name or relative path=w1156) -> (appended path=w1160:path)
        n735 = String To Path(string=w1165) -> (path=w1166:path)
        n736 = Build Path(base path=w1164, name or relative path=w1166) -> (appended path=w1163:path)
        n737 = call-poly <vilib>:"Read From Spreadsheet File.vi"("delimiter (\\t)"=";" ("delimiter (\\t)"), "file path (dialog if empty)"=w1160) -> ("first row"=w1157:string[])  [unwired: 5 in, 4 out]
        n738 = local write "Path Logging"(w1163) -> ()
        n739 = call-poly <vilib>:"Write To Spreadsheet File.vi"("delimiter (\\t)"=";" ("delimiter (\\t)"), "1D data"=w1157, "file path (dialog if empty)"=w1163) -> ()  [unwired: 5 in, 1 out]
      }
      event "SET P/I Value": Value Change {
        w1191 = u16 1 items=["NaN", "Kp_Position_Vibro", "Ki_Position_Vibro", "PAR_3", "Sinusfrequenz_preSh", "Zylinder_Move_Button", "PAR_6", "PAR_7", "PAR_8", "PAR_9", "PAR_10", "PAR_11", "PAR_12", "Amplitude_PreSh", "Compass_OFF", "PAR_15", "PAR_16", "SollMoog", "PAR_18", "PAR_19", "PAR_20", "Vibro_Test_Button", "PAR_22", "PAR_23", "PAR_24", "PAR_25", "PAR_26", "PAR_27", "PAR_28", "PAR_29", "PAR_30", "PAR_31", "PAR_32", "Start_Test_Button", "PAR_34", "Programm_counter", "PAR_36", "Circumference_ON_Flag", "PAR_38", "PAR_39", "Pore_Control_Button", "Side_Control_Button", "Axial_Control_Button", "PAR_43", "PAR_44", "PAR_45", "Einfahren_Piston", "PAR_47", "PAR_48", "PAR_49", "PAR_50", "PAR_51", "PAR_52", "PAR_53", "PAR_54", "PAR_55", "PAR_56", "PAR_57", "LinearUpDown_Button", "Linear_Pore_GO", "Linear_Axial_GO", "Linear_Side_GO", "PAR_62", "PAR_63", "PAR_64", "PAR_65", "PAR_66", "PAR_67", "PAR_68", "PAR_69", "Pre_Shearing_Button", "PAR_71", "PAR_72", "PAR_73", "PAR_74", "Circumf_Control_On", "PAR_76", "PAR_77", "PAR_78", "PAR_79", "Modus", "", "", "", "", "", "", "", "", "", "", "", "", "", "", "", "", "", "", "", "", "", "", "", "", "", ""] ("par_enum")
        w1190 = u16 2 items=["NaN", "Kp_Position_Vibro", "Ki_Position_Vibro", "PAR_3", "Sinusfrequenz_preSh", "Zylinder_Move_Button", "PAR_6", "PAR_7", "PAR_8", "PAR_9", "PAR_10", "PAR_11", "PAR_12", "Amplitude_PreSh", "Compass_OFF", "PAR_15", "PAR_16", "SollMoog", "PAR_18", "PAR_19", "PAR_20", "Vibro_Test_Button", "PAR_22", "PAR_23", "PAR_24", "PAR_25", "PAR_26", "PAR_27", "PAR_28", "PAR_29", "PAR_30", "PAR_31", "PAR_32", "Start_Test_Button", "PAR_34", "Programm_counter", "PAR_36", "Circumference_ON_Flag", "PAR_38", "PAR_39", "Pore_Control_Button", "Side_Control_Button", "Axial_Control_Button", "PAR_43", "PAR_44", "PAR_45", "Einfahren_Piston", "PAR_47", "PAR_48", "PAR_49", "PAR_50", "PAR_51", "PAR_52", "PAR_53", "PAR_54", "PAR_55", "PAR_56", "PAR_57", "LinearUpDown_Button", "Linear_Pore_GO", "Linear_Axial_GO", "Linear_Side_GO", "PAR_62", "PAR_63", "PAR_64", "PAR_65", "PAR_66", "PAR_67", "PAR_68", "PAR_69", "Pre_Shearing_Button", "PAR_71", "PAR_72", "PAR_73", "PAR_74", "Circumf_Control_On", "PAR_76", "PAR_77", "PAR_78", "PAR_79", "Modus", "", "", "", "", "", "", "", "", "", "", "", "", "", "", "", "", "", "", "", "", "", "", "", "", "", ""] ("par_enum")
        n740 = event-data() -> ()  [unwired: 1 in, 6 out]
        n741 = call "ADwin Set_Par.vi"("Value"="Soll P-Value", "Index"=w1191, "Device No."=w1194) -> ("Device No. out"=w1192:u16)  [unwired: 6 in, 2 out]
        n742 = call "ADwin Set_Par.vi"("Value"="Soll I-Value", "Index"=w1190, "Device No."=w1192) -> ()  [unwired: 6 in, 3 out]
      }
      event "Set New Path": Value Change {
        n743 = event-data() -> ("NewVal"=w1199:bool)  [unwired: 1 in, 5 out]
        n744 = String Length(string="New Path") -> (length=w1202:i32)
        n745 = Greater?(x=w1202, y=0) -> (0:w1200:bool)
        n746 = And(x=w1199, y=w1200) -> (x .and. y?=w1198:bool)
        n747 = case shown="True" w1198 {
          tunnel: w1203 -> [_ w1215]
          tunnel: "New Path" -> [_ w1214]
          tunnel: w1196 -> [_ w1206]
          frame False {
          }
          frame True {
            n748 = Current VI's Path() -> (path=w1211:path)
            n749 = Format Date/Time String(time format string (%c)="%d_%m_%y_%H_%M_") -> (date/time string=w1204:string)  [unwired: 2 in]
            n750 = Strip Path(path=w1211) -> (stripped path=w1210:path)  [unwired: 1 out]
            n751 = Build Path(base path=w1210, name or relative path=w1206) -> (appended path=w1212:path)
            n752 = Concatenate Strings(w1204, w1214, ".csv" ("String")) -> (w1216:string)
            n753 = Build Path(base path=w1215, name or relative path=w1216) -> (appended path=w1207:path)
            n754 = call-poly <vilib>:"Read From Spreadsheet File.vi"("delimiter (\\t)"=";" ("delimiter (\\t)"), "file path (dialog if empty)"=w1212) -> ("first row"=w1208:string[])  [unwired: 5 in, 4 out]
            n755 = call-poly <vilib>:"Write To Spreadsheet File.vi"("delimiter (\\t)"=";" ("delimiter (\\t)"), "1D data"=w1208, "file path (dialog if empty)"=w1207) -> ()  [unwired: 5 in, 1 out]
            n756 = local write "Path Logging"(w1207) -> ()
          }
        }
      }
      event "Activate Manuel Control": Value Change {
        n757 = event-data() -> ("NewVal"=w1218:bool)  [unwired: 1 in, 5 out]
        "Manuel Control" <- w1218
        n758 = case shown="False" w1218 {
          tunnel: w1221 -> [_ w1225]
          frame False {
          }
          frame True {
            w1222 = u16 80 items=["NaN", "Kp_Position_Vibro", "Ki_Position_Vibro", "PAR_3", "Sinusfrequenz_preSh", "Zylinder_Move_Button", "PAR_6", "PAR_7", "PAR_8", "PAR_9", "PAR_10", "PAR_11", "PAR_12", "Amplitude_PreSh", "Compass_OFF", "PAR_15", "PAR_16", "SollMoog", "PAR_18", "PAR_19", "PAR_20", "Vibro_Test_Button", "PAR_22", "PAR_23", "PAR_24", "PAR_25", "PAR_26", "PAR_27", "PAR_28", "PAR_29", "PAR_30", "PAR_31", "PAR_32", "Start_Test_Button", "PAR_34", "Programm_counter", "PAR_36", "Circumference_ON_Flag", "PAR_38", "PAR_39", "Pore_Control_Button", "Side_Control_Button", "Axial_Control_Button", "PAR_43", "PAR_44", "PAR_45", "Einfahren_Piston", "PAR_47", "PAR_48", "PAR_49", "PAR_50", "PAR_51", "PAR_52", "PAR_53", "PAR_54", "PAR_55", "PAR_56", "PAR_57", "LinearUpDown_Button", "Linear_Pore_GO", "Linear_Axial_GO", "Linear_Side_GO", "PAR_62", "PAR_63", "PAR_64", "PAR_65", "PAR_66", "PAR_67", "PAR_68", "PAR_69", "Pre_Shearing_Button", "PAR_71", "PAR_72", "PAR_73", "PAR_74", "Circumf_Control_On", "PAR_76", "PAR_77", "PAR_78", "PAR_79", "Modus", "", "", "", "", "", "", "", "", "", "", "", "", "", "", "", "", "", "", "", "", "", "", "", "", "", ""] ("par_enum")
            n759 = property on="Activate Pumps/Piston Controls" class="Bool (strict)"("DisabledEnum"=T6."Enabled" ("Disabled")) -> ()  [unwired: 2 in, 2 out]
            n760 = call "ADwin Set_Par.vi"("Value"=1, "Index"=w1222, "Device No."=w1225) -> ()  [unwired: 6 in, 3 out]
          }
        }
        n761 = local write "Activate Manuel Control"(TRUE ("Activate Manuel Control")) -> ()
        n762 = local write "Activate Pumps/Piston Controls"(FALSE ("Activate Controls")) -> ()
      }
      event "start penetration": Value Change {
        w1228 = u16 33 items=["NaN", "Kp_Position_Vibro", "Ki_Position_Vibro", "PAR_3", "Sinusfrequenz_preSh", "Zylinder_Move_Button", "PAR_6", "PAR_7", "PAR_8", "PAR_9", "PAR_10", "PAR_11", "PAR_12", "Amplitude_PreSh", "Compass_OFF", "PAR_15", "PAR_16", "SollMoog", "PAR_18", "PAR_19", "PAR_20", "Vibro_Test_Button", "PAR_22", "PAR_23", "PAR_24", "PAR_25", "PAR_26", "PAR_27", "PAR_28", "PAR_29", "PAR_30", "PAR_31", "PAR_32", "Start_Test_Button", "PAR_34", "Programm_counter", "PAR_36", "Circumference_ON_Flag", "PAR_38", "PAR_39", "Pore_Control_Button", "Side_Control_Button", "Axial_Control_Button", "PAR_43", "PAR_44", "PAR_45", "Einfahren_Piston", "PAR_47", "PAR_48", "PAR_49", "PAR_50", "PAR_51", "PAR_52", "PAR_53", "PAR_54", "PAR_55", "PAR_56", "PAR_57", "LinearUpDown_Button", "Linear_Pore_GO", "Linear_Axial_GO", "Linear_Side_GO", "PAR_62", "PAR_63", "PAR_64", "PAR_65", "PAR_66", "PAR_67", "PAR_68", "PAR_69", "Pre_Shearing_Button", "PAR_71", "PAR_72", "PAR_73", "PAR_74", "Circumf_Control_On", "PAR_76", "PAR_77", "PAR_78", "PAR_79", "Modus", "", "", "", "", "", "", "", "", "", "", "", "", "", "", "", "", "", "", "", "", "", "", "", "", "", ""] ("par_enum")
        n763 = event-data() -> ("NewVal"=w1227:bool)  [unwired: 1 in, 5 out]
        "Boolean" <- w1227
        "Penetration ongoing" <- w1227
        n764 = Wait (ms)(milliseconds to wait=u32 0) -> ()  [unwired: 1 out]
        n765 = case shown="True" w1227 {
          selector: w1227 -> [w1234 w1236]
          frame False {
            n766 = Not(x=w1234) -> (.not. x?=→"Test ended":bool)
          }
          frame True {
            n767 = property on="Pore Pressure okay:" class="Bool (strict)"("DisabledEnum"=T6."Enabled" ("Disabled")) -> ()  [unwired: 2 in, 2 out]
            n768 = property on="Side Pressure okay:" class="Bool (strict)"("DisabledEnum"=T6."Enabled" ("Disabled")) -> ()  [unwired: 2 in, 2 out]
            n769 = property on="Axial Pressure okay:" class="Bool (strict)"("DisabledEnum"=T6."Enabled" ("Disabled")) -> ()  [unwired: 2 in, 2 out]
            n770 = local write "Interner Kraftsensor [MPa]"(cluster{"Y":dbl[], "Y":dbl[]}[] [] ("Interner Kraftsensor [MPa]")) -> ()
            "Test Flag" <- w1236
            "Test Started" <- w1236
          }
        }
        n771 = local write "Record Data"(w1227) -> ()
        n772 = Select(t=1 ("Value"), s=w1227, f=0 ("Value")) -> (s? t:f=w1232:i32)
        n773 = call "ADwin Set_Par.vi"("Value"=w1232, "Index"=w1228, "Device No."=w1229) -> ()  [unwired: 6 in, 3 out]
      }
      event "SET Pre-Shearing": Value Change {
        w1240 = u16 4 items=["NaN", "Kp_Position_Vibro", "Ki_Position_Vibro", "PAR_3", "Sinusfrequenz_preSh", "Zylinder_Move_Button", "PAR_6", "PAR_7", "PAR_8", "PAR_9", "PAR_10", "PAR_11", "PAR_12", "Amplitude_PreSh", "Compass_OFF", "PAR_15", "PAR_16", "SollMoog", "PAR_18", "PAR_19", "PAR_20", "Vibro_Test_Button", "PAR_22", "PAR_23", "PAR_24", "PAR_25", "PAR_26", "PAR_27", "PAR_28", "PAR_29", "PAR_30", "PAR_31", "PAR_32", "Start_Test_Button", "PAR_34", "Programm_counter", "PAR_36", "Circumference_ON_Flag", "PAR_38", "PAR_39", "Pore_Control_Button", "Side_Control_Button", "Axial_Control_Button", "PAR_43", "PAR_44", "PAR_45", "Einfahren_Piston", "PAR_47", "PAR_48", "PAR_49", "PAR_50", "PAR_51", "PAR_52", "PAR_53", "PAR_54", "PAR_55", "PAR_56", "PAR_57", "LinearUpDown_Button", "Linear_Pore_GO", "Linear_Axial_GO", "Linear_Side_GO", "PAR_62", "PAR_63", "PAR_64", "PAR_65", "PAR_66", "PAR_67", "PAR_68", "PAR_69", "Pre_Shearing_Button", "PAR_71", "PAR_72", "PAR_73", "PAR_74", "Circumf_Control_On", "PAR_76", "PAR_77", "PAR_78", "PAR_79", "Modus", "", "", "", "", "", "", "", "", "", "", "", "", "", "", "", "", "", "", "", "", "", "", "", "", "", ""] ("par_enum")
        w1241 = u16 13 items=["NaN", "Kp_Position_Vibro", "Ki_Position_Vibro", "PAR_3", "Sinusfrequenz_preSh", "Zylinder_Move_Button", "PAR_6", "PAR_7", "PAR_8", "PAR_9", "PAR_10", "PAR_11", "PAR_12", "Amplitude_PreSh", "Compass_OFF", "PAR_15", "PAR_16", "SollMoog", "PAR_18", "PAR_19", "PAR_20", "Vibro_Test_Button", "PAR_22", "PAR_23", "PAR_24", "PAR_25", "PAR_26", "PAR_27", "PAR_28", "PAR_29", "PAR_30", "PAR_31", "PAR_32", "Start_Test_Button", "PAR_34", "Programm_counter", "PAR_36", "Circumference_ON_Flag", "PAR_38", "PAR_39", "Pore_Control_Button", "Side_Control_Button", "Axial_Control_Button", "PAR_43", "PAR_44", "PAR_45", "Einfahren_Piston", "PAR_47", "PAR_48", "PAR_49", "PAR_50", "PAR_51", "PAR_52", "PAR_53", "PAR_54", "PAR_55", "PAR_56", "PAR_57", "LinearUpDown_Button", "Linear_Pore_GO", "Linear_Axial_GO", "Linear_Side_GO", "PAR_62", "PAR_63", "PAR_64", "PAR_65", "PAR_66", "PAR_67", "PAR_68", "PAR_69", "Pre_Shearing_Button", "PAR_71", "PAR_72", "PAR_73", "PAR_74", "Circumf_Control_On", "PAR_76", "PAR_77", "PAR_78", "PAR_79", "Modus", "", "", "", "", "", "", "", "", "", "", "", "", "", "", "", "", "", "", "", "", "", "", "", "", "", ""] ("par_enum")
        n774 = event-data() -> ()  [unwired: 1 in, 6 out]
        n775 = expression code="65536/12000*x"("Amplitude Cycle SOLL") -> (w1245:i32)
        n776 = call "ADwin Set_Par.vi"("Value"=w1245, "Index"=w1241, "Device No."=w1243) -> ("Device No. out"=w1242:u16)  [unwired: 6 in, 2 out]
        n777 = call "ADwin Set_Par.vi"("Value"="Duration of Cycle SOLL", "Index"=w1240, "Device No."=w1242) -> ()  [unwired: 6 in, 3 out]
      }
      event "Start Pre-Shearing": Value Change {
        w1248 = u16 70 items=["NaN", "Kp_Position_Vibro", "Ki_Position_Vibro", "PAR_3", "Sinusfrequenz_preSh", "Zylinder_Move_Button", "PAR_6", "PAR_7", "PAR_8", "PAR_9", "PAR_10", "PAR_11", "PAR_12", "Amplitude_PreSh", "Compass_OFF", "PAR_15", "PAR_16", "SollMoog", "PAR_18", "PAR_19", "PAR_20", "Vibro_Test_Button", "PAR_22", "PAR_23", "PAR_24", "PAR_25", "PAR_26", "PAR_27", "PAR_28", "PAR_29", "PAR_30", "PAR_31", "PAR_32", "Start_Test_Button", "PAR_34", "Programm_counter", "PAR_36", "Circumference_ON_Flag", "PAR_38", "PAR_39", "Pore_Control_Button", "Side_Control_Button", "Axial_Control_Button", "PAR_43", "PAR_44", "PAR_45", "Einfahren_Piston", "PAR_47", "PAR_48", "PAR_49", "PAR_50", "PAR_51", "PAR_52", "PAR_53", "PAR_54", "PAR_55", "PAR_56", "PAR_57", "LinearUpDown_Button", "Linear_Pore_GO", "Linear_Axial_GO", "Linear_Side_GO", "PAR_62", "PAR_63", "PAR_64", "PAR_65", "PAR_66", "PAR_67", "PAR_68", "PAR_69", "Pre_Shearing_Button", "PAR_71", "PAR_72", "PAR_73", "PAR_74", "Circumf_Control_On", "PAR_76", "PAR_77", "PAR_78", "PAR_79", "Modus", "", "", "", "", "", "", "", "", "", "", "", "", "", "", "", "", "", "", "", "", "", "", "", "", "", ""] ("par_enum")
        n778 = event-data() -> ("NewVal"=w1249:bool)  [unwired: 1 in, 5 out]
        n779 = Select(t=1 ("Value"), s=w1249, f=0 ("Value")) -> (s? t:f=w1251:i32)
        n780 = call "ADwin Set_Par.vi"("Value"=w1251, "Index"=w1248, "Device No."=w1247) -> ()  [unwired: 6 in, 3 out]
      }
      event "Activate Pumps/Piston Controls": Value Change {
        n781 = event-data() -> ("NewVal"=w1254:bool)  [unwired: 1 in, 5 out]
        "Pump Control On" <- w1254
        n782 = case shown="True" w1254 {
          tunnel: w1257 -> [_ w1259]
          frame False {
          }
          frame True {
            w1258 = u16 80 items=["NaN", "Kp_Position_Vibro", "Ki_Position_Vibro", "PAR_3", "Sinusfrequenz_preSh", "Zylinder_Move_Button", "PAR_6", "PAR_7", "PAR_8", "PAR_9", "PAR_10", "PAR_11", "PAR_12", "Amplitude_PreSh", "Compass_OFF", "PAR_15", "PAR_16", "SollMoog", "PAR_18", "PAR_19", "PAR_20", "Vibro_Test_Button", "PAR_22", "PAR_23", "PAR_24", "PAR_25", "PAR_26", "PAR_27", "PAR_28", "PAR_29", "PAR_30", "PAR_31", "PAR_32", "Start_Test_Button", "PAR_34", "Programm_counter", "PAR_36", "Circumference_ON_Flag", "PAR_38", "PAR_39", "Pore_Control_Button", "Side_Control_Button", "Axial_Control_Button", "PAR_43", "PAR_44", "PAR_45", "Einfahren_Piston", "PAR_47", "PAR_48", "PAR_49", "PAR_50", "PAR_51", "PAR_52", "PAR_53", "PAR_54", "PAR_55", "PAR_56", "PAR_57", "LinearUpDown_Button", "Linear_Pore_GO", "Linear_Axial_GO", "Linear_Side_GO", "PAR_62", "PAR_63", "PAR_64", "PAR_65", "PAR_66", "PAR_67", "PAR_68", "PAR_69", "Pre_Shearing_Button", "PAR_71", "PAR_72", "PAR_73", "PAR_74", "Circumf_Control_On", "PAR_76", "PAR_77", "PAR_78", "PAR_79", "Modus", "", "", "", "", "", "", "", "", "", "", "", "", "", "", "", "", "", "", "", "", "", "", "", "", "", ""] ("par_enum")
            n783 = call "ADwin Set_Par.vi"("Value"=3, "Index"=w1258, "Device No."=w1259) -> ()  [unwired: 6 in, 3 out]
          }
        }
        n784 = local write "Manuel Control"(FALSE ("Manuel Control")) -> ()
        n785 = local write "Activate Manuel Control"(FALSE ("Activate Manuel Control")) -> ()
        n786 = local write "Activate Pumps/Piston Controls"(TRUE ("Activate Controls")) -> ()
      }
      event "Move": Value Change {
        w1261 = u16 17 items=["NaN", "Kp_Position_Vibro", "Ki_Position_Vibro", "PAR_3", "Sinusfrequenz_preSh", "Zylinder_Move_Button", "PAR_6", "PAR_7", "PAR_8", "PAR_9", "PAR_10", "PAR_11", "PAR_12", "Amplitude_PreSh", "Compass_OFF", "PAR_15", "PAR_16", "SollMoog", "PAR_18", "PAR_19", "PAR_20", "Vibro_Test_Button", "PAR_22", "PAR_23", "PAR_24", "PAR_25", "PAR_26", "PAR_27", "PAR_28", "PAR_29", "PAR_30", "PAR_31", "PAR_32", "Start_Test_Button", "PAR_34", "Programm_counter", "PAR_36", "Circumference_ON_Flag", "PAR_38", "PAR_39", "Pore_Control_Button", "Side_Control_Button", "Axial_Control_Button", "PAR_43", "PAR_44", "PAR_45", "Einfahren_Piston", "PAR_47", "PAR_48", "PAR_49", "PAR_50", "PAR_51", "PAR_52", "PAR_53", "PAR_54", "PAR_55", "PAR_56", "PAR_57", "LinearUpDown_Button", "Linear_Pore_GO", "Linear_Axial_GO", "Linear_Side_GO", "PAR_62", "PAR_63", "PAR_64", "PAR_65", "PAR_66", "PAR_67", "PAR_68", "PAR_69", "Pre_Shearing_Button", "PAR_71", "PAR_72", "PAR_73", "PAR_74", "Circumf_Control_On", "PAR_76", "PAR_77", "PAR_78", "PAR_79", "Modus", "", "", "", "", "", "", "", "", "", "", "", "", "", "", "", "", "", "", "", "", "", "", "", "", "", ""] ("par_enum")
        w1262 = u16 5 items=["NaN", "Kp_Position_Vibro", "Ki_Position_Vibro", "PAR_3", "Sinusfrequenz_preSh", "Zylinder_Move_Button", "PAR_6", "PAR_7", "PAR_8", "PAR_9", "PAR_10", "PAR_11", "PAR_12", "Amplitude_PreSh", "Compass_OFF", "PAR_15", "PAR_16", "SollMoog", "PAR_18", "PAR_19", "PAR_20", "Vibro_Test_Button", "PAR_22", "PAR_23", "PAR_24", "PAR_25", "PAR_26", "PAR_27", "PAR_28", "PAR_29", "PAR_30", "PAR_31", "PAR_32", "Start_Test_Button", "PAR_34", "Programm_counter", "PAR_36", "Circumference_ON_Flag", "PAR_38", "PAR_39", "Pore_Control_Button", "Side_Control_Button", "Axial_Control_Button", "PAR_43", "PAR_44", "PAR_45", "Einfahren_Piston", "PAR_47", "PAR_48", "PAR_49", "PAR_50", "PAR_51", "PAR_52", "PAR_53", "PAR_54", "PAR_55", "PAR_56", "PAR_57", "LinearUpDown_Button", "Linear_Pore_GO", "Linear_Axial_GO", "Linear_Side_GO", "PAR_62", "PAR_63", "PAR_64", "PAR_65", "PAR_66", "PAR_67", "PAR_68", "PAR_69", "Pre_Shearing_Button", "PAR_71", "PAR_72", "PAR_73", "PAR_74", "Circumf_Control_On", "PAR_76", "PAR_77", "PAR_78", "PAR_79", "Modus", "", "", "", "", "", "", "", "", "", "", "", "", "", "", "", "", "", "", "", "", "", "", "", "", "", ""] ("par_enum")
        n787 = event-data() -> ("NewVal"=w1271:bool)  [unwired: 1 in, 5 out]
        n788 = expression code="65336/10*x+32768"("Schieberegler") -> (w1264:dbl)
        n789 = Select(t=1 ("Value"), s=w1271, f=0 ("Value")) -> (s? t:f=w1268:i32)
        n790 = To Long Integer(number=w1264) -> (32bit integer=w1265:i32)
        n791 = call "ADwin Set_Par.vi"("Value"=w1268, "Index"=w1262, "Device No."=w1267) -> ("Device No. out"=w1266:u16)  [unwired: 6 in, 2 out]
        n792 = call "ADwin Set_Par.vi"("Value"=w1265, "Index"=w1261, "Device No."=w1266) -> ()  [unwired: 6 in, 3 out]
      }
      event "Regelung Akiv Porepress", "Regelung Akiv Sidepressure", "Regelung Akiv Axial": Value Change {
        w1274 = u16 42 items=["NaN", "Kp_Position_Vibro", "Ki_Position_Vibro", "PAR_3", "Sinusfrequenz_preSh", "Zylinder_Move_Button", "PAR_6", "PAR_7", "PAR_8", "PAR_9", "PAR_10", "PAR_11", "PAR_12", "Amplitude_PreSh", "Compass_OFF", "PAR_15", "PAR_16", "SollMoog", "PAR_18", "PAR_19", "PAR_20", "Vibro_Test_Button", "PAR_22", "PAR_23", "PAR_24", "PAR_25", "PAR_26", "PAR_27", "PAR_28", "PAR_29", "PAR_30", "PAR_31", "PAR_32", "Start_Test_Button", "PAR_34", "Programm_counter", "PAR_36", "Circumference_ON_Flag", "PAR_38", "PAR_39", "Pore_Control_Button", "Side_Control_Button", "Axial_Control_Button", "PAR_43", "PAR_44", "PAR_45", "Einfahren_Piston", "PAR_47", "PAR_48", "PAR_49", "PAR_50", "PAR_51", "PAR_52", "PAR_53", "PAR_54", "PAR_55", "PAR_56", "PAR_57", "LinearUpDown_Button", "Linear_Pore_GO", "Linear_Axial_GO", "Linear_Side_GO", "PAR_62", "PAR_63", "PAR_64", "PAR_65", "PAR_66", "PAR_67", "PAR_68", "PAR_69", "Pre_Shearing_Button", "PAR_71", "PAR_72", "PAR_73", "PAR_74", "Circumf_Control_On", "PAR_76", "PAR_77", "PAR_78", "PAR_79", "Modus", "", "", "", "", "", "", "", "", "", "", "", "", "", "", "", "", "", "", "", "", "", "", "", "", "", ""] ("par_enum")
        w1273 = u16 41 items=["NaN", "Kp_Position_Vibro", "Ki_Position_Vibro", "PAR_3", "Sinusfrequenz_preSh", "Zylinder_Move_Button", "PAR_6", "PAR_7", "PAR_8", "PAR_9", "PAR_10", "PAR_11", "PAR_12", "Amplitude_PreSh", "Compass_OFF", "PAR_15", "PAR_16", "SollMoog", "PAR_18", "PAR_19", "PAR_20", "Vibro_Test_Button", "PAR_22", "PAR_23", "PAR_24", "PAR_25", "PAR_26", "PAR_27", "PAR_28", "PAR_29", "PAR_30", "PAR_31", "PAR_32", "Start_Test_Button", "PAR_34", "Programm_counter", "PAR_36", "Circumference_ON_Flag", "PAR_38", "PAR_39", "Pore_Control_Button", "Side_Control_Button", "Axial_Control_Button", "PAR_43", "PAR_44", "PAR_45", "Einfahren_Piston", "PAR_47", "PAR_48", "PAR_49", "PAR_50", "PAR_51", "PAR_52", "PAR_53", "PAR_54", "PAR_55", "PAR_56", "PAR_57", "LinearUpDown_Button", "Linear_Pore_GO", "Linear_Axial_GO", "Linear_Side_GO", "PAR_62", "PAR_63", "PAR_64", "PAR_65", "PAR_66", "PAR_67", "PAR_68", "PAR_69", "Pre_Shearing_Button", "PAR_71", "PAR_72", "PAR_73", "PAR_74", "Circumf_Control_On", "PAR_76", "PAR_77", "PAR_78", "PAR_79", "Modus", "", "", "", "", "", "", "", "", "", "", "", "", "", "", "", "", "", "", "", "", "", "", "", "", "", ""] ("par_enum")
        w1272 = u16 40 items=["NaN", "Kp_Position_Vibro", "Ki_Position_Vibro", "PAR_3", "Sinusfrequenz_preSh", "Zylinder_Move_Button", "PAR_6", "PAR_7", "PAR_8", "PAR_9", "PAR_10", "PAR_11", "PAR_12", "Amplitude_PreSh", "Compass_OFF", "PAR_15", "PAR_16", "SollMoog", "PAR_18", "PAR_19", "PAR_20", "Vibro_Test_Button", "PAR_22", "PAR_23", "PAR_24", "PAR_25", "PAR_26", "PAR_27", "PAR_28", "PAR_29", "PAR_30", "PAR_31", "PAR_32", "Start_Test_Button", "PAR_34", "Programm_counter", "PAR_36", "Circumference_ON_Flag", "PAR_38", "PAR_39", "Pore_Control_Button", "Side_Control_Button", "Axial_Control_Button", "PAR_43", "PAR_44", "PAR_45", "Einfahren_Piston", "PAR_47", "PAR_48", "PAR_49", "PAR_50", "PAR_51", "PAR_52", "PAR_53", "PAR_54", "PAR_55", "PAR_56", "PAR_57", "LinearUpDown_Button", "Linear_Pore_GO", "Linear_Axial_GO", "Linear_Side_GO", "PAR_62", "PAR_63", "PAR_64", "PAR_65", "PAR_66", "PAR_67", "PAR_68", "PAR_69", "Pre_Shearing_Button", "PAR_71", "PAR_72", "PAR_73", "PAR_74", "Circumf_Control_On", "PAR_76", "PAR_77", "PAR_78", "PAR_79", "Modus", "", "", "", "", "", "", "", "", "", "", "", "", "", "", "", "", "", "", "", "", "", "", "", "", "", ""] ("par_enum")
        n793 = event-data() -> ()  [unwired: 1 in, 6 out]
        n794 = Select(t=1 ("Value"), s="Regelung Akiv Porepress", f=0 ("Value")) -> (s? t:f=w1277:i32)
        n795 = Select(t=1 ("Value"), s="Regelung Akiv Axial", f=0 ("Value")) -> (s? t:f=w1283:i32)
        n796 = Select(t=1 ("Value"), s="Regelung Akiv Sidepressure", f=0 ("Value")) -> (s? t:f=w1280:i32)
        n797 = call "ADwin Set_Par.vi"("Value"=w1277, "Index"=w1272, "Device No."=w1275) -> ("Device No. out"=w1288:u16)  [unwired: 6 in, 2 out]
        n798 = call "ADwin Set_Par.vi"("Value"=w1280, "Index"=w1273, "Device No."=w1288) -> ("Device No. out"=w1289:u16)  [unwired: 6 in, 2 out]
        n799 = call "ADwin Set_Par.vi"("Value"=w1283, "Index"=w1274, "Device No."=w1289) -> ()  [unwired: 6 in, 3 out]
      }
      event "SET Pump Pressures": Value Change {
        n800 = event-data() -> ()  [unwired: 1 in, 6 out]
        n801 = local read "Linear Control On"() -> (w1291:bool)
        n802 = Not(x=w1291) -> (.not. x?=w1290:bool)
        n803 = case shown="True" w1290 {
          tunnel: w1292 -> [_ w1304]
          frame False {
          }
          frame True {
            n804 = expression code="65536/12000*x+32768"("Soll Pore Pressure") -> (w1301:dbl)
            n805 = expression code="65536/12000*x+32768"("Soll Axial Pressure") -> (w1302:dbl)
            n806 = expression code="65536/12000*x+32768"("Soll Side Pressure") -> (w1303:dbl)
            n807 = To Single Precision Float(number=w1301) -> (single precision float=w1307:sgl)
            n808 = To Single Precision Float(number=w1302) -> (single precision float=w1306:sgl)
            n809 = To Single Precision Float(number=w1303) -> (single precision float=w1305:sgl)
            n810 = call "ADwin Set_FPar.vi"("Value"=w1307, "Index"=T10."Set_Soll_PorePressure" ("Enum"), "Device No."=w1304) -> ("Device No. out"=w1297:u16)  [unwired: 6 in, 2 out]
            n811 = call "ADwin Set_FPar.vi"("Value"=w1306, "Index"=T10."Set_Soll_AxialPressure" ("Enum"), "Device No."=w1297) -> ("Device No. out"=w1296:u16)  [unwired: 6 in, 2 out]
            n812 = call "ADwin Set_FPar.vi"("Value"=w1305, "Index"=T10."Set_Soll_SidePressure" ("Enum"), "Device No."=w1296) -> ()  [unwired: 6 in, 3 out]
          }
        }
      }
      event "SET Vibro Settings": Value Change {
        w1312 = u16 1 items=["NaN", "Kp_Position_Vibro", "Ki_Position_Vibro", "PAR_3", "Sinusfrequenz_preSh", "Zylinder_Move_Button", "PAR_6", "PAR_7", "PAR_8", "PAR_9", "PAR_10", "PAR_11", "PAR_12", "Amplitude_PreSh", "Compass_OFF", "PAR_15", "PAR_16", "SollMoog", "PAR_18", "PAR_19", "PAR_20", "Vibro_Test_Button", "PAR_22", "PAR_23", "PAR_24", "PAR_25", "PAR_26", "PAR_27", "PAR_28", "PAR_29", "PAR_30", "PAR_31", "PAR_32", "Start_Test_Button", "PAR_34", "Programm_counter", "PAR_36", "Circumference_ON_Flag", "PAR_38", "PAR_39", "Pore_Control_Button", "Side_Control_Button", "Axial_Control_Button", "PAR_43", "PAR_44", "PAR_45", "Einfahren_Piston", "PAR_47", "PAR_48", "PAR_49", "PAR_50", "PAR_51", "PAR_52", "PAR_53", "PAR_54", "PAR_55", "PAR_56", "PAR_57", "LinearUpDown_Button", "Linear_Pore_GO", "Linear_Axial_GO", "Linear_Side_GO", "PAR_62", "PAR_63", "PAR_64", "PAR_65", "PAR_66", "PAR_67", "PAR_68", "PAR_69", "Pre_Shearing_Button", "PAR_71", "PAR_72", "PAR_73", "PAR_74", "Circumf_Control_On", "PAR_76", "PAR_77", "PAR_78", "PAR_79", "Modus", "", "", "", "", "", "", "", "", "", "", "", "", "", "", "", "", "", "", "", "", "", "", "", "", "", ""] ("par_enum")
        w1313 = u16 2 items=["NaN", "Kp_Position_Vibro", "Ki_Position_Vibro", "PAR_3", "Sinusfrequenz_preSh", "Zylinder_Move_Button", "PAR_6", "PAR_7", "PAR_8", "PAR_9", "PAR_10", "PAR_11", "PAR_12", "Amplitude_PreSh", "Compass_OFF", "PAR_15", "PAR_16", "SollMoog", "PAR_18", "PAR_19", "PAR_20", "Vibro_Test_Button", "PAR_22", "PAR_23", "PAR_24", "PAR_25", "PAR_26", "PAR_27", "PAR_28", "PAR_29", "PAR_30", "PAR_31", "PAR_32", "Start_Test_Button", "PAR_34", "Programm_counter", "PAR_36", "Circumference_ON_Flag", "PAR_38", "PAR_39", "Pore_Control_Button", "Side_Control_Button", "Axial_Control_Button", "PAR_43", "PAR_44", "PAR_45", "Einfahren_Piston", "PAR_47", "PAR_48", "PAR_49", "PAR_50", "PAR_51", "PAR_52", "PAR_53", "PAR_54", "PAR_55", "PAR_56", "PAR_57", "LinearUpDown_Button", "Linear_Pore_GO", "Linear_Axial_GO", "Linear_Side_GO", "PAR_62", "PAR_63", "PAR_64", "PAR_65", "PAR_66", "PAR_67", "PAR_68", "PAR_69", "Pre_Shearing_Button", "PAR_71", "PAR_72", "PAR_73", "PAR_74", "Circumf_Control_On", "PAR_76", "PAR_77", "PAR_78", "PAR_79", "Modus", "", "", "", "", "", "", "", "", "", "", "", "", "", "", "", "", "", "", "", "", "", "", "", "", "", ""] ("par_enum")
        w1320 = u16 21 items=["NaN", "Kp_Position_Vibro", "Ki_Position_Vibro", "PAR_3", "Sinusfrequenz_preSh", "Zylinder_Move_Button", "PAR_6", "PAR_7", "PAR_8", "PAR_9", "PAR_10", "PAR_11", "PAR_12", "Amplitude_PreSh", "Compass_OFF", "PAR_15", "PAR_16", "SollMoog", "PAR_18", "PAR_19", "PAR_20", "Vibro_Test_Button", "PAR_22", "PAR_23", "PAR_24", "PAR_25", "PAR_26", "PAR_27", "PAR_28", "PAR_29", "PAR_30", "PAR_31", "PAR_32", "Start_Test_Button", "PAR_34", "Programm_counter", "PAR_36", "Circumference_ON_Flag", "PAR_38", "PAR_39", "Pore_Control_Button", "Side_Control_Button", "Axial_Control_Button", "PAR_43", "PAR_44", "PAR_45", "Einfahren_Piston", "PAR_47", "PAR_48", "PAR_49", "PAR_50", "PAR_51", "PAR_52", "PAR_53", "PAR_54", "PAR_55", "PAR_56", "PAR_57", "LinearUpDown_Button", "Linear_Pore_GO", "Linear_Axial_GO", "Linear_Side_GO", "PAR_62", "PAR_63", "PAR_64", "PAR_65", "PAR_66", "PAR_67", "PAR_68", "PAR_69", "Pre_Shearing_Button", "PAR_71", "PAR_72", "PAR_73", "PAR_74", "Circumf_Control_On", "PAR_76", "PAR_77", "PAR_78", "PAR_79", "Modus", "", "", "", "", "", "", "", "", "", "", "", "", "", "", "", "", "", "", "", "", "", "", "", "", "", ""] ("par_enum")
        # "Change Control Parameter to adjust to static and vibro control,\n for smoother control"
        n813 = event-data() -> ()  [unwired: 1 in, 6 out]
        n814 = Multiply(x="Vorschub SOLL", y=78.01) -> (x*y=w1318:dbl)
        n815 = Divide(x=w1318, y=5000.0) -> (x/y=w1317:dbl)
        n816 = expression code="1/x"("Frequency SOLL") -> (w1327:dbl)
        n817 = expression code="x*78"("Amplitude SOLL") -> (w1326:dbl)
        n818 = To Single Precision Float(number=w1317) -> (single precision float=w1331:sgl)
        n819 = To Single Precision Float(number=w1327) -> (single precision float=w1328:sgl)
        n820 = To Single Precision Float(number=w1326) -> (single precision float=w1325:sgl)
        n821 = Select(t=1 ("Value"), s="VibroTest", f=0 ("Value")) -> (s? t:f=w1335:i32)
        n822 = case shown="False" "VibroTest" {
          tunnel: [50 ("Value") 150 ("Value")] -> w1309
          tunnel: [0 ("Value") 10 ("Value")] -> w1308
          frame False {
          }
          frame True {
          }
        }
        n823 = call "ADwin Set_FPar.vi"("Value"=w1328, "Index"=T10."Sinusfrequenz_Vibro" ("Enum"), "Device No."=w1332) -> ("Device No. out"=w1330:u16)  [unwired: 6 in, 2 out]
        n824 = call "ADwin Set_FPar.vi"("Value"=w1331, "Index"=T10."Vorschub" ("Enum"), "Device No."=w1330) -> ("Device No. out"=w1329:u16)  [unwired: 6 in, 2 out]
        n825 = call "ADwin Set_FPar.vi"("Value"=w1325, "Index"=T10."Amplitude_Vibro" ("Enum"), "Device No."=w1329) -> ("Device No. out"=w1324:u16)  [unwired: 6 in, 2 out]
        n826 = call "ADwin Set_Par.vi"("Value"=w1335, "Index"=w1320, "Device No."=w1324) -> ("Device No. out"=w1310:u16)  [unwired: 6 in, 2 out]
        n827 = call "ADwin Set_Par.vi"("Value"=w1309, "Index"=w1312, "Device No."=w1310) -> ("Device No. out"=w1311:u16)  [unwired: 6 in, 2 out]
        n828 = call "ADwin Set_Par.vi"("Value"=w1308, "Index"=w1313, "Device No."=w1311) -> ()  [unwired: 6 in, 3 out]
      }
      event "SET Huang Su": Value Change {
        n829 = event-data() -> ()  [unwired: 1 in, 6 out]
        n830 = call "ADwin Set_FPar.vi"("Value"="SOLL Parameter 1", "Index"=T10."Huang_Su_par_1" ("Enum"), "Device No."=w1355) -> ("Device No. out"=w1342:u16)  [unwired: 6 in, 2 out]
        n831 = call "ADwin Set_FPar.vi"("Value"="SOLL Paramter 2", "Index"=T10."Huang_Su_par_2" ("Enum"), "Device No."=w1342) -> ("Device No. out"=w1354:u16)  [unwired: 6 in, 2 out]
        n832 = call "ADwin Set_FPar.vi"("Value"="SOLL Parameter 3", "Index"=T10."Huang_Su_par_3" ("Enum"), "Device No."=w1354) -> ("Device No. out"=w1353:u16)  [unwired: 6 in, 2 out]
        n833 = call "ADwin Set_FPar.vi"("Value"="SOLL Parameter 4", "Index"=T10."Huang_Su_par_4" ("Enum"), "Device No."=w1353) -> ("Device No. out"=w1352:u16)  [unwired: 6 in, 2 out]
        n834 = call "ADwin Set_FPar.vi"("Value"="SOLL Parameter 5", "Index"=T10."Huang_Su_par_5" ("Enum"), "Device No."=w1352) -> ("Device No. out"=w1351:u16)  [unwired: 6 in, 2 out]
        n835 = call "ADwin Set_FPar.vi"("Value"="SOLL Parameter 6", "Index"=T10."Huang_Su_par_6" ("Enum"), "Device No."=w1351) -> ("Device No. out"=w1350:u16)  [unwired: 6 in, 2 out]
        n836 = call "ADwin Set_FPar.vi"("Value"="SOLL Parameter 7", "Index"=T10."Huang_Su_par_7" ("Enum"), "Device No."=w1350) -> ()  [unwired: 6 in, 3 out]
      }
      event "Set button": Value Change {
        n837 = event-data() -> ()  [unwired: 1 in, 6 out]
        n838 = call "ADwin Get_FPar_Block.vi"("count"=i16 80, "startindex"=i16 1, "Device No."=w1365) -> ("Data"=w1363:sgl[], "Device No. out"=w1364:u16)  [unwired: 2 in, 2 out]
        n839 = case shown="True" "Set button" {
          tunnel: w1364 -> [_ w1369]
          tunnel: w1363 -> [_ w1371]
          frame False {
          }
          frame True {
            (unwired) "Standard value for Intercept"
            (unwired) "Standard value for slope"
            n840 = Decrement(x=T9."Slope_calibration" ("Enum")) -> (x-1=w1378:T9)
            n841 = Decrement(x=T9."Intercept_calibration" ("Enum")) -> (x-1=w1373:T9)
            n842 = Index Array(array=w1371, index=w1378) -> (element=w1374:sgl)
            n843 = Equal?(x=w1374, y="Soll Slope-Strain") -> (x = y?=w1375:bool)
            n844 = case shown="True" w1375 {
              tunnel: "Soll Slope-Strain" -> [w1387 _]
              tunnel: [w1387 w1388] -> w1382
              tunnel: w1374 -> [_ w1388]
              frame False {
              }
              frame True {
              }
            }
            n845 = Index Array(array=w1371, index=w1373) -> (element=w1370:sgl)
            n846 = Equal?(x="Soll Intercept-strain", y=w1370) -> (x = y?=w1381:bool)
            n847 = case shown="True" w1381 {
              tunnel: "Soll Intercept-strain" -> [w1385 _]
              tunnel: [w1385 w1386] -> w1379
              tunnel: w1370 -> [_ w1386]
              frame False {
              }
              frame True {
              }
            }
            n848 = call "ADwin Set_FPar.vi"("Value"=w1382, "Index"=T10."FPAR_18" ("Enum"), "Device No."=w1369) -> ()  [unwired: 6 in, 3 out]
            n849 = call "ADwin Set_FPar.vi"("Value"=w1379, "Index"=T10."FPAR_19" ("Enum"), "Device No."=w1369) -> ()  [unwired: 6 in, 3 out]
          }
        }
      }
      event "Huang Su Calibration File": Value Change {
        n850 = event-data() -> ("NewVal"=w1413:path)  [unwired: 1 in, 5 out]
        n851 = call-poly <vilib>:"Read Delimited Spreadsheet.vi"("file path (dialog if empty)"=w1413) -> ("all rows"=w1397:dbl[][])  [unwired: 9 in, 5 out]
        n852 = Index Array(array=w1397, index (row)=0, index (col)=0 ("disabled index (col)")) -> (element=w1396:dbl)
        n853 = Index Array(array=w1397, index (row)=1, index (col)=0 ("disabled index (col)")) -> (element=w1395:dbl)
        n854 = Index Array(array=w1397, index (row)=4, index (col)=0 ("disabled index (col)")) -> (element=w1392:dbl)
        n855 = Index Array(array=w1397, index (row)=3, index (col)=0 ("disabled index (col)")) -> (element=w1393:dbl)
        n856 = Index Array(array=w1397, index (row)=5, index (col)=0 ("disabled index (col)")) -> (element=w1391:dbl)
        n857 = Index Array(array=w1397, index (row)=2, index (col)=0 ("disabled index (col)")) -> (element=w1394:dbl)
        n858 = Index Array(array=w1397, index (row)=6, index (col)=0 ("disabled index (col)")) -> (element=w1390:dbl)
        n859 = local write "SOLL Parameter 4"(w1393) -> ()
        n860 = local write "SOLL Parameter 5"(w1392) -> ()
        n861 = local write "SOLL Parameter 6"(w1391) -> ()
        n862 = local write "SOLL Parameter 1"(w1396) -> ()
        n863 = local write "SOLL Parameter 3"(w1394) -> ()
        n864 = local write "SOLL Parameter 7"(w1390) -> ()
        n865 = local write "SOLL Paramter 2"(w1395) -> ()
        n866 = call "ADwin Set_FPar.vi"("Value"=w1396, "Index"=T10."Huang_Su_par_1" ("Enum"), "Device No."=w1410) -> ("Device No. out"=w1389:u16)  [unwired: 6 in, 2 out]
        n867 = call "ADwin Set_FPar.vi"("Value"=w1395, "Index"=T10."Huang_Su_par_2" ("Enum"), "Device No."=w1389) -> ("Device No. out"=w1425:u16)  [unwired: 6 in, 2 out]
        n868 = call "ADwin Set_FPar.vi"("Value"=w1394, "Index"=T10."Huang_Su_par_3" ("Enum"), "Device No."=w1425) -> ("Device No. out"=w1424:u16)  [unwired: 6 in, 2 out]
        n869 = call "ADwin Set_FPar.vi"("Value"=w1393, "Index"=T10."Huang_Su_par_4" ("Enum"), "Device No."=w1424) -> ("Device No. out"=w1423:u16)  [unwired: 6 in, 2 out]
        n870 = call "ADwin Set_FPar.vi"("Value"=w1392, "Index"=T10."Huang_Su_par_5" ("Enum"), "Device No."=w1423) -> ("Device No. out"=w1422:u16)  [unwired: 6 in, 2 out]
        n871 = call "ADwin Set_FPar.vi"("Value"=w1391, "Index"=T10."Huang_Su_par_6" ("Enum"), "Device No."=w1422) -> ("Device No. out"=w1421:u16)  [unwired: 6 in, 2 out]
        n872 = call "ADwin Set_FPar.vi"("Value"=w1390, "Index"=T10."Huang_Su_par_7" ("Enum"), "Device No."=w1421) -> ()  [unwired: 6 in, 3 out]
      }
    }
    n873 = Tick Count (ms)() -> (millisecond timer value=w42:u32)
    n874 = Subtract(x=w42, y=w44) -> (x-y=→"Time Loop":u32)
  }
